vi "stationary_v5_parallel_dragonfly.vi"() -> ()   [LabVIEW 2020]
uses:
  CUSTOM_CONTROLS/Liquid_Handler_Enum_NSE.ctl
  CUSTOM_CONTROLS/Transport_to_Reactor_Enum_NSE.ctl
  CUSTOM_CONTROLS/Transport_to_Analysis_Enum_NSE.ctl
  CUSTOM_CONTROLS/Rinse_Vent_Reactor_Enum_NSE.ctl
  CUSTOM_CONTROLS/Rinse_Vent_Transfer_Lines_Enum_NSE - Copy.ctl
  CUSTOM_CONTROLS/Hardware_Initiation_Enum.ctl
  CUSTOM_CONTROLS/Reactor_Outer_Loop_Enum_NSE.ctl
  CUSTOM_CONTROLS/Reactors_Enum_NSE.ctl
  <vilib>/DAQmx/read.llb/DAQmx Read (Analog 1D Wfm NChan 1Samp).vi
  <vilib>/DAQmx/miscellaneous.llb/DAQmx Fill In Error Info.vi
  HARVARD/LIBRARY_CC/Harvard Apparatus PHD Ultra Series.lvlib
panel:
  out "Schedule - Reactor to Analysis":dbl[](array[numeric])=[2556.0, 3156.0]
  out "Schedule - Liquid Handler":dbl[](array[numeric])=[1.0, 601.0]
  out "IndexTemp":dbl
  out "InitializationExp":bool
  out "IndexAct":dbl
  out "NextAnaTimeTrigger":dbl
  out "Index_Ana_Rxn":dbl
  out "Converged?":bool
  in  "Array 3":dbl[](array[numeric])
  in  "Convergence criterion (area counts)":dbl=-10.0
  out "Full Results":dbl[](array[numeric])
  out "Optimum":dbl[](array[numeric])=[50.17167959931792, 8.535205424923882, 2.0, 1.0, 39.0]
  in  "Array 2":dbl[](array[numeric])
  in  "Array":dbl[][](array[numeric])
  out "Next batch":dbl[][](array[numeric])=[[75.0, 32.5, 2.0, 2.0], [75.0, 32.5, 2.0, 2.0]]
  out "Batch Results":dbl[](array[numeric])
  in  "Batch size":i32=4
  in  "Number of initial experiments":i32=5
  out "Product area":dbl
  out "schedule_reset":bool
  out "product_area":dbl=1000000000000000.0
  out "analysis_finished":bool
  out "Next analysis time":dbl=1000000000000000.0
  out "reactor_to_analysis_finished":bool
  out "loop_to_reactor_finished":bool
  out "rinse_reactor_finished":bool
  out "rinse_transfer_lines_finished":bool
  out "liquid_handler_finished":bool
  out "Temperature - Reactor 10":dbl format="%#_3g"
  out "Temperature - Reactor 9":dbl format="%#_3g"
  out "Temperature - Reactor 8":dbl format="%#_3g"
  out "Temperature - Reactor 7":dbl format="%#_3g"
  out "Temperature - Reactor 6":dbl format="%#_3g"
  out "Temperature - Reactor 5":dbl format="%#_3g"
  out "Temperature - Reactor 4":dbl format="%#_3g"
  out "Temperature - Reactor 3":dbl format="%#_3g"
  out "Temperature - Reactor 2":dbl format="%#_3g"
  out "Temperature - Reactor 1":dbl
  out "Relay output DAQ error":bool
  out "Slug preparation error":bool
  out "Reaction scheduling error":bool
  out "Slug composition error":bool
  out "Analog input DAQ error":bool
  out "Reagent table parsing error":bool
  out "Data processing output":string
  out "Analysis Error":errorcluster
  out "Performing Optimization?":bool
  out "Shutdown complete":bool
  out "reaction scheduling error":errorcluster
  out "Analog input 3":waveform(dbl)[](graph)=[{"t0"=timestamp(3735667643.042628 s since 1904-01-01), "dt"=1.0, "Y"=[1.5884301073614158], "attributes"=variant("NI_ChannelName"=variant(string "NI9205"), "NI_UnitDescription"=variant(string "Volts"))}, {"t0"=timestamp(3735667643.0426416 s since 1904-01-01), "dt"=1.0, "Y"=[2.7564288374126047], "attributes"=variant("NI_ChannelName"=variant(string "NI9206"), "NI_UnitDescription"=variant(string "Volts"))}, {"t0"=timestamp(3735667643.042656 s since 1904-01-01), "dt"=1.0, "Y"=[0.0967580440506516], "attributes"=variant("NI_ChannelName"=variant(string "NI9207"), "NI_UnitDescription"=variant(string "Volts"))}, {"t0"=timestamp(3735667643.04267 s since 1904-01-01), "dt"=1.0, "Y"=[2.2988144683350704], "attributes"=variant("NI_ChannelName"=variant(string "NI9208"), "NI_UnitDescription"=variant(string "Volts"))}, {"t0"=timestamp(3735667643.042684 s since 1904-01-01), "dt"=1.0, "Y"=[0.5635616561855846], "attributes"=variant("NI_ChannelName"=variant(string "NI9209"), "NI_UnitDescription"=variant(string "Volts"))}, {"t0"=timestamp(3735667643.042698 s since 1904-01-01), "dt"=1.0, "Y"=[2.4613101697855475], "attributes"=variant("NI_ChannelName"=variant(string "NI9210"), "NI_UnitDescription"=variant(string "Volts"))}, {"t0"=timestamp(3735667643.0427117 s since 1904-01-01), "dt"=1.0, "Y"=[0.03569936837913687], "attributes"=variant("NI_ChannelName"=variant(string "NI9211"), "NI_UnitDescription"=variant(string "Volts"))}, {"t0"=timestamp(3735667643.042726 s since 1904-01-01), "dt"=1.0, "Y"=[2.0184685330254633], "attributes"=variant("NI_ChannelName"=variant(string "NI9212"), "NI_UnitDescription"=variant(string "Volts"))}, {"t0"=timestamp(3735667643.04274 s since 1904-01-01), "dt"=1.0, "Y"=[-8.232623427411115e-05], "attributes"=variant("NI_ChannelName"=variant(string "NI9213"), "NI_UnitDescription"=variant(string "Volts"))}, {"t0"=timestamp(3735667643.0427537 s since 1904-01-01), "dt"=1.0, "Y"=[0.0002459461853764819], "attributes"=variant("NI_ChannelName"=variant(string "NI9214"), "NI_UnitDescription"=variant(string "Volts"))}, {"t0"=timestamp(3735667643.042768 s since 1904-01-01), "dt"=1.0, "Y"=[-8.232623427411115e-05], "attributes"=variant("NI_ChannelName"=variant(string "NI9215"), "NI_UnitDescription"=variant(string "Volts"))}, {"t0"=timestamp(3735667643.042782 s since 1904-01-01), "dt"=1.0, "Y"=[-0.00041059865377756494], "attributes"=variant("NI_ChannelName"=variant(string "NI9216"), "NI_UnitDescription"=variant(string "Volts"))}, {"t0"=timestamp(3735667643.0427957 s since 1904-01-01), "dt"=1.0, "Y"=[-8.232623427411115e-05], "attributes"=variant("NI_ChannelName"=variant(string "NI9217"), "NI_UnitDescription"=variant(string "Volts"))}, {"t0"=timestamp(3735667643.04281 s since 1904-01-01), "dt"=1.0, "Y"=[-0.02634411933170616], "attributes"=variant("NI_ChannelName"=variant(string "NI9218"), "NI_UnitDescription"=variant(string "Volts"))}, {"t0"=timestamp(3735667643.042824 s since 1904-01-01), "dt"=1.0, "Y"=[0.0074679394549679486], "attributes"=variant("NI_ChannelName"=variant(string "NI9219"), "NI_UnitDescription"=variant(string "Volts"))}, {"t0"=timestamp(3735667643.0428376 s since 1904-01-01), "dt"=1.0, "Y"=[-0.007960864261802411], "attributes"=variant("NI_ChannelName"=variant(string "NI9220"), "NI_UnitDescription"=variant(string "Volts"))}, {"t0"=timestamp(3735667643.042852 s since 1904-01-01), "dt"=1.0, "Y"=[4.807167858513361], "attributes"=variant("NI_ChannelName"=variant(string "NI9221"), "NI_UnitDescription"=variant(string "Volts"))}, {"t0"=timestamp(3735667643.0428658 s since 1904-01-01), "dt"=1.0, "Y"=[0.6298727473376983], "attributes"=variant("NI_ChannelName"=variant(string "NI9222"), "NI_UnitDescription"=variant(string "Volts"))}, {"t0"=timestamp(3735667643.04288 s since 1904-01-01), "dt"=1.0, "Y"=[2.1277837243918682], "attributes"=variant("NI_ChannelName"=variant(string "NI9223"), "NI_UnitDescription"=variant(string "Volts"))}, {"t0"=timestamp(3735667643.042894 s since 1904-01-01), "dt"=1.0, "Y"=[2.690773937081018], "attributes"=variant("NI_ChannelName"=variant(string "NI9224"), "NI_UnitDescription"=variant(string "Volts"))}, {"t0"=timestamp(3735667643.0429077 s since 1904-01-01), "dt"=1.0, "Y"=[2.492496222785915], "attributes"=variant("NI_ChannelName"=variant(string "NI9225"), "NI_UnitDescription"=variant(string "Volts"))}, {"t0"=timestamp(3735667643.042922 s since 1904-01-01), "dt"=1.0, "Y"=[2.2528561025872307], "attributes"=variant("NI_ChannelName"=variant(string "NI9226"), "NI_UnitDescription"=variant(string "Volts"))}]
  out "r10_start_time":dbl
  out "r10_temp_F":string
  out "r10_res_time":dbl
  out "r9_start_time":dbl
  out "r9_temp_F":string
  out "r9_res_time":dbl
  out "r8_start_time":dbl=4416.0
  out "r8_temp_F":string="32"
  out "r8_res_time":dbl=300.0
  out "r7_start_time":dbl
  out "r7_temp_F":string
  out "r7_res_time":dbl
  out "r6_start_time":dbl=3651.0
  out "r6_temp_F":string="32"
  out "r6_res_time":dbl=300.0
  out "r5_start_time":dbl=596.0
  out "r5_temp_F":string="95"
  out "r5_res_time":dbl=240.0
  out "r4_start_time":dbl=591.0
  out "r4_temp_F":string="95"
  out "r4_res_time":dbl=240.0
  out "r3_start_time":dbl=1356.0
  out "r3_temp_F":string="32"
  out "r3_res_time":dbl=300.0
  out "r2_start_time":dbl=591.0
  out "r2_temp_F":string="32"
  out "r2_res_time":dbl=300.0
  out "r1_res_time":dbl
  out "r1_temp_F":string
  out "r1_start_time":dbl
  out "Next start time - rinse reactor":dbl=986.0
  out "Relay Output DAQ Error":errorcluster
  out "Next start time - transport from reactor to analysis":dbl=836.0
  out "Next start time - rinse transfer lines":dbl=596.0
  out "Analog Input DAQ Error":errorcluster
  out "Next start time - transport from loop to reactor":dbl=481.0
  out "Master time [s]":dbl
  out "Next start time - liquid handler":dbl=1.0
  out "Slug preparation status":string="Preparing slug 1"
  out "Ready to start schedule timer":bool
  in  "Stop everything":bool
  in  "Pressurization confirmed":bool
  out "Hardware communication established":bool
  in  "Initiate hardware communication":bool=TRUE
  in  "Tab Control":T1(tab)=enum."Reactor Valves & Enablement"
  in  "LH Valve Position - Needle":string="4"
  in  "LH Valve Position - Reservoir":string="1"
  in  "LH Valve ID":i32
  in  "LH Valve COM":refnum<visa-resource-name>="COM27"
  in  "Carrier Pump COM":refnum<visa-resource-name>="COM12"
  in  "LH Pump COM":refnum<visa-resource-name>="COM58"
  in  "Carrier Pump ID":i32
  in  "LH Pump ID":i32
  in  "Rinse Well Number":i16=68
  in  "Rinse Rack Placement":i16=1
  in  "Rinse Rack Number":i16=209
  in  "Gilson Valve ID":i32=3 caption="Rinse Pump ID"
  in  "Gilson LH ID":i32=27 caption="Rinse Pump ID"
  in  "LH Injection Flow Rate (uL/min)":dbl=100.0 format="%.1f"
  in  "Gas Buffer Well Number":i16=69
  in  "Gas Buffer Rack Placement":i16=1
  in  "Gas Buffer Rack Number":i16=209
  in  "LH Withdraw\nFlow Rate (uL/min)":dbl=75.0 format="%.1f"
  in  "Gilson COM":refnum<visa-resource-name>="COM4"
  in  "Carrier Syringe Infuse\nRate (Rinse) (uL/min)":dbl=600.0 format="%.1f"
  in  "LH Syringe Diameter (mm)":dbl=4.75 format="%.3f"
  in  "Carrier Syringe Diameter (mm)":dbl=9.525 format="%.3f"
  in  "LH Syringe Max Vol (mL)":dbl=2.5 format="%.1f"
  in  "Carrier Syringe Max Vol (mL)":dbl=8.0 format="%.1f"
  in  "Carrier Valve COM":refnum<visa-resource-name>="COM50"
  in  "Carrier Valve ID":i32
  in  "Carrier Valve Position - System":string="A"
  in  "Carrier Valve Position - Refill":string="B"
  in  "Waste Valve COM":refnum<visa-resource-name>="COM5"
  in  "Waste Valve ID":i32=8
  in  "Waste Valve Position - System":string="B"
  in  "Waste Valve Position - Sample":string="A"
  in  "Online Pump COM":refnum<visa-resource-name>="COM36"
  in  "Online Pump ID":i32
  in  "Online Syringe Diameter (mm)":dbl=9.525
  in  "Online Syringe Max Vol (mL)":dbl=8.0
  in  "Reactor Selector Valve\n - Upstream - COM":refnum<visa-resource-name>="COM10"
  in  "Reactor Number":string="2"
  in  "Rinse Pump COM":refnum<visa-resource-name>="COM9"
  in  "Rinse Pump ID":i32
  in  "Rinse Syringe Diameter [mm]":dbl=9.525
  in  "Rinse Syringe Max Vol [mL]":dbl=8.0
  in  "Rinse Syringe Infuse Rate [uL/min]":dbl=500.0
  in  "Online Syringe Infuse Rate [uL/min]":dbl
  in  "Injection Valve COM":refnum<visa-resource-name>="COM18"
  in  "Injection Valve ID":i32
  in  "Injection Valve Position - System":string="A"
  in  "Injection Valve Position - LH Needle":string="B"
  in  "Analytical Valve COM":refnum<visa-resource-name>="COM33"
  in  "Analytical Valve ID":i32
  in  "Analytical Valve Position - System":string="A"
  in  "Analytical Valve Position - HPLC":string="B"
  in  "Reactor Selector Valve Downstream COM":refnum<visa-resource-name>="COM54"
  in  "Reactor Selector Valve Upstream ID":i32
  in  "Reactor Selector Valve Downstream ID":i32
  in  "Vent Valve COM":refnum<visa-resource-name>="COM31"
  in  "Vent Valve ID":i32
  in  "Vent Valve Position - System":string="A"
  in  "Vent Valve Position - Vent":string="B"
  in  "Carrier Syringe Infuse Rate\n(Droplet Transport) [uL/min]":dbl=450.0
  in  "Perfluorinated Oil Well Number":dbl=64.0
  in  "Analog Input (NI 9205) task out":refnum<k21>
  in  "Relay Output (NI 9482) task out":refnum<k21>
  in  "Agilent channel (relay output)":i32
  in  "Entrance Volume (sample loop to reactor phase sensor) [uL]":dbl=390.0 format="%.1f"
  in  "Exit Volume (reactor to sampling valve) [uL]":dbl=480.0 format="%.1f"
  in  "Number of Post-Slug Purges of LH Needle":dbl=2.0 format="%#_13g"
  in  "Number of Post-Slug Purges of LH Needle (Hovering)":dbl=2.0 format="%#_13g"
  in  "Number of Rinse Vial Dips of the LH Needle, Post-Slug":i32=2
  in  "Number of Rinse Vial Dips of the LH Needle, Between Stock Solutions":i32=1
  in  "Dip Time of LH Needle in Rinse Vial [s]":dbl=1.0 format="%#_13g"
  in  "Reaction Time Target [s]":dbl=300.0 format="%.1f"
  in  "Entrance Volume (reactor phase sensor to reactor center) [uL]":dbl=52.0
  in  "LH Buffer (upstream) [uL]":dbl=10.0 format="%.1f"
  in  "Number of Droplet Stirs":i32=10
  in  "LH Transfer Fluid Density (g/L)":dbl=889.0 format="%.1f"
  in  "LH Sample Loop Volume (uL)":dbl=40.0 format="%.1f"
  in  "Number of LH Needle Purges Prior to Droplet Prep":dbl=1.0 format="%#_13g"
  in  "LH Gas Buffer (downstream) [uL]":dbl=10.0
  in  "Transfer Volume from Needle to Sample Loop [uL]":dbl=310.0
  in  "Reactor Valve 10 Position - Reaction":string="B"
  in  "Reactor Valve 9 Position - Reaction":string="B"
  in  "Reactor Valve 8 Position - Reaction":string="B"
  in  "Reactor Valve 7 Position - Reaction":string="B"
  in  "Reactor Valve 6 Position - Reaction":string="B"
  in  "Reactor Valve 5 Position - Reaction":string="B"
  in  "Reactor Valve 4 Position - Reaction":string="B"
  in  "Reactor Valve 3 Position - Reaction":string="B"
  in  "Reactor Valve 2 Position - Reaction":string="B"
  in  "Reactor Valve 10 Position - System":string="A"
  in  "Reactor Valve 9 Position - System":string="A"
  in  "Reactor Valve 8 Position - System":string="A"
  in  "Reactor Valve 7 Position - System":string="A"
  in  "Reactor Valve 6 Position - System":string="A"
  in  "Reactor Valve 5 Position - System":string="A"
  in  "Reactor Valve 4 Position - System":string="A"
  in  "Reactor Valve 3 Position - System":string="A"
  in  "Reactor Valve 2 Position - System":string="A"
  in  "Reactor Valve 10 ID":dbl
  in  "Reactor Valve 9 ID":dbl
  in  "Reactor Valve 8 ID":dbl
  in  "Reactor Valve 7 ID":dbl
  in  "Reactor Valve 6 ID":dbl
  in  "Reactor Valve 5 ID":dbl
  in  "Reactor Valve 4 ID":dbl
  in  "Reactor Valve 3 ID":dbl
  in  "Reactor Valve 2 ID":i32
  in  "Reactor Valve 10 COM":refnum<visa-resource-name>="COM51"
  in  "Reactor Valve 9 COM":refnum<visa-resource-name>="COM30"
  in  "Reactor Valve 8 COM":refnum<visa-resource-name>="COM56"
  in  "Reactor Valve 7 COM":refnum<visa-resource-name>="COM48"
  in  "Reactor Valve 6 COM":refnum<visa-resource-name>="COM53"
  in  "Reactor Valve 5 COM":refnum<visa-resource-name>="COM37"
  in  "Reactor Valve 4 COM":refnum<visa-resource-name>="COM49"
  in  "Reactor Valve 3 COM":refnum<visa-resource-name>="COM24"
  in  "Reactor Valve 2 COM":refnum<visa-resource-name>="COM5"
  in  "Reactor Valve 1 ID":i32
  in  "Reactor Valve 1 Position - System":string="A"
  in  "Reactor Valve 1 Position - Reaction":string="B"
  in  "Reactor Valve 1 COM":refnum<visa-resource-name>="COM26"
  in  "Reactor 1 enabled?":bool
  in  "Reactor 2 enabled?":bool
  in  "Reactor 3 enabled?":bool
  in  "Reactor 4 enabled?":bool=TRUE
  in  "Reactor 5 enabled?":bool=TRUE
  in  "Reactor 6 enabled?":bool=TRUE
  in  "Reactor 7 enabled?":bool
  in  "Reactor 8 enabled?":bool=TRUE
  in  "Reactor 9 enabled?":bool
  in  "Reactor 10 enabled?":bool
  out "Temperature Control Error - Reactor 10":errorcluster
  out "Temperature Control Error - Reactor 9":errorcluster
  out "Temperature Control Error - Reactor 8":errorcluster
  out "Temperature Control Error - Reactor 7":errorcluster
  out "Temperature Control Error - Reactor 6":errorcluster
  out "Temperature Control Error - Reactor 5":errorcluster
  out "Temperature Control Error - Reactor 4":errorcluster
  out "Temperature Control Error - Reactor 3":errorcluster
  out "Temperature Control Error - Reactor 2":errorcluster
  out "Temperature Control Error - Reactor 1":errorcluster
  in  "Watlow Instance - Reactor 10":dbl=1.0
  in  "Watlow Zone - Reactor 10":dbl=1.0
  in  "Watlow Instance - Reactor 9":dbl=9.0
  in  "Watlow Zone - Reactor 9":dbl=1.0
  in  "Watlow Instance - Reactor 8":dbl=8.0
  in  "Watlow Zone - Reactor 8":dbl=1.0
  in  "Watlow Instance - Reactor 7":dbl=12.0
  in  "Watlow Zone - Reactor 7":dbl=1.0
  in  "Watlow Instance - Reactor 6":dbl=11.0
  in  "Watlow Zone - Reactor 6":dbl=1.0
  in  "Watlow Instance - Reactor 5":dbl=10.0
  in  "Watlow Zone - Reactor 5":dbl=1.0
  in  "Watlow Instance - Reactor 4":dbl=4.0
  in  "Watlow Zone - Reactor 4":dbl=1.0
  in  "Watlow Instance - Reactor 3":dbl=7.0
  in  "Watlow Zone - Reactor 3":dbl=1.0
  in  "Watlow Instance - Reactor 2":dbl=2.0
  in  "Watlow Zone - Reactor 2":dbl=1.0
  in  "Watlow Instance - Reactor 1":dbl=5.0
  in  "Watlow Zone - Reactor 1":dbl=1.0
  out "r1_done":bool
  out "r2_done":bool
  out "r3_done":bool
  out "r4_done":bool
  out "r5_done":bool
  out "r6_done":bool
  out "r7_done":bool
  out "r8_done":bool
  out "r9_done":bool
  out "r10_done":bool
  in  "Watlow COM":refnum<visa-resource-name>="COM13"
  in  "Vent time [s]":dbl=40.0
  in  "Analytical method length [s]":dbl=820.0
  in  "Transport time - reactor to analysis [s]":dbl=150.0
  in  "Rinse and vent time - transfer lines plus one reactor [s]":dbl=230.0
  in  "Rinse and vent time - transfer lines only [s]":dbl=175.0
  in  "Transport time - droplet to reactor [s]":dbl=145.0
  in  "Liquid handler preparation time [s]":dbl=740.0
  out "Schedule - Liquid Handler to Reactor":dbl[](array[numeric])=[481.0, 1081.0]
  out "Schedule - Rinse Transfer Lines":dbl[](array[numeric])=[606.0, 1206.0]
  out "Schedule - Rinse Reactor":dbl[](array[numeric])=[2696.0, 3296.0]
  out "Schedule - Analysis":dbl[](array[numeric])=[2696.0, 3296.0]
  out "Schedule - Reactors":dbl[][](array[numeric])=[[0.0, 0.0], [606.0, 0.0], [0.0, 1206.0], [0.0, 0.0], [0.0, 0.0], [0.0, 0.0], [0.0, 0.0], [0.0, 0.0], [0.0, 0.0], [0.0, 0.0]]
  out "Reaction number - transport to reactor":dbl
  out "Reaction number - rinse transfer lines":dbl
  out "Reaction number - transport from reactor to analysis":dbl
  out "Reactor assignment - transport from loop to reactor":string
  out "Reactor assignment - transport from reactor to analysis":string="5"
  out "Reaction number - rinse reactor":dbl
  in  "Transfer lines plus reactor volume - for rinse/vent operation":dbl=1300.0
  in  "Transfer lines volume - for rinse/vent operation [uL]":dbl=1100.0
  in  "Volume between rinse droplets [uL]":dbl=15.0
  in  "Number of rinse droplets":i32=3
  in  "Rinse droplet volume [uL]":dbl=20.0
  out "Phase Sensor Reading - Injection Valve [V]":dbl=2.690773937081018
  out "Phase Sensor Reading - Reactor 1":dbl=1.5884301073614158
  out "Phase Sensor Reading - Reactor 2":dbl=2.7564288374126047
  out "Phase Sensor Reading - Reactor 3":dbl=0.0967580440506516
  out "Phase Sensor Reading - Reactor 4":dbl=2.2988144683350704
  out "Phase Sensor Reading - Reactor 5":dbl=0.5635616561855846
  out "Phase Sensor Reading - Reactor 6":dbl=2.4613101697855475
  out "Phase Sensor Reading - Reactor 7":dbl=0.03569936837913687
  out "Phase Sensor Reading - Reactor 8":dbl=2.0184685330254633
  out "Phase Sensor Reading - Reactor 9":dbl=4.807167858513361
  out "Phase Sensor Reading - Reactor 10":dbl=0.6298727473376983
  in  "Phase Sensor Liquid Threshold - Reactor 1":dbl=3.5
  in  "Phase Sensor Liquid Threshold - Reactor 2":dbl=3.5
  in  "Phase Sensor Liquid Threshold - Reactor 3":dbl=3.5
  in  "Phase Sensor Liquid Threshold - Reactor 4":dbl=1.0
  in  "Phase Sensor Liquid Threshold - Reactor 5":dbl=3.5
  in  "Phase Sensor Liquid Threshold - Reactor 6":dbl=3.5
  in  "Phase Sensor Liquid Threshold - Reactor 7":dbl=1.0
  in  "Phase Sensor Liquid Threshold - Reactor 8":dbl=3.5
  in  "Phase Sensor Liquid Threshold - Reactor 9":dbl=3.5
  in  "Phase Sensor Liquid Threshold - Reactor 10":dbl=3.5
  in  "Phase Sensor Liquid Threshold - Injection Valve":dbl=1.0
  out "Phase Sensor Detection - Injection Valve":bool
  out "Phase Sensor Reading Start - Injection Valve [s]":dbl=1000000000000000.0
  in  "Phase Sensor - Injection Valve - Minimum Gas Length [s]":dbl=3.0
  out "Phase Sensor Reading - Analytical Valve":dbl=0.6298727473376983
  in  "Phase Sensor Liquid Threshold - Analytical Valve":dbl=3.5
  out "Phase Sensor Reading Start - Reactor [s]":dbl=1000000000000000.0
  in  "Phase Sensor - Reactor - Minimum Liquid Length [s]":dbl=3.0
  out "Phase Sensor Detection - Reactor":bool
  out "Phase Sensor Detection - Analytical Valve":bool
  out "Phase Sensor Reading Start - Analytical Valve [s]":dbl=1000000000000000.0
  in  "Phase Sensor - Analytical Valve - Minimum Liquid Length [s]":dbl=3.0
  in  "python path":path=path "C:/Users/Parallel Oscillator/PycharmProjects/oscillatorArduino/interface_3.py"
  in  "python Peltier fn name":string="RunPeltier1"
  in  "Peltier value":dbl=255.0
  in  "LED value":dbl=128.0
  in  "Data Analysis File (root)":string="C:\\Users\\Admin\\Desktop\\log\\ana_path"
  in  "Path for HPLC Chromatograms":string="C:\\Chem32\\1\\Data\\"
  in  "ChemStation Name":string="hpcore1716"
  in  "Name of HPLC processing function":string="TS_process_coupling_product_area"
  in  "Data pattern":string="Test_Blank_FullReportF*"
  in  "Template reagent file path":path=path "C:/Users/Parallel Oscillator/Documents/Parallel LabVIEW/Input/TS_Reagent_Table_Dragonfly_2.xlsx"
  out "error out":errorcluster
  in  "Dragonfly python path":path=path "C:/Users/Parallel Oscillator/PycharmProjects/dragonfly_V1/dragonfly_V5.py"
  in  "Initialization function":string="define_initial_experiments"
  in  "Refinement function":string="refine"
  in  "Summary report function":string="report"
  out "Slug Composition Error":errorcluster
  out "Reagent Table Parsing Error":errorcluster
  out "Slug Preparation Error":errorcluster
  # "Error Tracking"
  # "Main Updates"
  # "Temperature Tracking"
  # "Dragonfly Optimization"
  # "Parameters & Control"
  # "Algorithm Output"
  # "Results"
  # "Schedule"
  # "Pumps and Valves (excluding reactor valves - see next tab)"
  # "Liquid Handler & Vial Placement"
  # "cDAQ"
  # "I/O --> DAQmx Name Controls --> DAQmx Task Name"
  # "Droplet Preparation"
  # "Transport Volumes"
  # "Carryover Minimization"
  # "Buttons for manually enabling/\ndisabling each reactor"
  # "The values in this tab define the lengths of operations, in seconds, that the scheduler uses to define the schedule for the\nreaction sequence"
  # "Same signal temporarily wired\nto R10 and analytical valve readings\ndue to hardware problem on MIT side"
  # "TODO: control board software not integrated with this VI yet"
  # "Type \"print _DDENAME$\" in OpenLab to obtain the Application Name"
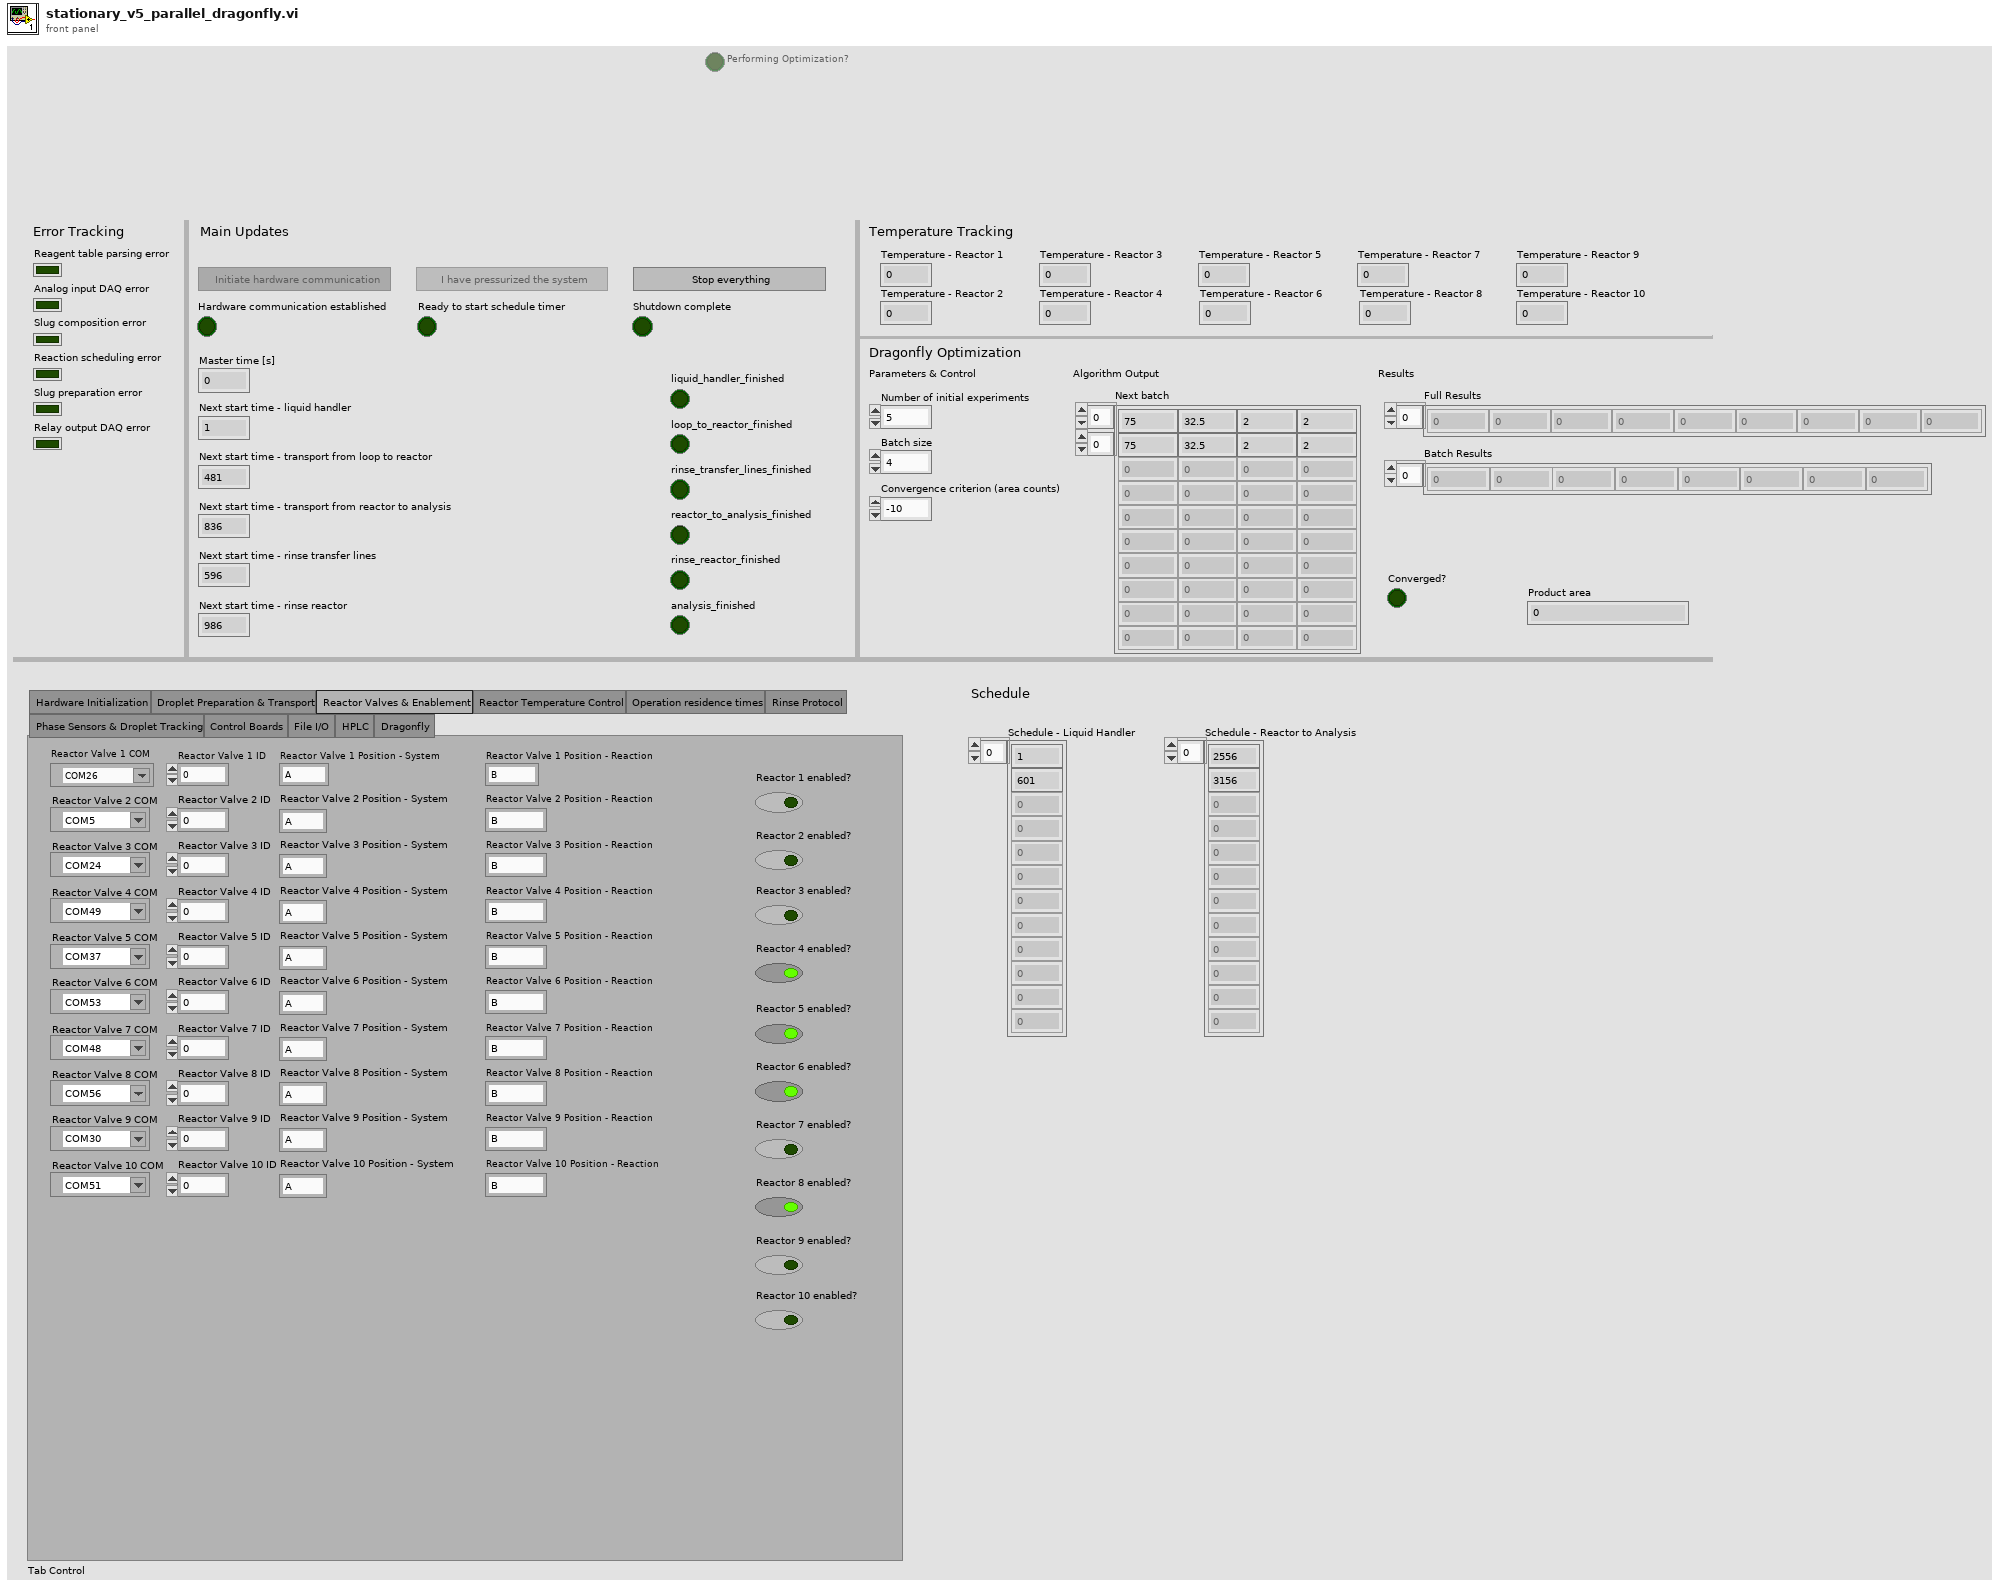
[diagram p1: front panel]
types:
  T1 = enum32{"Hardware Initialization", "Droplet Preparation & Transport", "Reactor Valves & Enablement", "Reactor Temperature Control", "Operation residence times", "Rinse Protocol", "Phase Sensors & Droplet Tracking", "Control Boards", "File I/O", "HPLC", "Dragonfly"}
  T2 = typedef "Hardware_Initiation_Enum.ctl" = enum16{"Initialize parameters", "Wait to begin hardware initialization", "Initialize hardware", "Wait for user to confirm pressurization", "Pressurize everything", "Running"}
  T3 = typedef "Rinse_Vent_Transfer_Lines_Enum_NSE - Copy.ctl" = enum16{"Waiting for hardware initialization", "Rinse and vent transfer lines sequence is idle", "Rinse and vent transfer lines in progress"}
  T4 = typedef "Rinse_Vent_Reactor_Enum_NSE.ctl" = enum16{"Waiting for hardware initialization", "Rinse and vent reactor sequence is idle", "Rinse and vent reactor in progress"}
  T5 = typedef "Transport_to_Analysis_Enum_NSE.ctl" = enum16{"Waiting for hardware initialization", "Transport sequence is idle", "Transport in progress"}
  T6 = typedef "Transport_to_Reactor_Enum_NSE.ctl" = enum16{"Waiting for hardware initialization", "Transport sequence is idle", "Transport in progress"}
  T7 = typedef "Liquid_Handler_Enum_NSE.ctl" = enum16{"Waiting for hardware initialization", "Liquid handler is idle", "Liquid handler is preparing a droplet"}
  T8 = enum16{"Enabled", "Disabled", "Disabled and Grayed Out"}
  T9 = typedef "Reactor_Outer_Loop_Enum_NSE.ctl" = enum16{"Waiting for hardware initialization", "Running"}
  T10 = typedef "Reactors_Enum_NSE.ctl" = enum16{"Getting next assignment", "Running", "Done"}
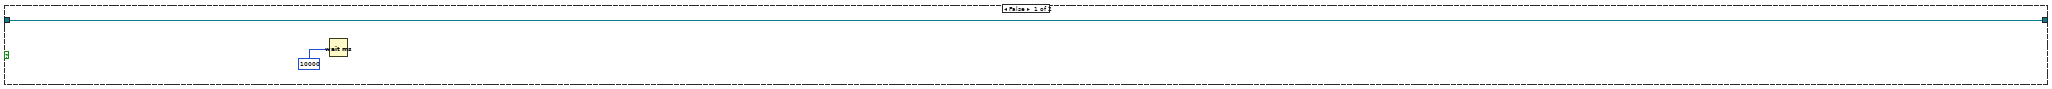
[diagram p2: hidden frame]
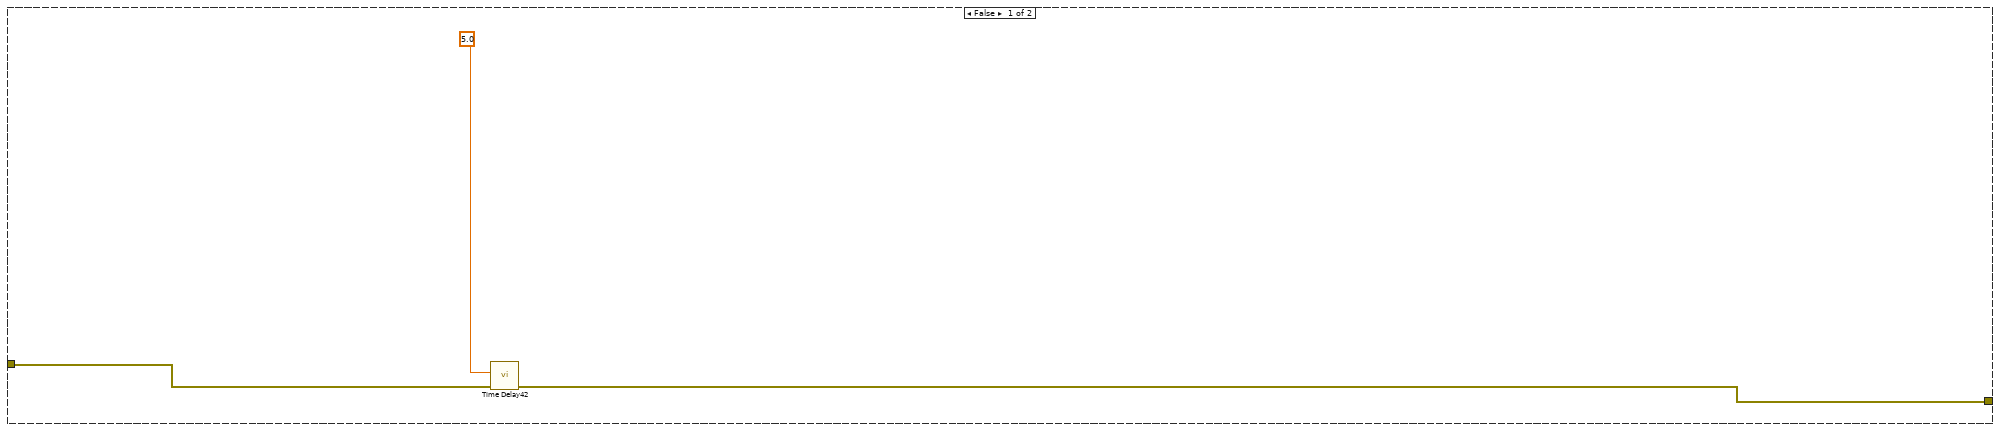
[diagram p4: hidden frame]
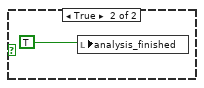
[diagram p5: hidden frame]
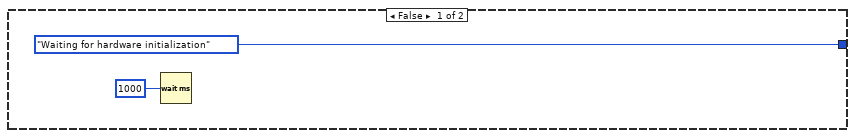
[diagram p7: hidden frame]
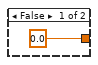
[diagram p8: hidden frame]
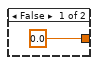
[diagram p9: hidden frame]
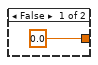
[diagram p10: hidden frame]
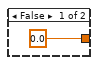
[diagram p11: hidden frame]
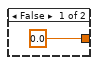
[diagram p12: hidden frame]
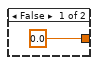
[diagram p13: hidden frame]
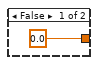
[diagram p14: hidden frame]
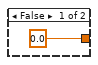
[diagram p15: hidden frame]
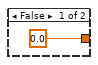
[diagram p16: hidden frame]
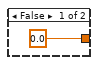
[diagram p17: hidden frame]
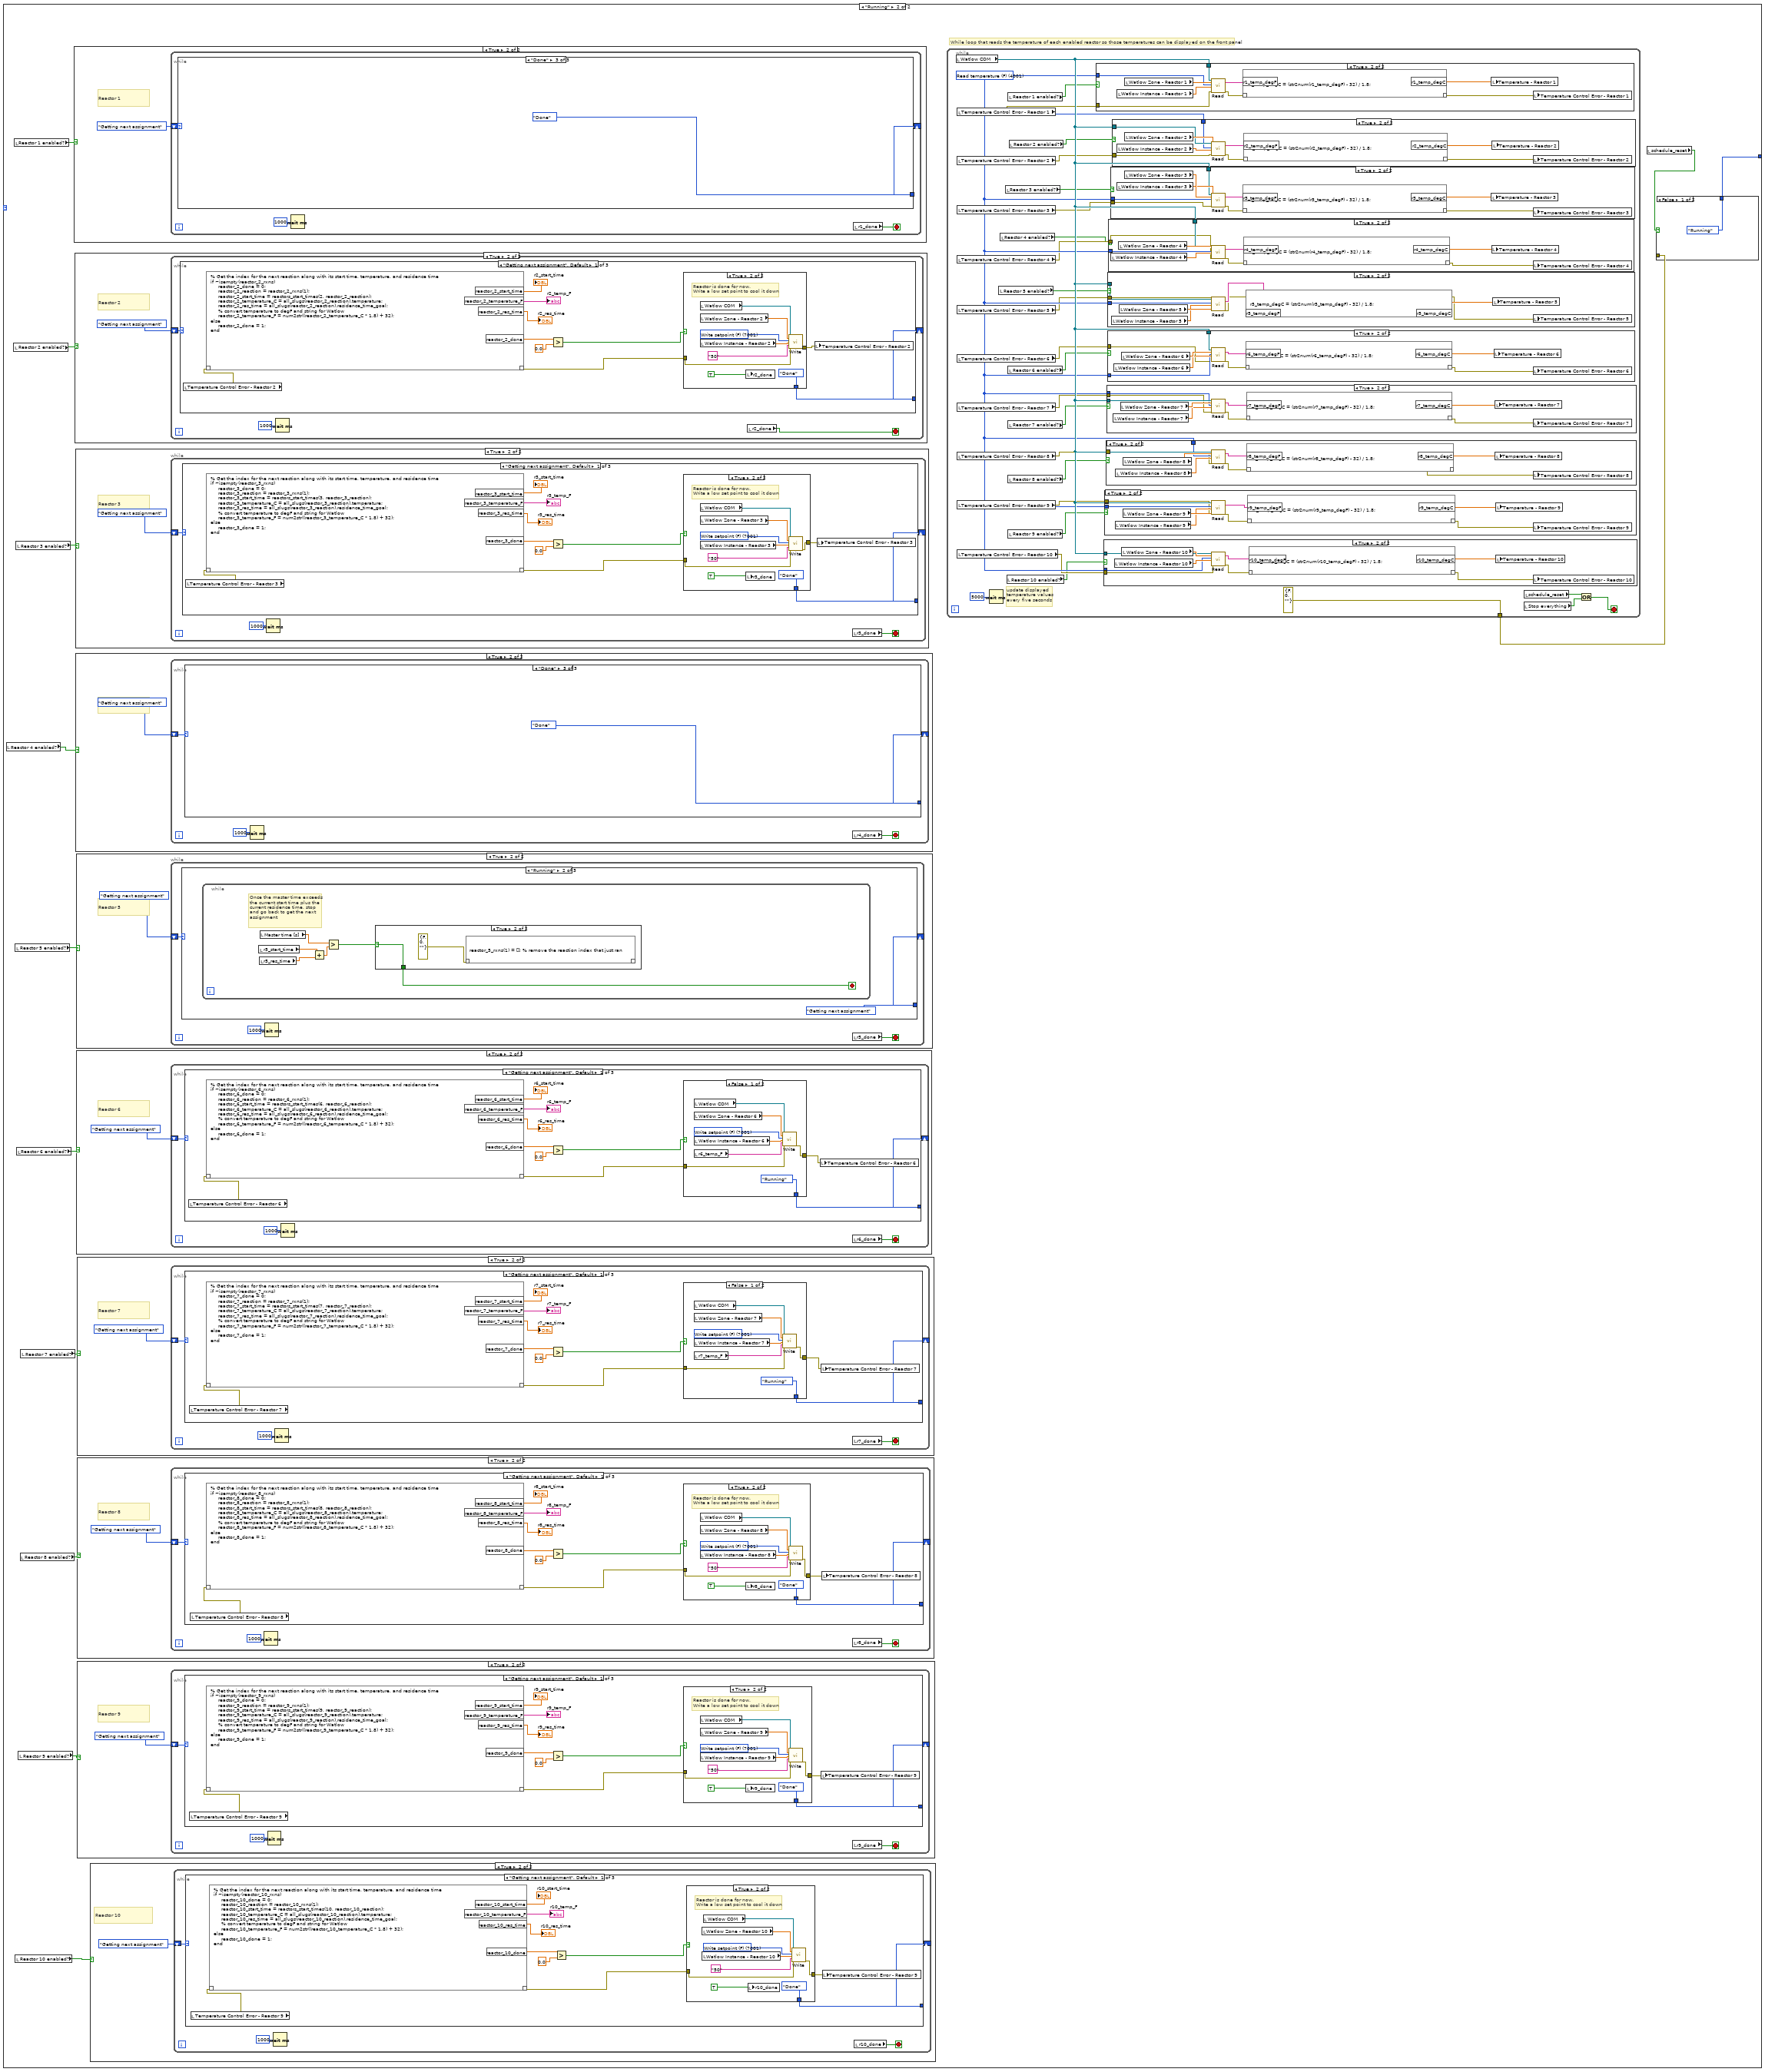
[diagram p18: hidden frame]
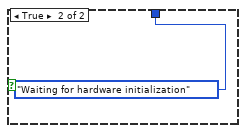
[diagram p19: hidden frame]
diagram:
  # "LIQUID HANDLER LOOP"
  # "Shutdown sequence"
  # "TODO: ADD CODE HERE TO DEAL WITH CASES WHERE THE\nPREP STEP FAILS AND THE SCHEDULE HAS TO BE RESET. IF\nTHE SCHEDULE GETS RESET, PRUDENT TO UPDATE THE \"NEXT\nSTART TIME\" VALUE. BUT DON'T NEED TO, BECAUSE THE\nCODE WON'T TRIGGER THE TRANSPORT UNTIL IT SEES THE\nDROPLET AT THE INJECTION VALVE ANYWAY"
  # "TODO: Calculate expected transport time\nto identify failure / lost droplet - use \ncalculated time in the while loop to the right ... to stop it EITHER when the PS detects the droplet OR when the droplet is suspected to be lost"
  # "Updating the master time and sensors"
  # "Rinse and vent sequences"
  # "Transport Sequence - Reactor to Analysis"
  # "Transport Sequence - Injection Valve Sample Loop to Reactor"
  # "Liquid Handler Loop"
  n1 = Open Python Session(python version="3.9", 3:errorcluster {"status"=FALSE, "code"=0, "source"=""} ("error constant")) -> (session out=w3:refnum<k35>, error out=w6:errorcluster)  [unwired: 1 in]
  n2 = while {
    shift-right: [w22] -> _
    shift-left: Hardware_Initiation_Enum."Initialize parameters" ("Enum") -> [w23]
    tunnel: errorcluster {"status"=FALSE, "code"=0, "source"=""} ("error constant") -> [w20]
    tunnel: w6 -> [w18]
    shift-right: [w19] -> _
    shift-left: w3 -> [w17]
    stop <- w21 stop-if-true
    n3 = case shown="\"Initialize parameters\"" w23 {
      tunnel: [Hardware_Initiation_Enum."Wait to begin hardware initialization" ("Enum") w118 Hardware_Initiation_Enum."Wait for user to confirm pressurization" ("Enum") w329 Hardware_Initiation_Enum."Running" ("Enum") w640] -> w22
      tunnel: w20 -> [_ _ _ _ _ _]
      tunnel: [w32 w115 w133 w327 w334 w638] -> w19
      tunnel: w17 -> [w31 w115 w133 w327 w334 w638]
      tunnel: w18 -> [w30 _ _ _ _ _]
      frame "Initialize parameters" {
        w24 = 1000.0
        w41 = 0.0
        w44 = 1000000000000000.0
        w48 = errorcluster {"status"=FALSE, "code"=0, "source"=""} ("error constant")
        w27 = errorcluster {"status"=FALSE, "code"=0, "source"=""} ("error constant")
        w42 = 0.0
        w45 = FALSE
        # "Reset error values"
        # "Perform initial scheduling operation"
        # "Load reagent table and parse initial slugs"
        n4 = local read "Liquid handler preparation time [s]"() -> (w90:dbl)
        n5 = local read "Transport time - droplet to reactor [s]"() -> (w89:dbl)
        n6 = local read "Rinse and vent time - transfer lines only [s]"() -> (w88:dbl)
        n7 = local read "Rinse and vent time - transfer lines plus one reactor [s]"() -> (w87:dbl)
        n8 = local read "Transport time - reactor to analysis [s]"() -> (w86:dbl)
        n9 = local read "Analytical method length [s]"() -> (w85:dbl)
        n10 = local read "Reactor 1 enabled?"() -> (w67:bool)
        n11 = local read "Reactor 2 enabled?"() -> (w66:bool)
        n12 = local read "Reactor 3 enabled?"() -> (w65:bool)
        n13 = local read "Reactor 4 enabled?"() -> (w64:bool)
        n14 = local read "Reactor 5 enabled?"() -> (w63:bool)
        n15 = local read "Reactor 6 enabled?"() -> (w62:bool)
        n16 = local read "Reactor 7 enabled?"() -> (w61:bool)
        n17 = local read "Reactor 8 enabled?"() -> (w60:bool)
        n18 = local read "Reactor 9 enabled?"() -> (w59:bool)
        n19 = local read "Reactor 10 enabled?"() -> (w58:bool)
        n20 = local write "Master time [s]"(w42) -> ()
        n21 = local write "Reaction number - rinse reactor"(w42) -> ()
        n22 = local write "Reaction number - rinse transfer lines"(w42) -> ()
        n23 = local write "Reaction number - transport from reactor to analysis"(w42) -> ()
        n24 = local write "Reaction number - transport to reactor"(w42) -> ()
        n25 = property on="Initiate hardware communication" class="Bool (strict)"(error in=w48, "DisabledEnum"=T8."Disabled and Grayed Out") -> ()  [unwired: 1 in, 2 out]
        n26 = local write "Initiate hardware communication"(w45) -> ()
        n27 = local write "Pressurization confirmed"(w45) -> ()
        n28 = local write "Hardware communication established"(w45) -> ()
        n29 = local write "Ready to start schedule timer"(w45) -> ()
        n30 = local write "Phase Sensor Detection - Injection Valve"(w45) -> ()
        n31 = local write "Stop everything"(w45) -> ()
        n32 = local write "Phase Sensor Detection - Reactor"(w45) -> ()
        n33 = local write "Phase Sensor Detection - Analytical Valve"(w45) -> ()
        n34 = local write "Shutdown complete"(w45) -> ()
        n35 = property on="Pressurization confirmed" class="Bool (strict)"(error in=w48, "DisabledEnum"=T8."Disabled and Grayed Out") -> ()  [unwired: 1 in, 2 out]
        n36 = local read "Rinse and vent time - transfer lines plus one reactor [s]"() -> (w75:dbl)
        n37 = local read "Rinse and vent time - transfer lines only [s]"() -> (w76:dbl)
        n38 = local write "Analysis Error"(w27) -> ()
        n39 = case shown="True" w67 {
          tunnel: [0.0 1.0] -> w68
          frame False {
          }
          frame True {
          }
        }
        n40 = case shown="True" w66 {
          tunnel: [0.0 1.0] -> w57
          frame False {
          }
          frame True {
          }
        }
        n41 = case shown="True" w65 {
          tunnel: [0.0 1.0] -> w56
          frame False {
          }
          frame True {
          }
        }
        n42 = case shown="True" w64 {
          tunnel: [0.0 1.0] -> w55
          frame False {
          }
          frame True {
          }
        }
        n43 = case shown="True" w63 {
          tunnel: [0.0 1.0] -> w54
          frame False {
          }
          frame True {
          }
        }
        n44 = case shown="True" w62 {
          tunnel: [0.0 1.0] -> w53
          frame False {
          }
          frame True {
          }
        }
        n45 = case shown="True" w61 {
          tunnel: [0.0 1.0] -> w52
          frame False {
          }
          frame True {
          }
        }
        n46 = case shown="True" w60 {
          tunnel: [0.0 1.0] -> w51
          frame False {
          }
          frame True {
          }
        }
        n47 = case shown="True" w59 {
          tunnel: [0.0 1.0] -> w50
          frame False {
          }
          frame True {
          }
        }
        n48 = case shown="True" w58 {
          tunnel: [0.0 1.0] -> w49
          frame False {
          }
          frame True {
          }
        }
        n49 = local write "Reagent Table Parsing Error"(w27) -> ()
        n50 = call "Time Delay79"("error in (no error)"=w27, "Delay Time (s)"=3.0) -> ("error out"=w26:errorcluster)  [unwired: 9 in]
        n51 = local write "Product area"(w42) -> ()
        n52 = local write "liquid_handler_finished"(w45) -> ()
        n53 = local write "reactor_to_analysis_finished"(w45) -> ()
        n54 = local write "loop_to_reactor_finished"(w45) -> ()
        n55 = local write "rinse_reactor_finished"(w45) -> ()
        n56 = local write "rinse_transfer_lines_finished"(w45) -> ()
        n57 = local write "analysis_finished"(w45) -> ()
        n58 = local read "Vent time [s]"() -> (w77:dbl)
        n59 = local read "Vent time [s]"() -> (w74:dbl)
        n60 = local write "Converged?"(w45) -> ()
        n61 = local write "Data processing output"("") -> ()
        n62 = local write "Next analysis time"(w44) -> ()
        n63 = Greater?(x=w77, y=w76) -> (0:w73:bool)
        n64 = Greater?(x=w74, y=w75) -> (0:w72:bool)
        n65 = Or(x=w73, y=w72) -> (x .or. y?=w71:bool)
        n66 = local read "Array 3"() -> (w29:dbl[])
        n67 = local read "Number of initial experiments"() -> (w39:i32)
        n68 = local write "Temperature - Reactor 1"(w41) -> ()
        n69 = local write "Temperature - Reactor 10"(w41) -> ()
        n70 = local write "Temperature - Reactor 2"(w41) -> ()
        n71 = local write "Temperature - Reactor 9"(w41) -> ()
        n72 = local write "Temperature - Reactor 8"(w41) -> ()
        n73 = local write "Temperature - Reactor 7"(w41) -> ()
        n74 = local write "Temperature - Reactor 6"(w41) -> ()
        n75 = local write "Temperature - Reactor 5"(w41) -> ()
        n76 = local write "Temperature - Reactor 4"(w41) -> ()
        n77 = case shown="True" w71 {
          tunnel: w26 -> [_ w114]
          frame False {
          }
          frame True {
            n78 = call "Display Message to User2"("error in (no error)"=w114) -> ()  [unwired: 9 in, 2 out]
            n79 = local write "Stop everything"(TRUE) -> ()
          }
        }
        n80 = local write "Temperature - Reactor 3"(w41) -> ()
        n81 = local read "Dragonfly python path"() -> (w36:path)
        n82 = local write "Batch Results"(w29) -> ()
        n83 = local write "Full Results"(w29) -> ()
        n84 = local read "Batch size"() -> (w38:i32)
        n85 = local read "Initialization function"() -> (w40:string)
        n86 = node(w31, w36, w40, w30, "Array", w39, w38) -> (w32:refnum<k35>, w35:dbl[][])  [unwired: 2 in, 3 out]
        n87 = local write "InitializationExp"(TRUE) -> ()
        n88 = local write "Next batch"(w35) -> ()
        n89 = local write "NextAnaTimeTrigger"(w24) -> ()
        n90 = local write "IndexAct"(w24) -> ()
        n91 = Path To String(path="Template reagent file path") -> (string=w33:string)
        n92 = script code="%clear all\n%fclose('all');\n\n% Define reagent table based on initialization experiments from Dragonfly\niteration = 0;\nreagent_table_path = nse_dragonfly_to_reagent_table(template_file_path, iteration, next_batch);\n\n\n% reagent_table lists all reagents in the system\nreagent_table = ReagentTable();\nreagent_table.load_from_file(reagent_table_path);\n\nanalyte_table = AnalyteTable();\nanalyte_table.load_from_file(reagent_table_path);\n\n% slug_tracker is the matrix of slug information\n% index identifies the information contained in each column of slug_tracker \n\nN_reactors = 0;\nenabled_reactors_list = [];\nif r1_enabled\n    enabled_reactors_list = [enabled_reactors_list 1];\n    N_reactors = N_reactors + 1;\nend\nif r2_enabled\n    enabled_reactors_list = [enabled_reactors_list 2];\n    N_reactors = N_reactors + 1;\nend\nif r3_enabled\n    enabled_reactors_list = [enabled_reactors_list 3];\n    N_reactors = N_reactors + 1;\nend\nif r4_enabled\n    enabled_reactors_list = [enabled_reactors_list 4];\n    N_reactors = N_reactors + 1;\nend\nif r5_enabled\n    enabled_reactors_list = [enabled_reactors_list 5];\n    N_reactors = N_reactors + 1;\nend\nif r6_enabled\n    enabled_reactors_list = [enabled_reactors_list 6];\n    N_reactors = N_reactors + 1;\nend\nif r7_enabled\n    enabled_reactors_list = [enabled_reactors_list 7];\n    N_reactors = N_reactors + 1;\nend\nif r8_enabled\n    enabled_reactors_list = [enabled_reactors_list 8];\n    N_reactors = N_reactors + 1;\nend\nif r9_enabled\n    enabled_reactors_list = [enabled_reactors_list 9];\n    N_reactors = N_reactors + 1;\nend\nif r10_enabled\n    enabled_reactors_list = [enabled_reactors_list 10];\n    N_reactors = N_reactors + 1;\nend\n[all_slugs] = nse_parse_initial_slugs_parallel_v7(reagent_table_path, N_reactors, enabled_reactors_list); %for Dragonfly: unsorted version!!!!\n[liquid_handler_start_times, loop_to_reactor_start_times, rinse_transfer_lines_start_times, reactor_to_analysis_start_times, rinse_reactor_start_times, analysis_start_times, reactors_start_times] = nse_scheduler_v3(all_slugs, 10, tau_prep, tau_loop_to_reactor, tau_rinse_vent_transfer_lines, tau_rinse_vent_reactor, tau_reactor_to_analysis, tau_analysis)\nrinse_transfer_lines_last_rxn = 0;\nrinse_reactor_last_rxn = 0;\n% wait until everything is initialized and pressurized before starting the clock\n\n% Define initial start time for liquid handler\nliquid_handler_next_start_time = liquid_handler_start_times(1);\n\nrinse_slugs = [];"("??"=w26, "tau_prep"=w90, "tau_loop_to_reactor"=w89, "tau_rinse_vent_transfer_lines"=w88, "tau_rinse_vent_reactor"=w87, "tau_reactor_to_analysis"=w86, "tau_analysis"=w85, "r1_enabled"=w68, "r2_enabled"=w57, "r3_enabled"=w56, "r4_enabled"=w55, "r5_enabled"=w54, "r6_enabled"=w53, "r7_enabled"=w52, "r8_enabled"=w51, "r9_enabled"=w50, "r10_enabled"=w49, "next_batch"=w35, "template_file_path"=w33) -> ("??"=w47:errorcluster, "liquid_handler_start_times"=→"Schedule - Liquid Handler":dbl[], "loop_to_reactor_start_times"=→"Schedule - Liquid Handler to Reactor":dbl[], "rinse_transfer_lines_start_times"=→"Schedule - Rinse Transfer Lines":dbl[], "reactor_to_analysis_start_times"=→"Schedule - Reactor to Analysis":dbl[], "rinse_reactor_start_times"=→"Schedule - Rinse Reactor":dbl[], "analysis_start_times"=→"Schedule - Analysis":dbl[], "reactors_start_times"=→"Schedule - Reactors":dbl[][], "liquid_handler_next_start_time"=w78:dbl)
        "Reagent Table Parsing Error" <- w47
        n93 = local write "Next start time - liquid handler"(w78) -> ()
        n94 = Unbundle By Name(w47) -> ("status"=→"Reagent table parsing error":bool)
        "Analog Input DAQ Error" <- w27
        "product_area" <- w44
        "schedule_reset" <- w45
      }
      frame "Wait to begin hardware initialization" {
        n95 = property on="Initiate hardware communication" class="Bool (strict)"(error in=errorcluster {"status"=FALSE, "code"=0, "source"=""} ("error constant"), "DisabledEnum"=T8."Enabled") -> ()  [unwired: 1 in, 2 out]
        n96 = local read "Initiate hardware communication"() -> (w119:bool)
        n97 = case shown="True" w119 {
          tunnel: [Hardware_Initiation_Enum."Wait to begin hardware initialization" ("Enum") Hardware_Initiation_Enum."Initialize hardware" ("Enum")] -> w118
          frame False {
            n98 = Wait (ms)(milliseconds to wait=100) -> ()  [unwired: 1 out]
          }
          frame True {
            # "The user has confirmed that we are ready to proceed with\nhardware initialization. Disable the \"initiate hardware\ncommunication\" button and proceed to the next case in\nthe sequence: the hardware initialization step."
            n99 = property on="Initiate hardware communication" class="Bool (strict)"("DisabledEnum"=T8."Disabled and Grayed Out") -> ()  [unwired: 2 in, 2 out]
          }
        }
      }
      frame "Initialize hardware" {
        w167 = "2"
        w196 = "0"
        w195 = u16 7001 items=["Read temperature (F)"=4001, "Read setpoint (F)"=8029, "Write setpoint (F)"=7001, "Read autotune status"=8027, "Write start autotune"=8026]
        # "TODO:\nEdit the cDAQ start VI\nto accommodate\nadditional relay modules,\nthe digital output module, etc."
        # "TODO:\nUse the \"reactor enabled\"\nbooleans to enable or\ndisable these temperature\nchannel initializations"
        # "TODO:\nUse the \"reactor enabled\"\nbooleans to enable or\ndisable these valve\ninitializations"
        # "Initialize the Watlow and write low setpoints"
        # "Initialize the Sensors"
        # "Initialize the Pumps and Valves"
        # "Home the Liquid Handler"
        n100 = local read "Gilson COM"() -> (w279:refnum<visa-resource-name>)
        n101 = local read "Gilson LH ID"() -> (w278:i32)
        n102 = call "Gilson Home Device.vi"("error in"=errorcluster {"status"=FALSE, "code"=0, "source"=""} ("error constant"), "ID (30 for GX-241)"=w278, "VISA resource name"=w279) -> ("error out"=w303:errorcluster)  [unwired: 6 in, 2 out]
        n103 = local read "Reactor Valve 2 COM"() -> (w257:refnum<visa-resource-name>)
        n104 = local read "Reactor Valve 3 COM"() -> (w255:refnum<visa-resource-name>)
        n105 = local read "Reactor Valve 4 COM"() -> (w253:refnum<visa-resource-name>)
        n106 = local read "Reactor Valve 5 COM"() -> (w251:refnum<visa-resource-name>)
        n107 = local read "Reactor Valve 6 COM"() -> (w249:refnum<visa-resource-name>)
        n108 = local read "Reactor Valve 7 COM"() -> (w247:refnum<visa-resource-name>)
        n109 = local read "Reactor Valve 8 COM"() -> (w245:refnum<visa-resource-name>)
        n110 = local read "Reactor Valve 9 COM"() -> (w243:refnum<visa-resource-name>)
        n111 = local read "Reactor Valve 10 COM"() -> (w241:refnum<visa-resource-name>)
        n112 = local read "Injection Valve COM"() -> (w275:refnum<visa-resource-name>)
        n113 = call <vilib>:"Simple Error Handler.vi"("error in (no error)"=w303) -> ("error out"=w150:errorcluster)  [unwired: 4 in, 4 out]
        n114 = case shown="True" FALSE {
          tunnel: [w304 w306] -> w182
          tunnel: w150 -> [w304 w305]
          frame False {
            # "COMMENTING OUT REACTOR VALVE 1"
          }
          frame True {
            n115 = local read "Reactor Valve 1 COM"() -> (w310:refnum<visa-resource-name>)
            n116 = call "VALCO_OPEN.vi"("Error In (No Error)"=w305, "COM Port"=w310) -> ("Error Out"=w311:errorcluster, "COM Port (Out)"=w309:refnum<visa-resource-name>)  [unwired: 8 in]
            n117 = local read "Reactor Valve 1 ID"() -> (w307:i32)
            n118 = local read "Reactor Valve 1 Position - System"() -> (w308:string)
            n119 = call "VALCO_SET_POS_232.vi"("Error In"=w311, "New Position (as string)"=w308, "Valve ID"=w307, "COM Port In"=w309) -> ("Error Out"=w306:errorcluster)  [unwired: 5 in, 2 out]
          }
        }
        n120 = local read "Carrier Valve COM"() -> (w142:refnum<visa-resource-name>)
        n121 = local read "Injection Valve Position - LH Needle"() -> (w272:string)
        n122 = local read "Reactor Selector Valve\n - Upstream - COM"() -> (w287:refnum<visa-resource-name>)
        n123 = local read "Reactor Selector Valve Downstream COM"() -> (w169:refnum<visa-resource-name>)
        n124 = local read "LH Valve COM"() -> (w302:refnum<visa-resource-name>)
        n125 = local read "LH Valve Position - Needle"() -> (w290:string)
        n126 = local read "Analytical Valve COM"() -> (w271:refnum<visa-resource-name>)
        n127 = call "VALCO_OPEN.vi"("Error In (No Error)"=w150, "COM Port"=w257) -> ("Error Out"=w266:errorcluster, "COM Port (Out)"=w256:refnum<visa-resource-name>)  [unwired: 8 in]
        n128 = call "VALCO_OPEN.vi"("Error In (No Error)"=w150, "COM Port"=w255) -> ("Error Out"=w265:errorcluster, "COM Port (Out)"=w254:refnum<visa-resource-name>)  [unwired: 8 in]
        n129 = call "VALCO_OPEN.vi"("Error In (No Error)"=w150, "COM Port"=w253) -> ("Error Out"=w264:errorcluster, "COM Port (Out)"=w252:refnum<visa-resource-name>)  [unwired: 8 in]
        n130 = call "VALCO_OPEN.vi"("Error In (No Error)"=w150, "COM Port"=w251) -> ("Error Out"=w263:errorcluster, "COM Port (Out)"=w250:refnum<visa-resource-name>)  [unwired: 8 in]
        n131 = call "VALCO_OPEN.vi"("Error In (No Error)"=w150, "COM Port"=w249) -> ("Error Out"=w262:errorcluster, "COM Port (Out)"=w248:refnum<visa-resource-name>)  [unwired: 8 in]
        n132 = call "VALCO_OPEN.vi"("Error In (No Error)"=w150, "COM Port"=w247) -> ("Error Out"=w261:errorcluster, "COM Port (Out)"=w246:refnum<visa-resource-name>)  [unwired: 8 in]
        n133 = call "VALCO_OPEN.vi"("Error In (No Error)"=w150, "COM Port"=w245) -> ("Error Out"=w260:errorcluster, "COM Port (Out)"=w244:refnum<visa-resource-name>)  [unwired: 8 in]
        n134 = call "VALCO_OPEN.vi"("Error In (No Error)"=w150, "COM Port"=w243) -> ("Error Out"=w259:errorcluster, "COM Port (Out)"=w242:refnum<visa-resource-name>)  [unwired: 8 in]
        n135 = call "VALCO_OPEN.vi"("Error In (No Error)"=w150, "COM Port"=w241) -> ("Error Out"=w258:errorcluster, "COM Port (Out)"=w240:refnum<visa-resource-name>)  [unwired: 8 in]
        n136 = local read "Injection Valve ID"() -> (w273:i32)
        n137 = local read "LH Valve ID"() -> (w289:i32)
        n138 = local read "Reactor Valve 10 Position - System"() -> (w230:string)
        n139 = call "START_CDAQ_NIMAX_NSE_Parallel.vi"("error in (no error)"=errorcluster {"status"=FALSE, "code"=0, "source"=""} ("error constant")) -> ("analog input (NI 9205) task out"=w149:refnum<k21>, "analog input (NI 9205) error out"=w138:errorcluster, "relay output (NI 9482) task out"=w148:refnum<k21>, "relay output (NI 9482) error out"=w136:errorcluster)  [unwired: 21 in, 2 out]
        n140 = call "VALCO_OPEN.vi"("Error In (No Error)"=w150, "COM Port"=w275) -> ("Error Out"=w276:errorcluster, "COM Port (Out)"=w274:refnum<visa-resource-name>)  [unwired: 8 in]
        n141 = local read "Analytical Valve Position - System"() -> (w268:string)
        n142 = local read "Reactor Valve 2 Position - System"() -> (w238:string)
        n143 = local read "Reactor Valve 3 Position - System"() -> (w237:string)
        n144 = local read "Reactor Valve 4 Position - System"() -> (w236:string)
        n145 = local read "Reactor Valve 5 Position - System"() -> (w235:string)
        n146 = local read "Reactor Valve 6 Position - System"() -> (w234:string)
        n147 = local read "Reactor Valve 7 Position - System"() -> (w233:string)
        n148 = local read "Reactor Valve 8 Position - System"() -> (w232:string)
        n149 = local read "Reactor Valve 9 Position - System"() -> (w231:string)
        n150 = local read "Carrier Valve Position - System"() -> (w143:string)
        n151 = call "VALCO_OPEN.vi"("Error In (No Error)"=w150, "COM Port"=w142) -> ("Error Out"=w140:errorcluster, "COM Port (Out)"=w141:refnum<visa-resource-name>)  [unwired: 8 in]
        n152 = call "VALCO_OPEN.vi"("Error In (No Error)"=w150, "COM Port"=w271) -> ("Error Out"=w267:errorcluster, "COM Port (Out)"=w270:refnum<visa-resource-name>)  [unwired: 8 in]
        n153 = Unbundle By Name(w136) -> ("status"=→"Relay output DAQ error":bool)
        n154 = call "VALCO_OPEN.vi"("Error In (No Error)"=w150, "COM Port"=w302) -> ("Error Out"=w291:errorcluster, "COM Port (Out)"=w292:refnum<visa-resource-name>)  [unwired: 8 in]
        n155 = call "VALCO_OPEN.vi"("Error In (No Error)"=w150, "COM Port"=w169) -> ("Error Out"=w168:errorcluster, "COM Port (Out)"=w170:refnum<visa-resource-name>)  [unwired: 8 in]
        n156 = call "VALCO_OPEN.vi"("Error In (No Error)"=w150, "COM Port"=w287) -> ("Error Out"=w288:errorcluster, "COM Port (Out)"=w286:refnum<visa-resource-name>)  [unwired: 8 in]
        n157 = call "VALCO_SET_POS_232.vi"("Error In"=w276, "New Position (as string)"=w272, "Valve ID"=w273, "COM Port In"=w274) -> ()  [unwired: 5 in, 3 out]
        n158 = local read "Carrier Valve ID"() -> (w144:i32)
        n159 = local write "Analog Input (NI 9205) task out"(w149) -> ()
        n160 = local write "Analog Input DAQ Error"(w138) -> ()
        n161 = local write "Relay Output (NI 9482) task out"(w148) -> ()
        n162 = local write "Relay Output DAQ Error"(w136) -> ()
        n163 = local read "Watlow COM"() -> (w217:refnum<visa-resource-name>)
        n164 = local read "Vent Valve COM"() -> (w156:refnum<visa-resource-name>)
        n165 = local read "Analytical Valve ID"() -> (w269:i32)
        n166 = call "VALCO_SET_POS_232.vi"("Error In"=w267, "New Position (as string)"=w268, "Valve ID"=w269, "COM Port In"=w270) -> ("Error Out"=w166:errorcluster)  [unwired: 5 in, 2 out]
        n167 = call "VALCO_SET_POS_232.vi"("Error In"=w291, "New Position (as string)"=w290, "Valve ID"=w289, "COM Port In"=w292) -> ("Error Out"=w165:errorcluster)  [unwired: 5 in, 2 out]
        n168 = call "VALCO_SET_POS_232.vi"("Error In"=w140, "New Position (as string)"=w143, "Valve ID"=w144, "COM Port In"=w141) -> ("Error Out"=w139:errorcluster)  [unwired: 5 in, 2 out]
        n169 = call "VALCO_SET_POS_232.vi"("Error In"=w266, "New Position (as string)"=w238, "Valve ID"=0, "COM Port In"=w256) -> ("Error Out"=w181:errorcluster)  [unwired: 5 in, 2 out]
        n170 = call "VALCO_SET_POS_232.vi"("Error In"=w265, "New Position (as string)"=w237, "Valve ID"=0, "COM Port In"=w254) -> ("Error Out"=w180:errorcluster)  [unwired: 5 in, 2 out]
        n171 = call "VALCO_SET_POS_232.vi"("Error In"=w264, "New Position (as string)"=w236, "Valve ID"=0, "COM Port In"=w252) -> ("Error Out"=w179:errorcluster)  [unwired: 5 in, 2 out]
        n172 = call "VALCO_SET_POS_232.vi"("Error In"=w263, "New Position (as string)"=w235, "Valve ID"=0, "COM Port In"=w250) -> ("Error Out"=w178:errorcluster)  [unwired: 5 in, 2 out]
        n173 = call "VALCO_SET_POS_232.vi"("Error In"=w262, "New Position (as string)"=w234, "Valve ID"=0, "COM Port In"=w248) -> ("Error Out"=w177:errorcluster)  [unwired: 5 in, 2 out]
        n174 = call "VALCO_SET_POS_232.vi"("Error In"=w261, "New Position (as string)"=w233, "Valve ID"=0, "COM Port In"=w246) -> ("Error Out"=w176:errorcluster)  [unwired: 5 in, 2 out]
        n175 = call "VALCO_SET_POS_232.vi"("Error In"=w260, "New Position (as string)"=w232, "Valve ID"=0, "COM Port In"=w244) -> ("Error Out"=w175:errorcluster)  [unwired: 5 in, 2 out]
        n176 = call "VALCO_SET_POS_232.vi"("Error In"=w259, "New Position (as string)"=w231, "Valve ID"=0, "COM Port In"=w242) -> ("Error Out"=w174:errorcluster)  [unwired: 5 in, 2 out]
        n177 = call "VALCO_SET_POS_232.vi"("Error In"=w258, "New Position (as string)"=w230, "Valve ID"=0, "COM Port In"=w240) -> ("Error Out"=w173:errorcluster)  [unwired: 5 in, 2 out]
        n178 = call "Initialize.vi"("Comms Port"=w217, "Error In"=errorcluster {"status"=FALSE, "code"=0, "source"=""} ("error constant")) -> ("UUT Port 2"=w194:refnum<visa-resource-name>, "Error Out"=w193:errorcluster)  [unwired: 15 in, 1 out]
        n179 = local read "Vent Valve Position - System"() -> (w154:string)
        n180 = call "VALCO_SET_POS_232.vi"("Error In"=w168, "New Position (as string)"=w167, "Valve ID"=0, "COM Port In"=w170) -> ("Error Out"=w163:errorcluster)  [unwired: 5 in, 2 out]
        n181 = local read "Watlow Zone - Reactor 2"() -> (w214:dbl)
        n182 = local read "Watlow Instance - Reactor 2"() -> (w213:dbl)
        n183 = local read "Watlow Zone - Reactor 3"() -> (w212:dbl)
        n184 = local read "Watlow Instance - Reactor 3"() -> (w211:dbl)
        n185 = local read "Watlow Zone - Reactor 4"() -> (w210:dbl)
        n186 = local read "Watlow Instance - Reactor 4"() -> (w209:dbl)
        n187 = local read "Watlow Zone - Reactor 5"() -> (w208:dbl)
        n188 = local read "Watlow Instance - Reactor 5"() -> (w207:dbl)
        n189 = local read "Watlow Zone - Reactor 6"() -> (w206:dbl)
        n190 = local read "Watlow Instance - Reactor 6"() -> (w205:dbl)
        n191 = local read "Watlow Zone - Reactor 7"() -> (w204:dbl)
        n192 = local read "Watlow Instance - Reactor 7"() -> (w203:dbl)
        n193 = local read "Watlow Zone - Reactor 8"() -> (w202:dbl)
        n194 = local read "Watlow Instance - Reactor 8"() -> (w201:dbl)
        n195 = local read "Watlow Zone - Reactor 9"() -> (w199:dbl)
        n196 = local read "Watlow Instance - Reactor 9"() -> (w200:dbl)
        n197 = local read "Watlow Zone - Reactor 10"() -> (w198:dbl)
        n198 = local read "Watlow Instance - Reactor 10"() -> (w197:dbl)
        n199 = call "VALCO_SET_POS_232.vi"("Error In"=w288, "New Position (as string)"=w167, "Valve ID"=0, "COM Port In"=w286) -> ("Error Out"=w164:errorcluster)  [unwired: 5 in, 2 out]
        n200 = call "VALCO_OPEN.vi"("Error In (No Error)"=w150, "COM Port"=w156) -> ("Error Out"=w158:errorcluster, "COM Port (Out)"=w157:refnum<visa-resource-name>)  [unwired: 8 in]
        n201 = local read "Vent Valve ID"() -> (w155:i32)
        n202 = local read "Watlow Instance - Reactor 1"() -> (w215:dbl)
        n203 = local read "Watlow Zone - Reactor 1"() -> (w216:dbl)
        n204 = Unbundle By Name(w138) -> ("status"=w137:bool)
        n205 = call "VALCO_SET_POS_232.vi"("Error In"=w158, "New Position (as string)"=w154, "Valve ID"=w155, "COM Port In"=w157) -> ("Error Out"=w153:errorcluster)  [unwired: 5 in, 2 out]
        n206 = local read "Rinse Syringe Infuse Rate [uL/min]"() -> (w280:dbl)
        n207 = Merge Errors(w153, w166, w165, w139, w164, w163) -> (w151:errorcluster)
        n208 = local read "Carrier Syringe Infuse\nRate (Rinse) (uL/min)"() -> (w294:dbl)
        n209 = Merge Errors(w182, w181, w180, w179, w178, w177, w176, w175, w174, w173) -> (w172:errorcluster)
        n210 = local read "LH Withdraw\nFlow Rate (uL/min)"() -> (w293:dbl)
        n211 = local read "Carrier Pump COM"() -> (w300:refnum<visa-resource-name>)
        n212 = local write "Analog input DAQ error"(w137) -> ()
        n213 = local read "LH Pump COM"() -> (w301:refnum<visa-resource-name>)
        n214 = local read "Rinse Pump COM"() -> (w284:refnum<visa-resource-name>)
        n215 = call "Write.vi"("PC Comms Port"=w194, "Zone"=w216, "Parameter"=w195, "Instance"=w215, "Write Value"=w196, "Error In"=w193) -> ("Error Out"=w192:errorcluster)  [unwired: 13 in]
        n216 = call "Write.vi"("PC Comms Port"=w194, "Zone"=w214, "Parameter"=w195, "Instance"=w213, "Write Value"=w196, "Error In"=w193) -> ("Error Out"=w191:errorcluster)  [unwired: 13 in]
        n217 = call "Write.vi"("PC Comms Port"=w194, "Zone"=w212, "Parameter"=w195, "Instance"=w211, "Write Value"=w196, "Error In"=w193) -> ("Error Out"=w190:errorcluster)  [unwired: 13 in]
        n218 = call "Write.vi"("PC Comms Port"=w194, "Zone"=w210, "Parameter"=w195, "Instance"=w209, "Write Value"=w196, "Error In"=w193) -> ("Error Out"=w189:errorcluster)  [unwired: 13 in]
        n219 = call "Write.vi"("PC Comms Port"=w194, "Zone"=w208, "Parameter"=w195, "Instance"=w207, "Write Value"=w196, "Error In"=w193) -> ("Error Out"=w188:errorcluster)  [unwired: 13 in]
        n220 = call "Write.vi"("PC Comms Port"=w194, "Zone"=w206, "Parameter"=w195, "Instance"=w205, "Write Value"=w196, "Error In"=w193) -> ("Error Out"=w187:errorcluster)  [unwired: 13 in]
        n221 = call "Write.vi"("PC Comms Port"=w194, "Zone"=w204, "Parameter"=w195, "Instance"=w203, "Write Value"=w196, "Error In"=w193) -> ("Error Out"=w186:errorcluster)  [unwired: 13 in]
        n222 = call "Write.vi"("PC Comms Port"=w194, "Zone"=w202, "Parameter"=w195, "Instance"=w201, "Write Value"=w196, "Error In"=w193) -> ("Error Out"=w185:errorcluster)  [unwired: 13 in]
        n223 = call "Write.vi"("PC Comms Port"=w194, "Zone"=w199, "Parameter"=w195, "Instance"=w200, "Write Value"=w196, "Error In"=w193) -> ("Error Out"=w184:errorcluster)  [unwired: 13 in]
        n224 = call "Write.vi"("PC Comms Port"=w194, "Zone"=w198, "Parameter"=w195, "Instance"=w197, "Write Value"=w196, "Error In"=w193) -> ("Error Out"=w183:errorcluster)  [unwired: 13 in]
        n225 = case shown="False" FALSE {
          tunnel: [w312 w314] -> w160
          tunnel: w150 -> [w312 w313]
          frame False {
            # "commenting out the online pump"
          }
          frame True {
            n226 = local read "Online Pump COM"() -> (w320:refnum<visa-resource-name>)
            n227 = call "Initialize.vi"("error in (no error)"=w313, "VISA resource name"=w320) -> ("error out"=w315:errorcluster, "VISA resource name out"=w319:refnum<visa-resource-name>)  [unwired: 8 in]
            n228 = local read "Online Syringe Infuse Rate [uL/min]"() -> (w316:dbl)
            n229 = local read "Online Pump ID"() -> (w318:i32)
            n230 = local read "Online Syringe Diameter (mm)"() -> (w317:dbl)
            n231 = call "HARVARD_INITIALIZE_PUMP.vi"("VISA resource name"=w319, "Pump address (0)"=w318, "Syringe Diameter (9.525 mm)"=w317, "Infuse Flow Rate (80)"=w316, "error in (no error)"=w315) -> ("error out"=w314:errorcluster)  [unwired: 21 in, 1 out]
          }
        }
        n232 = call "Initialize.vi"("error in (no error)"=w150, "VISA resource name"=w300) -> ("error out"=w128:errorcluster, "VISA resource name out"=w298:refnum<visa-resource-name>)  [unwired: 8 in]
        n233 = local read "Carrier Pump ID"() -> (w296:i32)
        n234 = call "Initialize.vi"("error in (no error)"=w150, "VISA resource name"=w301) -> ("error out"=w130:errorcluster, "VISA resource name out"=w299:refnum<visa-resource-name>)  [unwired: 8 in]
        n235 = call "Time Delay78"("error in (no error)"=w128, "Delay Time (s)"=0.5) -> ("error out"=w127:errorcluster)  [unwired: 9 in]
        n236 = call "Time Delay77"("error in (no error)"=w130, "Delay Time (s)"=0.5) -> ("error out"=w129:errorcluster)  [unwired: 9 in]
        n237 = call "Initialize.vi"("error in (no error)"=w150, "VISA resource name"=w284) -> ("error out"=w132:errorcluster, "VISA resource name out"=w283:refnum<visa-resource-name>)  [unwired: 8 in]
        n238 = call "Time Delay76"() -> ()  [unwired: 11 in, 1 out]
        n239 = local write "Temperature Control Error - Reactor 10"(w183) -> ()
        n240 = local write "Temperature Control Error - Reactor 2"(w191) -> ()
        n241 = local write "Temperature Control Error - Reactor 3"(w190) -> ()
        n242 = local write "Temperature Control Error - Reactor 4"(w189) -> ()
        n243 = local write "Temperature Control Error - Reactor 5"(w188) -> ()
        n244 = local write "Temperature Control Error - Reactor 6"(w187) -> ()
        n245 = local write "Temperature Control Error - Reactor 7"(w186) -> ()
        n246 = local write "Temperature Control Error - Reactor 8"(w185) -> ()
        n247 = local write "Temperature Control Error - Reactor 9"(w184) -> ()
        n248 = local read "Rinse Syringe Diameter [mm]"() -> (w282:dbl)
        n249 = call "Time Delay75"("error in (no error)"=w132, "Delay Time (s)"=0.5) -> ("error out"=w131:errorcluster)  [unwired: 9 in]
        n250 = local read "LH Pump ID"() -> (w297:i32)
        n251 = call "HARVARD_INITIALIZE_PUMP.vi"("VISA resource name"=w299, "Pump address (0)"=w297, "Syringe Diameter (9.525 mm)"=4.75, "Infuse Flow Rate (80)"=w293, "error in (no error)"=w129) -> ("error out"=w162:errorcluster)  [unwired: 21 in, 1 out]
        n252 = local read "Carrier Syringe Diameter (mm)"() -> (w295:dbl)
        n253 = call "HARVARD_INITIALIZE_PUMP.vi"("VISA resource name"=w298, "Pump address (0)"=w296, "Syringe Diameter (9.525 mm)"=w295, "Infuse Flow Rate (80)"=w294, "error in (no error)"=w127) -> ("error out"=w161:errorcluster)  [unwired: 21 in, 1 out]
        n254 = call "HARVARD_INITIALIZE_PUMP.vi"("VISA resource name"=w283, "Pump address (0)"=0, "Syringe Diameter (9.525 mm)"=w282, "Infuse Flow Rate (80)"=w280, "error in (no error)"=w131) -> ("error out"=w159:errorcluster)  [unwired: 21 in, 1 out]
        n255 = local write "Temperature Control Error - Reactor 1"(w192) -> ()
        n256 = Merge Errors(w162, w161, w160, w159) -> (w152:errorcluster)
        n257 = Merge Errors(w150, w151, w152, w172, w192, w191, w190, w189, w188, w187, w186, w185, w184, w183, w138, w136) -> (w220:errorcluster)
        n258 = Unbundle By Name(w220) -> ("status"=w219:bool)
        n259 = case shown="True" w219 {
          frame False {
            n260 = local write "Hardware communication established"(TRUE) -> ()
            n261 = property on="Pressurization confirmed" class="Bool (strict)"("DisabledEnum"=T8."Enabled") -> ()  [unwired: 2 in, 2 out]
          }
          frame True {
            n262 = call "Time Delay"("Delay Time (s)"=5.0) -> ("error out"=w324:errorcluster)  [unwired: 10 in]
            n263 = call "Display Message to User"("error in (no error)"=w324, "Message"="Not all hardware could be initialized; the VI will now quit. Please check all hardware connections. It may be necessary to cycle all power off and back on. Allow the control box up to 30 seconds to boot up after turning it on.") -> ("OK"=w325:bool)  [unwired: 8 in, 1 out]
            n264 = Stop(stop? (T)=w325) -> ()
          }
        }
      }
      frame "Wait for user to confirm pressurization" {
        n265 = local read "Pressurization confirmed"() -> (w328:bool)
        n266 = case shown="False" w328 {
          tunnel: [Hardware_Initiation_Enum."Wait for user to confirm pressurization" ("Enum") Hardware_Initiation_Enum."Pressurize everything" ("Enum")] -> w329
          frame False {
            n267 = Wait (ms)(milliseconds to wait=100) -> ()  [unwired: 1 out]
          }
          frame True {
            n268 = property on="Pressurization confirmed" class="Bool (strict)"("DisabledEnum"=T8."Disabled and Grayed Out") -> ()  [unwired: 2 in, 2 out]
          }
        }
      }
      frame "Pressurize everything" {
        w345 = "10"
        w362 = "9"
        w375 = "8"
        w392 = "7"
        w399 = "6"
        w416 = "5"
        w423 = "4"
        w440 = "3"
        w448 = "2"
        w460 = "2"
        w457 = errorcluster {"status"=FALSE, "code"=0, "source"=""} ("error constant")
        w473 = 5
        # "Pressurize the reactor loops"
        n269 = case shown="False" FALSE {
          tunnel: w457 -> [w492 w496]
          tunnel: [w492 w494] -> w444
          tunnel: [0 w493] -> w338
          frame False {
            # "JUST COMMENTING OUT REACTOR VALVE 1"
          }
          frame True {
            w505 = "1"
            w493 = 3
            n270 = local read "Reactor Valve 1 COM"() -> (w498:refnum<visa-resource-name>)
            n271 = local read "Reactor Valve 1 ID"() -> (w497:i32)
            n272 = local read "Reactor Selector Valve\n - Upstream - COM"() -> (w503:refnum<visa-resource-name>)
            n273 = local read "Reactor Selector Valve Downstream COM"() -> (w500:refnum<visa-resource-name>)
            n274 = call "VALCO_OPEN.vi"("Error In (No Error)"=w496, "COM Port"=w503) -> ("Error Out"=w504:errorcluster, "COM Port (Out)"=w502:refnum<visa-resource-name>)  [unwired: 8 in]
            n275 = call "VALCO_OPEN.vi"("Error In (No Error)"=w496, "COM Port"=w500) -> ("Error Out"=w499:errorcluster, "COM Port (Out)"=w501:refnum<visa-resource-name>)  [unwired: 8 in]
            n276 = call "VALCO_SET_POS_232.vi"("Error In"=w504, "New Position (as string)"=w505, "Valve ID"=0, "COM Port In"=w502) -> ("Error Out"=w495:errorcluster)  [unwired: 5 in, 2 out]
            n277 = call "VALCO_SET_POS_232.vi"("Error In"=w499, "New Position (as string)"=w505, "Valve ID"=0, "COM Port In"=w501) -> ()  [unwired: 5 in, 3 out]
            n278 = for {
              N: w493 -> [_]
              tunnel: w498 -> [w511]
              tunnel: w497 -> [w510]
              shift-right: [w509] -> w494
              shift-left: w495 -> [w508]
              n279 = local read "Reactor Valve 1 Position - Reaction"() -> (w517:string)
              n280 = call "Time Delay5"("error in (no error)"=w508, "Delay Time (s)"=1) -> ("error out"=w514:errorcluster)  [unwired: 9 in]
              n281 = call "VALCO_SET_POS_232.vi"("Error In"=w514, "New Position (as string)"=w517, "Valve ID"=w510, "COM Port In"=w511) -> ("Error Out"=w515:errorcluster, "Valve ID out"=w519:u8, "COM Port Out"=w520:refnum<visa-resource-name>)  [unwired: 5 in]
              n282 = local read "Reactor Valve 1 Position - System"() -> (w518:string)
              n283 = call "Time Delay6"("error in (no error)"=w515, "Delay Time (s)"=1) -> ("error out"=w516:errorcluster)  [unwired: 9 in]
              n284 = call "VALCO_SET_POS_232.vi"("Error In"=w516, "New Position (as string)"=w518, "Valve ID"=w519, "COM Port In"=w520) -> ("Error Out"=w509:errorcluster)  [unwired: 5 in, 2 out]
            }
          }
        }
        n285 = local read "Reactor Valve 6 COM"() -> (w406:refnum<visa-resource-name>)
        n286 = local read "Reactor Valve 6 ID"() -> (w407:dbl)
        n287 = local read "Reactor Selector Valve\n - Upstream - COM"() -> (w401:refnum<visa-resource-name>)
        n288 = local read "Reactor Selector Valve Downstream COM"() -> (w404:refnum<visa-resource-name>)
        n289 = local read "Reactor Valve 2 COM"() -> (w455:refnum<visa-resource-name>)
        n290 = local read "Reactor Valve 2 ID"() -> (w456:i32)
        n291 = local read "Reactor Selector Valve\n - Upstream - COM"() -> (w450:refnum<visa-resource-name>)
        n292 = local read "Reactor Selector Valve Downstream COM"() -> (w453:refnum<visa-resource-name>)
        n293 = local read "Reactor Valve 10 COM"() -> (w352:refnum<visa-resource-name>)
        n294 = local read "Reactor Valve 10 ID"() -> (w353:dbl)
        n295 = local read "Reactor Valve 5 COM"() -> (w409:refnum<visa-resource-name>)
        n296 = local read "Reactor Valve 5 ID"() -> (w408:dbl)
        n297 = local read "Reactor Selector Valve\n - Upstream - COM"() -> (w414:refnum<visa-resource-name>)
        n298 = local read "Reactor Selector Valve Downstream COM"() -> (w411:refnum<visa-resource-name>)
        n299 = local read "Reactor Valve 3 COM"() -> (w433:refnum<visa-resource-name>)
        n300 = local read "Reactor Valve 3 ID"() -> (w432:dbl)
        n301 = local read "Reactor Selector Valve\n - Upstream - COM"() -> (w438:refnum<visa-resource-name>)
        n302 = local read "Reactor Selector Valve Downstream COM"() -> (w435:refnum<visa-resource-name>)
        n303 = local read "Reactor Valve 4 COM"() -> (w430:refnum<visa-resource-name>)
        n304 = local read "Reactor Valve 4 ID"() -> (w431:dbl)
        n305 = local read "Reactor Selector Valve\n - Upstream - COM"() -> (w425:refnum<visa-resource-name>)
        n306 = local read "Reactor Selector Valve Downstream COM"() -> (w428:refnum<visa-resource-name>)
        n307 = local read "Reactor Valve 7 COM"() -> (w385:refnum<visa-resource-name>)
        n308 = local read "Reactor Valve 7 ID"() -> (w384:dbl)
        n309 = local read "Reactor Selector Valve\n - Upstream - COM"() -> (w390:refnum<visa-resource-name>)
        n310 = local read "Reactor Selector Valve Downstream COM"() -> (w387:refnum<visa-resource-name>)
        n311 = local read "Reactor Selector Valve\n - Upstream - COM"() -> (w347:refnum<visa-resource-name>)
        n312 = local read "Reactor Selector Valve Downstream COM"() -> (w350:refnum<visa-resource-name>)
        n313 = local read "Reactor Valve 8 COM"() -> (w382:refnum<visa-resource-name>)
        n314 = local read "Reactor Valve 8 ID"() -> (w383:dbl)
        n315 = local read "Reactor Selector Valve\n - Upstream - COM"() -> (w377:refnum<visa-resource-name>)
        n316 = local read "Reactor Selector Valve Downstream COM"() -> (w380:refnum<visa-resource-name>)
        n317 = local read "Reactor Valve 9 COM"() -> (w355:refnum<visa-resource-name>)
        n318 = local read "Reactor Valve 9 ID"() -> (w354:dbl)
        n319 = local read "Reactor Selector Valve\n - Upstream - COM"() -> (w360:refnum<visa-resource-name>)
        n320 = local read "Reactor Selector Valve Downstream COM"() -> (w357:refnum<visa-resource-name>)
        n321 = call "VALCO_OPEN.vi"("Error In (No Error)"=w444, "COM Port"=w450) -> ("Error Out"=w449:errorcluster, "COM Port (Out)"=w451:refnum<visa-resource-name>)  [unwired: 8 in]
        n322 = call "VALCO_OPEN.vi"("Error In (No Error)"=w444, "COM Port"=w453) -> ("Error Out"=w454:errorcluster, "COM Port (Out)"=w452:refnum<visa-resource-name>)  [unwired: 8 in]
        n323 = call "VALCO_SET_POS_232.vi"("Error In"=w449, "New Position (as string)"=w448, "Valve ID"=0, "COM Port In"=w451) -> ("Error Out"=w445:errorcluster)  [unwired: 5 in, 2 out]
        n324 = call "VALCO_SET_POS_232.vi"("Error In"=w454, "New Position (as string)"=w448, "Valve ID"=0, "COM Port In"=w452) -> ()  [unwired: 5 in, 3 out]
        n325 = for {
          N: w338 -> [_]
          tunnel: w455 -> [w627]
          tunnel: w456 -> [w626]
          shift-right: [w625] -> w371
          shift-left: w445 -> [w637]
          n326 = local read "Reactor Valve 2 Position - Reaction"() -> (w633:string)
          n327 = call "Time Delay47"("error in (no error)"=w637, "Delay Time (s)"=1) -> ("error out"=w630:errorcluster)  [unwired: 9 in]
          n328 = call "VALCO_SET_POS_232.vi"("Error In"=w630, "New Position (as string)"=w633, "Valve ID"=w626, "COM Port In"=w627) -> ("Error Out"=w631:errorcluster, "Valve ID out"=w635:u8, "COM Port Out"=w636:refnum<visa-resource-name>)  [unwired: 5 in]
          n329 = local read "Reactor Valve 2 Position - System"() -> (w634:string)
          n330 = call "Time Delay48"("error in (no error)"=w631, "Delay Time (s)"=1) -> ("error out"=w632:errorcluster)  [unwired: 9 in]
          n331 = call "VALCO_SET_POS_232.vi"("Error In"=w632, "New Position (as string)"=w634, "Valve ID"=w635, "COM Port In"=w636) -> ("Error Out"=w625:errorcluster)  [unwired: 5 in, 2 out]
        }
        n332 = call "VALCO_OPEN.vi"("Error In (No Error)"=w371, "COM Port"=w438) -> ("Error Out"=w439:errorcluster, "COM Port (Out)"=w437:refnum<visa-resource-name>)  [unwired: 8 in]
        n333 = call "VALCO_OPEN.vi"("Error In (No Error)"=w371, "COM Port"=w435) -> ("Error Out"=w434:errorcluster, "COM Port (Out)"=w436:refnum<visa-resource-name>)  [unwired: 8 in]
        n334 = call "VALCO_SET_POS_232.vi"("Error In"=w439, "New Position (as string)"=w440, "Valve ID"=0, "COM Port In"=w437) -> ("Error Out"=w443:errorcluster)  [unwired: 5 in, 2 out]
        n335 = call "VALCO_SET_POS_232.vi"("Error In"=w434, "New Position (as string)"=w440, "Valve ID"=0, "COM Port In"=w436) -> ()  [unwired: 5 in, 3 out]
        n336 = for {
          N: w338 -> [_]
          tunnel: w433 -> [w614]
          tunnel: w432 -> [w613]
          shift-right: [w612] -> w370
          shift-left: w443 -> [w624]
          n337 = local read "Reactor Valve 3 Position - Reaction"() -> (w620:string)
          n338 = call "Time Delay49"("error in (no error)"=w624, "Delay Time (s)"=1) -> ("error out"=w617:errorcluster)  [unwired: 9 in]
          n339 = call "VALCO_SET_POS_232.vi"("Error In"=w617, "New Position (as string)"=w620, "Valve ID"=w613, "COM Port In"=w614) -> ("Error Out"=w618:errorcluster, "Valve ID out"=w622:u8, "COM Port Out"=w623:refnum<visa-resource-name>)  [unwired: 5 in]
          n340 = local read "Reactor Valve 3 Position - System"() -> (w621:string)
          n341 = call "Time Delay50"("error in (no error)"=w618, "Delay Time (s)"=1) -> ("error out"=w619:errorcluster)  [unwired: 9 in]
          n342 = call "VALCO_SET_POS_232.vi"("Error In"=w619, "New Position (as string)"=w621, "Valve ID"=w622, "COM Port In"=w623) -> ("Error Out"=w612:errorcluster)  [unwired: 5 in, 2 out]
        }
        n343 = call "VALCO_OPEN.vi"("Error In (No Error)"=w370, "COM Port"=w425) -> ("Error Out"=w424:errorcluster, "COM Port (Out)"=w426:refnum<visa-resource-name>)  [unwired: 8 in]
        n344 = call "VALCO_OPEN.vi"("Error In (No Error)"=w370, "COM Port"=w428) -> ("Error Out"=w429:errorcluster, "COM Port (Out)"=w427:refnum<visa-resource-name>)  [unwired: 8 in]
        n345 = call "VALCO_SET_POS_232.vi"("Error In"=w424, "New Position (as string)"=w423, "Valve ID"=0, "COM Port In"=w426) -> ("Error Out"=w420:errorcluster)  [unwired: 5 in, 2 out]
        n346 = call "VALCO_SET_POS_232.vi"("Error In"=w429, "New Position (as string)"=w423, "Valve ID"=0, "COM Port In"=w427) -> ()  [unwired: 5 in, 3 out]
        n347 = for {
          N: w338 -> [_]
          tunnel: w430 -> [w601]
          tunnel: w431 -> [w600]
          shift-right: [w599] -> w369
          shift-left: w420 -> [w611]
          n348 = local read "Reactor Valve 4 Position - Reaction"() -> (w607:string)
          n349 = call "Time Delay51"("error in (no error)"=w611, "Delay Time (s)"=1) -> ("error out"=w604:errorcluster)  [unwired: 9 in]
          n350 = call "VALCO_SET_POS_232.vi"("Error In"=w604, "New Position (as string)"=w607, "Valve ID"=w600, "COM Port In"=w601) -> ("Error Out"=w605:errorcluster, "Valve ID out"=w609:u8, "COM Port Out"=w610:refnum<visa-resource-name>)  [unwired: 5 in]
          n351 = local read "Reactor Valve 4 Position - System"() -> (w608:string)
          n352 = call "Time Delay52"("error in (no error)"=w605, "Delay Time (s)"=1) -> ("error out"=w606:errorcluster)  [unwired: 9 in]
          n353 = call "VALCO_SET_POS_232.vi"("Error In"=w606, "New Position (as string)"=w608, "Valve ID"=w609, "COM Port In"=w610) -> ("Error Out"=w599:errorcluster)  [unwired: 5 in, 2 out]
        }
        n354 = call "VALCO_OPEN.vi"("Error In (No Error)"=w369, "COM Port"=w414) -> ("Error Out"=w415:errorcluster, "COM Port (Out)"=w413:refnum<visa-resource-name>)  [unwired: 8 in]
        n355 = call "VALCO_OPEN.vi"("Error In (No Error)"=w369, "COM Port"=w411) -> ("Error Out"=w410:errorcluster, "COM Port (Out)"=w412:refnum<visa-resource-name>)  [unwired: 8 in]
        n356 = call "VALCO_SET_POS_232.vi"("Error In"=w415, "New Position (as string)"=w416, "Valve ID"=0, "COM Port In"=w413) -> ("Error Out"=w419:errorcluster)  [unwired: 5 in, 2 out]
        n357 = call "VALCO_SET_POS_232.vi"("Error In"=w410, "New Position (as string)"=w416, "Valve ID"=0, "COM Port In"=w412) -> ()  [unwired: 5 in, 3 out]
        n358 = for {
          N: w338 -> [_]
          tunnel: w409 -> [w588]
          tunnel: w408 -> [w587]
          shift-right: [w586] -> w368
          shift-left: w419 -> [w598]
          n359 = local read "Reactor Valve 5 Position - Reaction"() -> (w594:string)
          n360 = call "Time Delay53"("error in (no error)"=w598, "Delay Time (s)"=1) -> ("error out"=w591:errorcluster)  [unwired: 9 in]
          n361 = call "VALCO_SET_POS_232.vi"("Error In"=w591, "New Position (as string)"=w594, "Valve ID"=w587, "COM Port In"=w588) -> ("Error Out"=w592:errorcluster, "Valve ID out"=w596:u8, "COM Port Out"=w597:refnum<visa-resource-name>)  [unwired: 5 in]
          n362 = local read "Reactor Valve 5 Position - System"() -> (w595:string)
          n363 = call "Time Delay54"("error in (no error)"=w592, "Delay Time (s)"=1) -> ("error out"=w593:errorcluster)  [unwired: 9 in]
          n364 = call "VALCO_SET_POS_232.vi"("Error In"=w593, "New Position (as string)"=w595, "Valve ID"=w596, "COM Port In"=w597) -> ("Error Out"=w586:errorcluster)  [unwired: 5 in, 2 out]
        }
        n365 = call "VALCO_OPEN.vi"("Error In (No Error)"=w368, "COM Port"=w401) -> ("Error Out"=w400:errorcluster, "COM Port (Out)"=w402:refnum<visa-resource-name>)  [unwired: 8 in]
        n366 = call "VALCO_OPEN.vi"("Error In (No Error)"=w368, "COM Port"=w404) -> ("Error Out"=w405:errorcluster, "COM Port (Out)"=w403:refnum<visa-resource-name>)  [unwired: 8 in]
        n367 = call "VALCO_SET_POS_232.vi"("Error In"=w400, "New Position (as string)"=w399, "Valve ID"=0, "COM Port In"=w402) -> ("Error Out"=w396:errorcluster)  [unwired: 5 in, 2 out]
        n368 = call "VALCO_SET_POS_232.vi"("Error In"=w405, "New Position (as string)"=w399, "Valve ID"=0, "COM Port In"=w403) -> ()  [unwired: 5 in, 3 out]
        n369 = for {
          N: w338 -> [_]
          tunnel: w406 -> [w575]
          tunnel: w407 -> [w574]
          shift-right: [w573] -> w367
          shift-left: w396 -> [w585]
          n370 = local read "Reactor Valve 6 Position - Reaction"() -> (w581:string)
          n371 = call "Time Delay55"("error in (no error)"=w585, "Delay Time (s)"=1) -> ("error out"=w578:errorcluster)  [unwired: 9 in]
          n372 = call "VALCO_SET_POS_232.vi"("Error In"=w578, "New Position (as string)"=w581, "Valve ID"=w574, "COM Port In"=w575) -> ("Error Out"=w579:errorcluster, "Valve ID out"=w583:u8, "COM Port Out"=w584:refnum<visa-resource-name>)  [unwired: 5 in]
          n373 = local read "Reactor Valve 6 Position - System"() -> (w582:string)
          n374 = call "Time Delay56"("error in (no error)"=w579, "Delay Time (s)"=1) -> ("error out"=w580:errorcluster)  [unwired: 9 in]
          n375 = call "VALCO_SET_POS_232.vi"("Error In"=w580, "New Position (as string)"=w582, "Valve ID"=w583, "COM Port In"=w584) -> ("Error Out"=w573:errorcluster)  [unwired: 5 in, 2 out]
        }
        n376 = call "VALCO_OPEN.vi"("Error In (No Error)"=w367, "COM Port"=w390) -> ("Error Out"=w391:errorcluster, "COM Port (Out)"=w389:refnum<visa-resource-name>)  [unwired: 8 in]
        n377 = call "VALCO_OPEN.vi"("Error In (No Error)"=w367, "COM Port"=w387) -> ("Error Out"=w386:errorcluster, "COM Port (Out)"=w388:refnum<visa-resource-name>)  [unwired: 8 in]
        n378 = call "VALCO_SET_POS_232.vi"("Error In"=w391, "New Position (as string)"=w392, "Valve ID"=0, "COM Port In"=w389) -> ("Error Out"=w395:errorcluster)  [unwired: 5 in, 2 out]
        n379 = call "VALCO_SET_POS_232.vi"("Error In"=w386, "New Position (as string)"=w392, "Valve ID"=0, "COM Port In"=w388) -> ()  [unwired: 5 in, 3 out]
        n380 = for {
          N: w338 -> [_]
          tunnel: w385 -> [w562]
          tunnel: w384 -> [w561]
          shift-right: [w560] -> w366
          shift-left: w395 -> [w572]
          n381 = local read "Reactor Valve 7 Position - Reaction"() -> (w568:string)
          n382 = call "Time Delay57"("error in (no error)"=w572, "Delay Time (s)"=1) -> ("error out"=w565:errorcluster)  [unwired: 9 in]
          n383 = call "VALCO_SET_POS_232.vi"("Error In"=w565, "New Position (as string)"=w568, "Valve ID"=w561, "COM Port In"=w562) -> ("Error Out"=w566:errorcluster, "Valve ID out"=w570:u8, "COM Port Out"=w571:refnum<visa-resource-name>)  [unwired: 5 in]
          n384 = local read "Reactor Valve 7 Position - System"() -> (w569:string)
          n385 = call "Time Delay58"("error in (no error)"=w566, "Delay Time (s)"=1) -> ("error out"=w567:errorcluster)  [unwired: 9 in]
          n386 = call "VALCO_SET_POS_232.vi"("Error In"=w567, "New Position (as string)"=w569, "Valve ID"=w570, "COM Port In"=w571) -> ("Error Out"=w560:errorcluster)  [unwired: 5 in, 2 out]
        }
        n387 = call "VALCO_OPEN.vi"("Error In (No Error)"=w366, "COM Port"=w377) -> ("Error Out"=w376:errorcluster, "COM Port (Out)"=w378:refnum<visa-resource-name>)  [unwired: 8 in]
        n388 = call "VALCO_OPEN.vi"("Error In (No Error)"=w366, "COM Port"=w380) -> ("Error Out"=w381:errorcluster, "COM Port (Out)"=w379:refnum<visa-resource-name>)  [unwired: 8 in]
        n389 = call "VALCO_SET_POS_232.vi"("Error In"=w376, "New Position (as string)"=w375, "Valve ID"=0, "COM Port In"=w378) -> ("Error Out"=w372:errorcluster)  [unwired: 5 in, 2 out]
        n390 = call "VALCO_SET_POS_232.vi"("Error In"=w381, "New Position (as string)"=w375, "Valve ID"=0, "COM Port In"=w379) -> ()  [unwired: 5 in, 3 out]
        n391 = for {
          N: w338 -> [_]
          tunnel: w382 -> [w549]
          tunnel: w383 -> [w548]
          shift-right: [w547] -> w341
          shift-left: w372 -> [w559]
          n392 = local read "Reactor Valve 8 Position - Reaction"() -> (w555:string)
          n393 = call "Time Delay59"("error in (no error)"=w559, "Delay Time (s)"=1) -> ("error out"=w552:errorcluster)  [unwired: 9 in]
          n394 = call "VALCO_SET_POS_232.vi"("Error In"=w552, "New Position (as string)"=w555, "Valve ID"=w548, "COM Port In"=w549) -> ("Error Out"=w553:errorcluster, "Valve ID out"=w557:u8, "COM Port Out"=w558:refnum<visa-resource-name>)  [unwired: 5 in]
          n395 = local read "Reactor Valve 8 Position - System"() -> (w556:string)
          n396 = call "Time Delay60"("error in (no error)"=w553, "Delay Time (s)"=1) -> ("error out"=w554:errorcluster)  [unwired: 9 in]
          n397 = call "VALCO_SET_POS_232.vi"("Error In"=w554, "New Position (as string)"=w556, "Valve ID"=w557, "COM Port In"=w558) -> ("Error Out"=w547:errorcluster)  [unwired: 5 in, 2 out]
        }
        n398 = call "VALCO_OPEN.vi"("Error In (No Error)"=w341, "COM Port"=w360) -> ("Error Out"=w361:errorcluster, "COM Port (Out)"=w359:refnum<visa-resource-name>)  [unwired: 8 in]
        n399 = call "VALCO_OPEN.vi"("Error In (No Error)"=w341, "COM Port"=w357) -> ("Error Out"=w356:errorcluster, "COM Port (Out)"=w358:refnum<visa-resource-name>)  [unwired: 8 in]
        n400 = call "VALCO_SET_POS_232.vi"("Error In"=w361, "New Position (as string)"=w362, "Valve ID"=0, "COM Port In"=w359) -> ("Error Out"=w365:errorcluster)  [unwired: 5 in, 2 out]
        n401 = call "VALCO_SET_POS_232.vi"("Error In"=w356, "New Position (as string)"=w362, "Valve ID"=0, "COM Port In"=w358) -> ()  [unwired: 5 in, 3 out]
        n402 = for {
          N: w338 -> [_]
          tunnel: w355 -> [w536]
          tunnel: w354 -> [w535]
          shift-right: [w534] -> w340
          shift-left: w365 -> [w546]
          n403 = local read "Reactor Valve 9 Position - Reaction"() -> (w542:string)
          n404 = call "Time Delay61"("error in (no error)"=w546, "Delay Time (s)"=1) -> ("error out"=w539:errorcluster)  [unwired: 9 in]
          n405 = call "VALCO_SET_POS_232.vi"("Error In"=w539, "New Position (as string)"=w542, "Valve ID"=w535, "COM Port In"=w536) -> ("Error Out"=w540:errorcluster, "Valve ID out"=w544:u8, "COM Port Out"=w545:refnum<visa-resource-name>)  [unwired: 5 in]
          n406 = local read "Reactor Valve 9 Position - System"() -> (w543:string)
          n407 = call "Time Delay62"("error in (no error)"=w540, "Delay Time (s)"=1) -> ("error out"=w541:errorcluster)  [unwired: 9 in]
          n408 = call "VALCO_SET_POS_232.vi"("Error In"=w541, "New Position (as string)"=w543, "Valve ID"=w544, "COM Port In"=w545) -> ("Error Out"=w534:errorcluster)  [unwired: 5 in, 2 out]
        }
        n409 = call "VALCO_OPEN.vi"("Error In (No Error)"=w340, "COM Port"=w347) -> ("Error Out"=w346:errorcluster, "COM Port (Out)"=w348:refnum<visa-resource-name>)  [unwired: 8 in]
        n410 = call "VALCO_OPEN.vi"("Error In (No Error)"=w340, "COM Port"=w350) -> ("Error Out"=w351:errorcluster, "COM Port (Out)"=w349:refnum<visa-resource-name>)  [unwired: 8 in]
        n411 = call "VALCO_SET_POS_232.vi"("Error In"=w346, "New Position (as string)"=w345, "Valve ID"=0, "COM Port In"=w348) -> ("Error Out"=w342:errorcluster)  [unwired: 5 in, 2 out]
        n412 = call "VALCO_SET_POS_232.vi"("Error In"=w351, "New Position (as string)"=w345, "Valve ID"=0, "COM Port In"=w349) -> ()  [unwired: 5 in, 3 out]
        n413 = for {
          N: w338 -> [_]
          tunnel: w352 -> [w523]
          tunnel: w353 -> [w522]
          shift-right: [w521] -> w339
          shift-left: w342 -> [w533]
          n414 = local read "Reactor Valve 10 Position - Reaction"() -> (w529:string)
          n415 = call "Time Delay63"("error in (no error)"=w533, "Delay Time (s)"=1) -> ("error out"=w526:errorcluster)  [unwired: 9 in]
          n416 = call "VALCO_SET_POS_232.vi"("Error In"=w526, "New Position (as string)"=w529, "Valve ID"=w522, "COM Port In"=w523) -> ("Error Out"=w527:errorcluster, "Valve ID out"=w531:u8, "COM Port Out"=w532:refnum<visa-resource-name>)  [unwired: 5 in]
          n417 = local read "Reactor Valve 10 Position - System"() -> (w530:string)
          n418 = call "Time Delay64"("error in (no error)"=w527, "Delay Time (s)"=1) -> ("error out"=w528:errorcluster)  [unwired: 9 in]
          n419 = call "VALCO_SET_POS_232.vi"("Error In"=w528, "New Position (as string)"=w530, "Valve ID"=w531, "COM Port In"=w532) -> ("Error Out"=w521:errorcluster)  [unwired: 5 in, 2 out]
        }
        n420 = local read "Carrier Valve ID"() -> (w475:i32)
        n421 = local read "Carrier Valve Position - System"() -> (w476:string)
        n422 = local read "Carrier Valve COM"() -> (w474:refnum<visa-resource-name>)
        n423 = call "VALCO_SET_POS_232.vi"("Error In"=w457, "New Position (as string)"=w476, "Valve ID"=w475, "COM Port In"=w474) -> ("Error Out"=w477:errorcluster, "Valve ID out"=w479:u8, "COM Port Out"=w478:refnum<visa-resource-name>)  [unwired: 5 in]
        n424 = local read "Carrier Valve Position - Refill"() -> (w480:string)
        n425 = call "Time Delay11"("error in (no error)"=w477, "Delay Time (s)"=w473) -> ("error out"=w481:errorcluster)  [unwired: 9 in]
        n426 = local read "Carrier Valve Position - System"() -> (w486:string)
        n427 = call "VALCO_SET_POS_232.vi"("Error In"=w481, "New Position (as string)"=w480, "Valve ID"=w479, "COM Port In"=w478) -> ("Error Out"=w482:errorcluster, "Valve ID out"=w485:u8, "COM Port Out"=w484:refnum<visa-resource-name>)  [unwired: 5 in]
        n428 = call "Time Delay12"("error in (no error)"=w482, "Delay Time (s)"=w473) -> ("error out"=w483:errorcluster)  [unwired: 9 in]
        n429 = call "VALCO_SET_POS_232.vi"("Error In"=w483, "New Position (as string)"=w486, "Valve ID"=w485, "COM Port In"=w484) -> ()  [unwired: 5 in, 3 out]
        n430 = local read "Reactor Selector Valve\n - Upstream - COM"() -> (w462:refnum<visa-resource-name>)
        n431 = local read "Reactor Selector Valve Downstream COM"() -> (w465:refnum<visa-resource-name>)
        n432 = local read "Injection Valve COM"() -> (w471:refnum<visa-resource-name>)
        n433 = call "VALCO_OPEN.vi"("Error In (No Error)"=w339, "COM Port"=w465) -> ("Error Out"=w466:errorcluster, "COM Port (Out)"=w464:refnum<visa-resource-name>)  [unwired: 8 in]
        n434 = call "VALCO_OPEN.vi"("Error In (No Error)"=w339, "COM Port"=w462) -> ("Error Out"=w461:errorcluster, "COM Port (Out)"=w463:refnum<visa-resource-name>)  [unwired: 8 in]
        n435 = local read "Injection Valve Position - LH Needle"() -> (w468:string)
        n436 = local read "Injection Valve ID"() -> (w469:i32)
        n437 = call "VALCO_OPEN.vi"("Error In (No Error)"=w339, "COM Port"=w471) -> ("Error Out"=w467:errorcluster, "COM Port (Out)"=w470:refnum<visa-resource-name>)  [unwired: 8 in]
        n438 = call "VALCO_SET_POS_232.vi"("Error In"=w466, "New Position (as string)"=w460, "Valve ID"=0, "COM Port In"=w464) -> ("Error Out"=w337:errorcluster)  [unwired: 5 in, 2 out]
        n439 = case shown="False" FALSE {
          tunnel: w337 -> [_ w487]
          frame False {
            # "COMMENTING OUT RINSE SYRINGE PRIMING"
          }
          frame True {
            n440 = in-place {
              in-place-border: w487 -> [w488]
              in-place-border: [w488] -> _
              n441 = local read "Rinse Pump COM"() -> (w489:refnum<visa-resource-name>)
              n442 = local read "Rinse Pump ID"() -> (w490:i32)
              n443 = call "POPUP_PRIMING_NSE.vi"("Rinse Pump ID"=w490, "Rinse Pump COM"=w489) -> ()  [unwired: 2 in]
            }
          }
        }
        n444 = call "VALCO_SET_POS_232.vi"("Error In"=w461, "New Position (as string)"=w460, "Valve ID"=0, "COM Port In"=w463) -> ()  [unwired: 5 in, 3 out]
        n445 = call "VALCO_SET_POS_232.vi"("Error In"=w467, "New Position (as string)"=w468, "Valve ID"=w469, "COM Port In"=w470) -> ()  [unwired: 5 in, 3 out]
      }
      frame "Running" {
        # "Just an infinite loop while the rest of the system is running"
        n446 = while {
          tunnel: [Hardware_Initiation_Enum."Running" ("Enum")] -> w640
          stop <- w641 stop-if-true
          n447 = call "Elapsed Time"("Time Target (s)"=5.0) -> ("Time has Elapsed"=w641:bool)  [unwired: 11 in, 7 out]
        }
        n448 = local write "Ready to start schedule timer"(TRUE) -> ()
      }
    }
    n449 = local read "Stop everything"() -> (w21:bool)
  }
  n450 = case shown="True" TRUE {
    frame False {
    }
    frame True {
      # "Reactor Sequence\nThe loops below exclusively manage the temperatures of the reactors"
      n451 = while {
        shift-right: [w648] -> _
        shift-left: Reactor_Outer_Loop_Enum_NSE."Waiting for hardware initialization" ("Enum") -> [w647]
        stop <- w646 stop-if-true
        n452 = Wait (ms)(milliseconds to wait=1000) -> ()  [unwired: 1 out]
        n453 = case shown="\"Waiting for hardware initialization\", Default" w647 {
          tunnel: [w650 w699] -> w648
          frame "Waiting for hardware initialization", Default {
            w649 = FALSE
            n454 = local write "r1_done"(w649) -> ()
            n455 = local write "r2_done"(w649) -> ()
            n456 = local write "r3_done"(w649) -> ()
            n457 = local write "r4_done"(w649) -> ()
            n458 = local write "r5_done"(w649) -> ()
            n459 = local write "r6_done"(w649) -> ()
            n460 = local write "r7_done"(w649) -> ()
            n461 = local write "r8_done"(w649) -> ()
            n462 = local write "r9_done"(w649) -> ()
            n463 = local write "r10_done"(w649) -> ()
            n464 = local read "Ready to start schedule timer"() -> (w651:bool)
            n465 = case shown="True" w651 {
              tunnel: [Reactor_Outer_Loop_Enum_NSE."Waiting for hardware initialization" ("Enum") Reactor_Outer_Loop_Enum_NSE."Running" ("Enum")] -> w650
              frame False {
                n466 = Wait (ms)(milliseconds to wait=1000) -> ()  [unwired: 1 out]
              }
              frame True {
                n467 = local read "Reactor 1 enabled?"() -> (w675:bool)
                n468 = local read "Reactor 2 enabled?"() -> (w674:bool)
                n469 = local read "Reactor 3 enabled?"() -> (w673:bool)
                n470 = local read "Reactor 4 enabled?"() -> (w672:bool)
                n471 = local read "Reactor 5 enabled?"() -> (w671:bool)
                n472 = local read "Reactor 6 enabled?"() -> (w670:bool)
                n473 = local read "Reactor 7 enabled?"() -> (w669:bool)
                n474 = local read "Reactor 8 enabled?"() -> (w668:bool)
                n475 = local read "Reactor 9 enabled?"() -> (w667:bool)
                n476 = local read "Reactor 10 enabled?"() -> (w666:bool)
                n477 = case shown="True" w675 {
                  tunnel: [0.0 1.0] -> w665
                  frame False {
                  }
                  frame True {
                  }
                }
                n478 = case shown="True" w674 {
                  tunnel: [0.0 1.0] -> w664
                  frame False {
                  }
                  frame True {
                  }
                }
                n479 = case shown="True" w673 {
                  tunnel: [0.0 1.0] -> w663
                  frame False {
                  }
                  frame True {
                  }
                }
                n480 = case shown="True" w672 {
                  tunnel: [0.0 1.0] -> w662
                  frame False {
                  }
                  frame True {
                  }
                }
                n481 = case shown="True" w671 {
                  tunnel: [0.0 1.0] -> w661
                  frame False {
                  }
                  frame True {
                  }
                }
                n482 = case shown="True" w670 {
                  tunnel: [0.0 1.0] -> w660
                  frame False {
                  }
                  frame True {
                  }
                }
                n483 = case shown="True" w669 {
                  tunnel: [0.0 1.0] -> w659
                  frame False {
                  }
                  frame True {
                  }
                }
                n484 = case shown="True" w668 {
                  tunnel: [0.0 1.0] -> w658
                  frame False {
                  }
                  frame True {
                  }
                }
                n485 = case shown="True" w667 {
                  tunnel: [0.0 1.0] -> w657
                  frame False {
                  }
                  frame True {
                  }
                }
                n486 = case shown="True" w666 {
                  tunnel: [0.0 1.0] -> w656
                  frame False {
                  }
                  frame True {
                  }
                }
                n487 = local read "Schedule - Reactors"() -> (w677:dbl[][])
                n488 = script code="% reactors_start_times: N_reactors x N_rxns -- the row denotes the reactor number, the column denotes the reaction number\n% a row for a given reactor looks like: 0 0 0 17 0 0 0 0 0 0 0 0 0 0 74 0 0 0 0 0 0 0 0 0 0 0 139 0 0 0 0 0\n% this means that at t=17, \"given reactor\" needs to already be at the temperature for reaction 4. Starting at t=17, \"given reactor\" needs to remain at\n% that temperature until t=17+tau_res_time_4, then \"given reactor\" needs to start moving to the  temperature for reaction 15; starting at t=74,\n% \"given reactor\" needs to remain at that temperature until t=74+tau_res_time_15\nif r1_enabled\n    reactor_1_rxns = find(reactors_start_times(1,:)); % returns the indices corresponding to the nonzero elements in reactors_start_times(1,:); the indices are equal to the assigned reaction numbers\n    reactor_1_reaction = reactor_1_rxns(1);\nend\nif r2_enabled\n    reactor_2_rxns = find(reactors_start_times(2,:));\n    reactor_2_reaction = reactor_2_rxns(1);\nend\nif r3_enabled\n    reactor_3_rxns = find(reactors_start_times(3,:));\n    reactor_3_reaction = reactor_3_rxns(1);\nend\nif r4_enabled\n    reactor_4_rxns = find(reactors_start_times(4,:));\n    reactor_4_reaction = reactor_4_rxns(1);\nend\nif r5_enabled\n    reactor_5_rxns = find(reactors_start_times(5,:));\n    reactor_5_reaction = reactor_5_rxns(1);\nend\nif r6_enabled\n    reactor_6_rxns = find(reactors_start_times(6,:));\n    reactor_6_reaction = reactor_6_rxns(1);\nend\nif r7_enabled\n    reactor_7_rxns = find(reactors_start_times(7,:));\n   reactor_7_reaction = reactor_7_rxns(1);\nend\nif r8_enabled\n    reactor_8_rxns = find(reactors_start_times(8,:));\n    reactor_8_reaction = reactor_8_rxns(1);\nend\nif r9_enabled\n    reactor_9_rxns = find(reactors_start_times(9,:));\n    reactor_9_reaction = reactor_9_rxns(1);\nend\nif r10_enabled\n    reactor_10_rxns = find(reactors_start_times(10,:));\n    reactor_10_reaction = reactor_10_rxns(1);\nend"("??"=errorcluster {"status"=FALSE, "code"=0, "source"=""} ("error constant"), "reactors_start_times"=w677, "r1_enabled"=w665, "r2_enabled"=w664, "r3_enabled"=w663, "r4_enabled"=w662, "r5_enabled"=w661, "r6_enabled"=w660, "r7_enabled"=w659, "r8_enabled"=w658, "r9_enabled"=w657, "r10_enabled"=w656) -> ("??"=w655:errorcluster)
                "reaction scheduling error" <- w655
                n489 = Unbundle By Name(w655) -> ("status"=w654:bool)
                n490 = local write "Reaction scheduling error"(w654) -> ()
              }
            }
          }
          frame "Running" {
            # "While loop that reads the temperature of each enabled reactor so those temperatures can be displayed on the front panel"
            n491 = local read "Reactor 4 enabled?"() -> (w705:bool)
            n492 = local read "Reactor 2 enabled?"() -> (w703:bool)
            n493 = local read "Reactor 1 enabled?"() -> (w702:bool)
            n494 = local read "Reactor 5 enabled?"() -> (w706:bool)
            n495 = local read "Reactor 10 enabled?"() -> (w711:bool)
            n496 = local read "Reactor 3 enabled?"() -> (w704:bool)
            n497 = local read "Reactor 6 enabled?"() -> (w707:bool)
            n498 = local read "Reactor 9 enabled?"() -> (w710:bool)
            n499 = local read "Reactor 8 enabled?"() -> (w709:bool)
            n500 = local read "Reactor 7 enabled?"() -> (w708:bool)
            n501 = case shown="True" w702 {
              frame False {
              }
              frame True {
                # "Reactor 1"
                n502 = while {
                  shift-right: [w1070] -> _
                  shift-left: Reactors_Enum_NSE."Getting next assignment" ("Enum") -> [w1069]
                  stop <- w1068 stop-if-true
                  n503 = case shown="\"Done\"" w1069 {
                    tunnel: [w1077 Reactors_Enum_NSE."Getting next assignment" ("Enum") Reactors_Enum_NSE."Done" ("Enum")] -> w1070
                    frame "Getting next assignment", Default {
                      n504 = local read "Temperature Control Error - Reactor 1"() -> (w1072:errorcluster)
                      n505 = script code="% Get the index for the next reaction along with its start time, temperature, and residence time\nif ~isempty(reactor_1_rxns)\n     reactor_1_done = 0;\n     reactor_1_reaction = reactor_1_rxns(1);\n     reactor_1_start_time = reactors_start_times(1, reactor_1_reaction);\n     reactor_1_temperature_C = all_slugs(reactor_1_reaction).temperature;\n     reactor_1_res_time = all_slugs(reactor_1_reaction).residence_time_goal;\n     % convert temperature to degF and string for Watlow\n     reactor_1_temperature_F = num2str((reactor_1_temperature_C * 1.8) + 32);\nelse\n     reactor_1_done = 1;\nend"("??"=w1072) -> ("??"=w1076:errorcluster, "reactor_1_start_time"=→"r1_start_time":dbl, "reactor_1_temperature_F"=→"r1_temp_F":string, "reactor_1_res_time"=→"r1_res_time":dbl, "reactor_1_done"=w1075:dbl)
                      n506 = Greater?(x=w1075, y=0.0) -> (0:w1073:bool)
                      n507 = case shown="True" w1073 {
                        tunnel: [Reactors_Enum_NSE."Running" ("Enum") Reactors_Enum_NSE."Done" ("Enum")] -> w1077
                        tunnel: w1076 -> [w1082 w1092]
                        tunnel: [w1081 w1089] -> w1071
                        frame False {
                          w1084 = u16 7001 items=["Read temperature (F)"=4001, "Read setpoint (F)"=8029, "Write setpoint (F)"=7001, "Read autotune status"=8027, "Write start autotune"=8026]
                          n508 = local read "Watlow COM"() -> (w1085:refnum<visa-resource-name>)
                          n509 = local read "Watlow Zone - Reactor 1"() -> (w1086:dbl)
                          n510 = local read "Watlow Instance - Reactor 1"() -> (w1087:dbl)
                          n511 = local read "r1_temp_F"() -> (w1083:string)
                          n512 = call "Write.vi"("PC Comms Port"=w1085, "Zone"=w1086, "Parameter"=w1084, "Instance"=w1087, "Write Value"=w1083, "Error In"=w1082) -> ("Error Out"=w1081:errorcluster)  [unwired: 13 in]
                        }
                        frame True {
                          w1093 = u16 7001 items=["Read temperature (F)"=4001, "Read setpoint (F)"=8029, "Write setpoint (F)"=7001, "Read autotune status"=8027, "Write start autotune"=8026]
                          # "Reactor is done for now.\nWrite a low set point to cool it down"
                          n513 = local read "Watlow COM"() -> (w1094:refnum<visa-resource-name>)
                          n514 = local read "Watlow Zone - Reactor 1"() -> (w1095:dbl)
                          n515 = local read "Watlow Instance - Reactor 1"() -> (w1096:dbl)
                          n516 = local write "r1_done"(TRUE) -> ()
                          n517 = call "Write.vi"("PC Comms Port"=w1094, "Zone"=w1095, "Parameter"=w1093, "Instance"=w1096, "Write Value"="50", "Error In"=w1092) -> ("Error Out"=w1089:errorcluster)  [unwired: 13 in]
                        }
                      }
                      n518 = local write "Temperature Control Error - Reactor 1"(w1071) -> ()
                    }
                    frame "Running" {
                      n519 = while {
                        stop <- w1099 stop-if-true
                        # "Once the master time exceeds\nthe current start time plus the\ncurrent residence time, stop\nand go back to get the next\nassignment"
                        n520 = local read "r1_start_time"() -> (w1104:dbl)
                        n521 = local read "r1_res_time"() -> (w1103:dbl)
                        n522 = local read "Master time [s]"() -> (w1101:dbl)
                        n523 = Add(x=w1104, y=w1103) -> (x+y=w1102:dbl)
                        n524 = Greater?(x=w1101, y=w1102) -> (0:w1100:bool)
                        n525 = case shown="True" w1100 {
                          selector: w1100 -> [w1105 w1108]
                          tunnel: [w1105 w1108] -> w1099
                          frame False {
                            n526 = Wait (ms)(milliseconds to wait=500) -> ()  [unwired: 1 out]
                          }
                          frame True {
                            n527 = script code="reactor_1_rxns(1) = []; % remove the reaction index that just ran"("??"=errorcluster {"status"=FALSE, "code"=0, "source"=""} ("error constant")) -> ()  [unwired: 1 out]
                          }
                        }
                      }
                    }
                    frame "Done" {
                    }
                  }
                  n528 = Wait (ms)(milliseconds to wait=1000) -> ()  [unwired: 1 out]
                  n529 = local read "r1_done"() -> (w1068:bool)
                }
              }
            }
            n530 = case shown="True" w703 {
              frame False {
              }
              frame True {
                # "Reactor 2"
                n531 = while {
                  shift-right: [w1026] -> _
                  shift-left: Reactors_Enum_NSE."Getting next assignment" ("Enum") -> [w1025]
                  stop <- w1023 stop-if-true
                  n532 = case shown="\"Getting next assignment\", Default" w1025 {
                    tunnel: [w1033 Reactors_Enum_NSE."Getting next assignment" ("Enum") Reactors_Enum_NSE."Done" ("Enum")] -> w1026
                    frame "Getting next assignment", Default {
                      n533 = local read "Temperature Control Error - Reactor 2"() -> (w1028:errorcluster)
                      n534 = script code="% Get the index for the next reaction along with its start time, temperature, and residence time\nif ~isempty(reactor_2_rxns)\n     reactor_2_done = 0;\n     reactor_2_reaction = reactor_2_rxns(1);\n     reactor_2_start_time = reactors_start_times(2, reactor_2_reaction);\n     reactor_2_temperature_C = all_slugs(reactor_2_reaction).temperature;\n     reactor_2_res_time = all_slugs(reactor_2_reaction).residence_time_goal;\n     % convert temperature to degF and string for Watlow\n     reactor_2_temperature_F = num2str((reactor_2_temperature_C * 1.8) + 32);\nelse\n     reactor_2_done = 1;\nend"("??"=w1028) -> ("??"=w1032:errorcluster, "reactor_2_start_time"=→"r2_start_time":dbl, "reactor_2_temperature_F"=→"r2_temp_F":string, "reactor_2_res_time"=→"r2_res_time":dbl, "reactor_2_done"=w1031:dbl)
                      n535 = Greater?(x=w1031, y=0.0) -> (0:w1029:bool)
                      n536 = case shown="True" w1029 {
                        tunnel: [Reactors_Enum_NSE."Running" ("Enum") Reactors_Enum_NSE."Done" ("Enum")] -> w1033
                        tunnel: w1032 -> [w1038 w1048]
                        tunnel: [w1037 w1045] -> w1027
                        frame False {
                          w1040 = u16 7001 items=["Read temperature (F)"=4001, "Read setpoint (F)"=8029, "Write setpoint (F)"=7001, "Read autotune status"=8027, "Write start autotune"=8026]
                          n537 = local read "Watlow COM"() -> (w1041:refnum<visa-resource-name>)
                          n538 = local read "Watlow Zone - Reactor 2"() -> (w1042:dbl)
                          n539 = local read "Watlow Instance - Reactor 2"() -> (w1043:dbl)
                          n540 = local read "r2_temp_F"() -> (w1039:string)
                          n541 = call "Write.vi"("PC Comms Port"=w1041, "Zone"=w1042, "Parameter"=w1040, "Instance"=w1043, "Write Value"=w1039, "Error In"=w1038) -> ("Error Out"=w1037:errorcluster)  [unwired: 13 in]
                        }
                        frame True {
                          w1049 = u16 7001 items=["Read temperature (F)"=4001, "Read setpoint (F)"=8029, "Write setpoint (F)"=7001, "Read autotune status"=8027, "Write start autotune"=8026]
                          # "Reactor is done for now.\nWrite a low set point to cool it down"
                          n542 = local read "Watlow COM"() -> (w1050:refnum<visa-resource-name>)
                          n543 = local read "Watlow Zone - Reactor 2"() -> (w1051:dbl)
                          n544 = local read "Watlow Instance - Reactor 2"() -> (w1052:dbl)
                          n545 = local write "r2_done"(TRUE) -> ()
                          n546 = call "Write.vi"("PC Comms Port"=w1050, "Zone"=w1051, "Parameter"=w1049, "Instance"=w1052, "Write Value"="50", "Error In"=w1048) -> ("Error Out"=w1045:errorcluster)  [unwired: 13 in]
                        }
                      }
                      n547 = local write "Temperature Control Error - Reactor 2"(w1027) -> ()
                    }
                    frame "Running" {
                      n548 = while {
                        stop <- w1055 stop-if-true
                        # "Once the master time exceeds\nthe current start time plus the\ncurrent residence time, stop\nand go back to get the next\nassignment"
                        n549 = local read "r2_start_time"() -> (w1060:dbl)
                        n550 = local read "r2_res_time"() -> (w1059:dbl)
                        n551 = local read "Master time [s]"() -> (w1057:dbl)
                        n552 = Add(x=w1060, y=w1059) -> (x+y=w1058:dbl)
                        n553 = Greater?(x=w1057, y=w1058) -> (0:w1056:bool)
                        n554 = case shown="True" w1056 {
                          selector: w1056 -> [w1061 w1064]
                          tunnel: [w1061 w1064] -> w1055
                          frame False {
                            n555 = Wait (ms)(milliseconds to wait=500) -> ()  [unwired: 1 out]
                          }
                          frame True {
                            n556 = script code="reactor_2_rxns(1) = []; % remove the reaction index that just ran"("??"=errorcluster {"status"=FALSE, "code"=0, "source"=""} ("error constant")) -> ()  [unwired: 1 out]
                          }
                        }
                      }
                    }
                    frame "Done" {
                    }
                  }
                  n557 = Wait (ms)(milliseconds to wait=1000) -> ()  [unwired: 1 out]
                  n558 = local read "r2_done"() -> (w1023:bool)
                }
              }
            }
            n559 = case shown="True" w704 {
              frame False {
              }
              frame True {
                # "Reactor 3"
                n560 = while {
                  shift-right: [w982] -> _
                  shift-left: Reactors_Enum_NSE."Getting next assignment" ("Enum") -> [w981]
                  stop <- w980 stop-if-true
                  n561 = case shown="\"Getting next assignment\", Default" w981 {
                    tunnel: [w989 Reactors_Enum_NSE."Getting next assignment" ("Enum") Reactors_Enum_NSE."Done" ("Enum")] -> w982
                    frame "Getting next assignment", Default {
                      n562 = local read "Temperature Control Error - Reactor 3"() -> (w984:errorcluster)
                      n563 = script code="% Get the index for the next reaction along with its start time, temperature, and residence time\nif ~isempty(reactor_3_rxns)\n     reactor_3_done = 0;\n     reactor_3_reaction = reactor_3_rxns(1);\n     reactor_3_start_time = reactors_start_times(3, reactor_3_reaction);\n     reactor_3_temperature_C = all_slugs(reactor_3_reaction).temperature;\n     reactor_3_res_time = all_slugs(reactor_3_reaction).residence_time_goal;\n     % convert temperature to degF and string for Watlow\n     reactor_3_temperature_F = num2str((reactor_3_temperature_C * 1.8) + 32);\nelse\n     reactor_3_done = 1;\nend"("??"=w984) -> ("??"=w988:errorcluster, "reactor_3_start_time"=→"r3_start_time":dbl, "reactor_3_temperature_F"=→"r3_temp_F":string, "reactor_3_res_time"=→"r3_res_time":dbl, "reactor_3_done"=w987:dbl)
                      n564 = Greater?(x=w987, y=0.0) -> (0:w985:bool)
                      n565 = case shown="True" w985 {
                        tunnel: [Reactors_Enum_NSE."Running" ("Enum") Reactors_Enum_NSE."Done" ("Enum")] -> w989
                        tunnel: w988 -> [w994 w1004]
                        tunnel: [w993 w1001] -> w983
                        frame False {
                          w996 = u16 7001 items=["Read temperature (F)"=4001, "Read setpoint (F)"=8029, "Write setpoint (F)"=7001, "Read autotune status"=8027, "Write start autotune"=8026]
                          n566 = local read "Watlow COM"() -> (w997:refnum<visa-resource-name>)
                          n567 = local read "Watlow Zone - Reactor 3"() -> (w998:dbl)
                          n568 = local read "Watlow Instance - Reactor 3"() -> (w999:dbl)
                          n569 = local read "r3_temp_F"() -> (w995:string)
                          n570 = call "Write.vi"("PC Comms Port"=w997, "Zone"=w998, "Parameter"=w996, "Instance"=w999, "Write Value"=w995, "Error In"=w994) -> ("Error Out"=w993:errorcluster)  [unwired: 13 in]
                        }
                        frame True {
                          w1005 = u16 7001 items=["Read temperature (F)"=4001, "Read setpoint (F)"=8029, "Write setpoint (F)"=7001, "Read autotune status"=8027, "Write start autotune"=8026]
                          # "Reactor is done for now.\nWrite a low set point to cool it down"
                          n571 = local read "Watlow COM"() -> (w1006:refnum<visa-resource-name>)
                          n572 = local read "Watlow Zone - Reactor 3"() -> (w1007:dbl)
                          n573 = local read "Watlow Instance - Reactor 3"() -> (w1008:dbl)
                          n574 = local write "r3_done"(TRUE) -> ()
                          n575 = call "Write.vi"("PC Comms Port"=w1006, "Zone"=w1007, "Parameter"=w1005, "Instance"=w1008, "Write Value"="50", "Error In"=w1004) -> ("Error Out"=w1001:errorcluster)  [unwired: 13 in]
                        }
                      }
                      n576 = local write "Temperature Control Error - Reactor 3"(w983) -> ()
                    }
                    frame "Running" {
                      n577 = while {
                        stop <- w1011 stop-if-true
                        # "Once the master time exceeds\nthe current start time plus the\ncurrent residence time, stop\nand go back to get the next\nassignment"
                        n578 = local read "r3_start_time"() -> (w1016:dbl)
                        n579 = local read "r3_res_time"() -> (w1015:dbl)
                        n580 = local read "Master time [s]"() -> (w1013:dbl)
                        n581 = Add(x=w1016, y=w1015) -> (x+y=w1014:dbl)
                        n582 = Greater?(x=w1013, y=w1014) -> (0:w1012:bool)
                        n583 = case shown="True" w1012 {
                          selector: w1012 -> [w1017 w1020]
                          tunnel: [w1017 w1020] -> w1011
                          frame False {
                            n584 = Wait (ms)(milliseconds to wait=500) -> ()  [unwired: 1 out]
                          }
                          frame True {
                            n585 = script code="reactor_3_rxns(1) = []; % remove the reaction index that just ran"("??"=errorcluster {"status"=FALSE, "code"=0, "source"=""} ("error constant")) -> ()  [unwired: 1 out]
                          }
                        }
                      }
                    }
                    frame "Done" {
                    }
                  }
                  n586 = Wait (ms)(milliseconds to wait=1000) -> ()  [unwired: 1 out]
                  n587 = local read "r3_done"() -> (w980:bool)
                }
              }
            }
            n588 = case shown="True" w705 {
              frame False {
              }
              frame True {
                # "Reactor 4"
                n589 = while {
                  shift-right: [w938] -> _
                  shift-left: Reactors_Enum_NSE."Getting next assignment" ("Enum") -> [w937]
                  stop <- w936 stop-if-true
                  n590 = case shown="\"Done\"" w937 {
                    tunnel: [w945 Reactors_Enum_NSE."Getting next assignment" ("Enum") Reactors_Enum_NSE."Done" ("Enum")] -> w938
                    frame "Getting next assignment", Default {
                      n591 = local read "Temperature Control Error - Reactor 4"() -> (w940:errorcluster)
                      n592 = script code="% Get the index for the next reaction along with its start time, temperature, and residence time\nif ~isempty(reactor_4_rxns)\n     reactor_4_done = 0;\n     reactor_4_reaction = reactor_4_rxns(1);\n     reactor_4_start_time = reactors_start_times(4, reactor_4_reaction);\n     reactor_4_temperature_C = all_slugs(reactor_4_reaction).temperature;\n     reactor_4_res_time = all_slugs(reactor_4_reaction).residence_time_goal;\n     % convert temperature to degF and string for Watlow\n     reactor_4_temperature_F = num2str((reactor_4_temperature_C * 1.8) + 32);\nelse\n     reactor_4_done = 1;\nend"("??"=w940) -> ("??"=w944:errorcluster, "reactor_4_start_time"=→"r4_start_time":dbl, "reactor_4_temperature_F"=→"r4_temp_F":string, "reactor_4_res_time"=→"r4_res_time":dbl, "reactor_4_done"=w943:dbl)
                      n593 = Greater?(x=w943, y=0.0) -> (0:w941:bool)
                      n594 = case shown="False" w941 {
                        tunnel: [Reactors_Enum_NSE."Running" ("Enum") Reactors_Enum_NSE."Done" ("Enum")] -> w945
                        tunnel: w944 -> [w950 w960]
                        tunnel: [w949 w957] -> w939
                        frame False {
                          w952 = u16 7001 items=["Read temperature (F)"=4001, "Read setpoint (F)"=8029, "Write setpoint (F)"=7001, "Read autotune status"=8027, "Write start autotune"=8026]
                          n595 = local read "Watlow COM"() -> (w953:refnum<visa-resource-name>)
                          n596 = local read "Watlow Zone - Reactor 4"() -> (w954:dbl)
                          n597 = local read "Watlow Instance - Reactor 4"() -> (w955:dbl)
                          n598 = local read "r4_temp_F"() -> (w951:string)
                          n599 = call "Write.vi"("PC Comms Port"=w953, "Zone"=w954, "Parameter"=w952, "Instance"=w955, "Write Value"=w951, "Error In"=w950) -> ("Error Out"=w949:errorcluster)  [unwired: 13 in]
                        }
                        frame True {
                          w961 = u16 7001 items=["Read temperature (F)"=4001, "Read setpoint (F)"=8029, "Write setpoint (F)"=7001, "Read autotune status"=8027, "Write start autotune"=8026]
                          # "Reactor is done for now.\nWrite a low set point to cool it down"
                          n600 = local read "Watlow COM"() -> (w962:refnum<visa-resource-name>)
                          n601 = local read "Watlow Zone - Reactor 4"() -> (w963:dbl)
                          n602 = local read "Watlow Instance - Reactor 4"() -> (w964:dbl)
                          n603 = local write "r4_done"(TRUE) -> ()
                          n604 = call "Write.vi"("PC Comms Port"=w962, "Zone"=w963, "Parameter"=w961, "Instance"=w964, "Write Value"="50", "Error In"=w960) -> ("Error Out"=w957:errorcluster)  [unwired: 13 in]
                        }
                      }
                      n605 = local write "Temperature Control Error - Reactor 4"(w939) -> ()
                    }
                    frame "Running" {
                      n606 = while {
                        stop <- w967 stop-if-true
                        # "Once the master time exceeds\nthe current start time plus the\ncurrent residence time, stop\nand go back to get the next\nassignment"
                        n607 = local read "r4_start_time"() -> (w972:dbl)
                        n608 = local read "r4_res_time"() -> (w971:dbl)
                        n609 = local read "Master time [s]"() -> (w969:dbl)
                        n610 = Add(x=w972, y=w971) -> (x+y=w970:dbl)
                        n611 = Greater?(x=w969, y=w970) -> (0:w968:bool)
                        n612 = case shown="False" w968 {
                          selector: w968 -> [w973 w976]
                          tunnel: [w973 w976] -> w967
                          frame False {
                            n613 = Wait (ms)(milliseconds to wait=500) -> ()  [unwired: 1 out]
                          }
                          frame True {
                            n614 = script code="reactor_4_rxns(1) = []; % remove the reaction index that just ran"("??"=errorcluster {"status"=FALSE, "code"=0, "source"=""} ("error constant")) -> ()  [unwired: 1 out]
                          }
                        }
                      }
                    }
                    frame "Done" {
                    }
                  }
                  n615 = Wait (ms)(milliseconds to wait=1000) -> ()  [unwired: 1 out]
                  n616 = local read "r4_done"() -> (w936:bool)
                }
              }
            }
            n617 = case shown="True" w706 {
              frame False {
              }
              frame True {
                # "Reactor 5"
                n618 = while {
                  shift-right: [w894] -> _
                  shift-left: Reactors_Enum_NSE."Getting next assignment" ("Enum") -> [w893]
                  stop <- w892 stop-if-true
                  n619 = case shown="\"Running\"" w893 {
                    tunnel: [w901 Reactors_Enum_NSE."Getting next assignment" ("Enum") Reactors_Enum_NSE."Done" ("Enum")] -> w894
                    frame "Getting next assignment", Default {
                      n620 = local read "Temperature Control Error - Reactor 5"() -> (w896:errorcluster)
                      n621 = script code="% Get the index for the next reaction along with its start time, temperature, and residence time\nif ~isempty(reactor_5_rxns)\n     reactor_5_done = 0;\n     reactor_5_reaction = reactor_5_rxns(1);\n     reactor_5_start_time = reactors_start_times(5, reactor_5_reaction);\n     reactor_5_temperature_C = all_slugs(reactor_5_reaction).temperature;\n     reactor_5_res_time = all_slugs(reactor_5_reaction).residence_time_goal;\n     % convert temperature to degF and string for Watlow\n     reactor_5_temperature_F = num2str((reactor_5_temperature_C * 1.8) + 32);\nelse\n     reactor_5_done = 1;\nend"("??"=w896) -> ("??"=w900:errorcluster, "reactor_5_start_time"=→"r5_start_time":dbl, "reactor_5_temperature_F"=→"r5_temp_F":string, "reactor_5_res_time"=→"r5_res_time":dbl, "reactor_5_done"=w899:dbl)
                      n622 = Greater?(x=w899, y=0.0) -> (0:w897:bool)
                      n623 = case shown="True" w897 {
                        tunnel: [Reactors_Enum_NSE."Running" ("Enum") Reactors_Enum_NSE."Done" ("Enum")] -> w901
                        tunnel: w900 -> [w906 w916]
                        tunnel: [w905 w913] -> w895
                        frame False {
                          w908 = u16 7001 items=["Read temperature (F)"=4001, "Read setpoint (F)"=8029, "Write setpoint (F)"=7001, "Read autotune status"=8027, "Write start autotune"=8026]
                          n624 = local read "Watlow COM"() -> (w909:refnum<visa-resource-name>)
                          n625 = local read "Watlow Zone - Reactor 5"() -> (w910:dbl)
                          n626 = local read "Watlow Instance - Reactor 5"() -> (w911:dbl)
                          n627 = local read "r5_temp_F"() -> (w907:string)
                          n628 = call "Write.vi"("PC Comms Port"=w909, "Zone"=w910, "Parameter"=w908, "Instance"=w911, "Write Value"=w907, "Error In"=w906) -> ("Error Out"=w905:errorcluster)  [unwired: 13 in]
                        }
                        frame True {
                          w917 = u16 7001 items=["Read temperature (F)"=4001, "Read setpoint (F)"=8029, "Write setpoint (F)"=7001, "Read autotune status"=8027, "Write start autotune"=8026]
                          # "Reactor is done for now.\nWrite a low set point to cool it down"
                          n629 = local read "Watlow COM"() -> (w918:refnum<visa-resource-name>)
                          n630 = local read "Watlow Zone - Reactor 5"() -> (w919:dbl)
                          n631 = local read "Watlow Instance - Reactor 5"() -> (w920:dbl)
                          n632 = local write "r5_done"(TRUE) -> ()
                          n633 = call "Write.vi"("PC Comms Port"=w918, "Zone"=w919, "Parameter"=w917, "Instance"=w920, "Write Value"="50", "Error In"=w916) -> ("Error Out"=w913:errorcluster)  [unwired: 13 in]
                        }
                      }
                      n634 = local write "Temperature Control Error - Reactor 5"(w895) -> ()
                    }
                    frame "Running" {
                      n635 = while {
                        stop <- w923 stop-if-true
                        # "Once the master time exceeds\nthe current start time plus the\ncurrent residence time, stop\nand go back to get the next\nassignment"
                        n636 = local read "r5_start_time"() -> (w928:dbl)
                        n637 = local read "r5_res_time"() -> (w927:dbl)
                        n638 = local read "Master time [s]"() -> (w925:dbl)
                        n639 = Add(x=w928, y=w927) -> (x+y=w926:dbl)
                        n640 = Greater?(x=w925, y=w926) -> (0:w924:bool)
                        n641 = case shown="True" w924 {
                          selector: w924 -> [w929 w932]
                          tunnel: [w929 w932] -> w923
                          frame False {
                            n642 = Wait (ms)(milliseconds to wait=500) -> ()  [unwired: 1 out]
                          }
                          frame True {
                            n643 = script code="reactor_5_rxns(1) = []; % remove the reaction index that just ran"("??"=errorcluster {"status"=FALSE, "code"=0, "source"=""} ("error constant")) -> ()  [unwired: 1 out]
                          }
                        }
                      }
                    }
                    frame "Done" {
                    }
                  }
                  n644 = Wait (ms)(milliseconds to wait=1000) -> ()  [unwired: 1 out]
                  n645 = local read "r5_done"() -> (w892:bool)
                }
              }
            }
            n646 = case shown="True" w707 {
              frame False {
              }
              frame True {
                # "Reactor 6"
                n647 = while {
                  shift-right: [w850] -> _
                  shift-left: Reactors_Enum_NSE."Getting next assignment" ("Enum") -> [w849]
                  stop <- w848 stop-if-true
                  n648 = case shown="\"Getting next assignment\", Default" w849 {
                    tunnel: [w857 Reactors_Enum_NSE."Getting next assignment" ("Enum") Reactors_Enum_NSE."Done" ("Enum")] -> w850
                    frame "Getting next assignment", Default {
                      n649 = local read "Temperature Control Error - Reactor 6"() -> (w852:errorcluster)
                      n650 = script code="% Get the index for the next reaction along with its start time, temperature, and residence time\nif ~isempty(reactor_6_rxns)\n     reactor_6_done = 0;\n     reactor_6_reaction = reactor_6_rxns(1);\n     reactor_6_start_time = reactors_start_times(6, reactor_6_reaction);\n     reactor_6_temperature_C = all_slugs(reactor_6_reaction).temperature;\n     reactor_6_res_time = all_slugs(reactor_6_reaction).residence_time_goal;\n     % convert temperature to degF and string for Watlow\n     reactor_6_temperature_F = num2str((reactor_6_temperature_C * 1.8) + 32);\nelse\n     reactor_6_done = 1;\nend"("??"=w852) -> ("??"=w856:errorcluster, "reactor_6_start_time"=→"r6_start_time":dbl, "reactor_6_temperature_F"=→"r6_temp_F":string, "reactor_6_res_time"=→"r6_res_time":dbl, "reactor_6_done"=w855:dbl)
                      n651 = Greater?(x=w855, y=0.0) -> (0:w853:bool)
                      n652 = case shown="False" w853 {
                        tunnel: [Reactors_Enum_NSE."Running" ("Enum") Reactors_Enum_NSE."Done" ("Enum")] -> w857
                        tunnel: w856 -> [w862 w872]
                        tunnel: [w861 w869] -> w851
                        frame False {
                          w864 = u16 7001 items=["Read temperature (F)"=4001, "Read setpoint (F)"=8029, "Write setpoint (F)"=7001, "Read autotune status"=8027, "Write start autotune"=8026]
                          n653 = local read "Watlow COM"() -> (w865:refnum<visa-resource-name>)
                          n654 = local read "Watlow Zone - Reactor 6"() -> (w866:dbl)
                          n655 = local read "Watlow Instance - Reactor 6"() -> (w867:dbl)
                          n656 = local read "r6_temp_F"() -> (w863:string)
                          n657 = call "Write.vi"("PC Comms Port"=w865, "Zone"=w866, "Parameter"=w864, "Instance"=w867, "Write Value"=w863, "Error In"=w862) -> ("Error Out"=w861:errorcluster)  [unwired: 13 in]
                        }
                        frame True {
                          w873 = u16 7001 items=["Read temperature (F)"=4001, "Read setpoint (F)"=8029, "Write setpoint (F)"=7001, "Read autotune status"=8027, "Write start autotune"=8026]
                          # "Reactor is done for now.\nWrite a low set point to cool it down"
                          n658 = local read "Watlow COM"() -> (w874:refnum<visa-resource-name>)
                          n659 = local read "Watlow Zone - Reactor 6"() -> (w875:dbl)
                          n660 = local read "Watlow Instance - Reactor 6"() -> (w876:dbl)
                          n661 = local write "r6_done"(TRUE) -> ()
                          n662 = call "Write.vi"("PC Comms Port"=w874, "Zone"=w875, "Parameter"=w873, "Instance"=w876, "Write Value"="50", "Error In"=w872) -> ("Error Out"=w869:errorcluster)  [unwired: 13 in]
                        }
                      }
                      n663 = local write "Temperature Control Error - Reactor 6"(w851) -> ()
                    }
                    frame "Running" {
                      n664 = while {
                        stop <- w879 stop-if-true
                        # "Once the master time exceeds\nthe current start time plus the\ncurrent residence time, stop\nand go back to get the next\nassignment"
                        n665 = local read "r6_start_time"() -> (w884:dbl)
                        n666 = local read "r6_res_time"() -> (w883:dbl)
                        n667 = local read "Master time [s]"() -> (w881:dbl)
                        n668 = Add(x=w884, y=w883) -> (x+y=w882:dbl)
                        n669 = Greater?(x=w881, y=w882) -> (0:w880:bool)
                        n670 = case shown="False" w880 {
                          selector: w880 -> [w885 w888]
                          tunnel: [w885 w888] -> w879
                          frame False {
                            n671 = Wait (ms)(milliseconds to wait=500) -> ()  [unwired: 1 out]
                          }
                          frame True {
                            n672 = script code="reactor_6_rxns(1) = []; % remove the reaction index that just ran"("??"=errorcluster {"status"=FALSE, "code"=0, "source"=""} ("error constant")) -> ()  [unwired: 1 out]
                          }
                        }
                      }
                    }
                    frame "Done" {
                    }
                  }
                  n673 = Wait (ms)(milliseconds to wait=1000) -> ()  [unwired: 1 out]
                  n674 = local read "r6_done"() -> (w848:bool)
                }
              }
            }
            n675 = case shown="True" w708 {
              frame False {
              }
              frame True {
                # "Reactor 7"
                n676 = while {
                  shift-right: [w806] -> _
                  shift-left: Reactors_Enum_NSE."Getting next assignment" ("Enum") -> [w805]
                  stop <- w804 stop-if-true
                  n677 = case shown="\"Getting next assignment\", Default" w805 {
                    tunnel: [w813 Reactors_Enum_NSE."Getting next assignment" ("Enum") Reactors_Enum_NSE."Done" ("Enum")] -> w806
                    frame "Getting next assignment", Default {
                      n678 = local read "Temperature Control Error - Reactor 7"() -> (w808:errorcluster)
                      n679 = script code="% Get the index for the next reaction along with its start time, temperature, and residence time\nif ~isempty(reactor_7_rxns)\n     reactor_7_done = 0;\n     reactor_7_reaction = reactor_7_rxns(1);\n     reactor_7_start_time = reactors_start_times(7, reactor_7_reaction);\n     reactor_7_temperature_C = all_slugs(reactor_7_reaction).temperature;\n     reactor_7_res_time = all_slugs(reactor_7_reaction).residence_time_goal;\n     % convert temperature to degF and string for Watlow\n     reactor_7_temperature_F = num2str((reactor_7_temperature_C * 1.8) + 32);\nelse\n     reactor_7_done = 1;\nend"("??"=w808) -> ("??"=w812:errorcluster, "reactor_7_start_time"=→"r7_start_time":dbl, "reactor_7_temperature_F"=→"r7_temp_F":string, "reactor_7_res_time"=→"r7_res_time":dbl, "reactor_7_done"=w811:dbl)
                      n680 = Greater?(x=w811, y=0.0) -> (0:w809:bool)
                      n681 = case shown="False" w809 {
                        tunnel: [Reactors_Enum_NSE."Running" ("Enum") Reactors_Enum_NSE."Done" ("Enum")] -> w813
                        tunnel: w812 -> [w818 w828]
                        tunnel: [w817 w825] -> w807
                        frame False {
                          w820 = u16 7001 items=["Read temperature (F)"=4001, "Read setpoint (F)"=8029, "Write setpoint (F)"=7001, "Read autotune status"=8027, "Write start autotune"=8026]
                          n682 = local read "Watlow COM"() -> (w821:refnum<visa-resource-name>)
                          n683 = local read "Watlow Zone - Reactor 7"() -> (w822:dbl)
                          n684 = local read "Watlow Instance - Reactor 7"() -> (w823:dbl)
                          n685 = local read "r7_temp_F"() -> (w819:string)
                          n686 = call "Write.vi"("PC Comms Port"=w821, "Zone"=w822, "Parameter"=w820, "Instance"=w823, "Write Value"=w819, "Error In"=w818) -> ("Error Out"=w817:errorcluster)  [unwired: 13 in]
                        }
                        frame True {
                          w829 = u16 7001 items=["Read temperature (F)"=4001, "Read setpoint (F)"=8029, "Write setpoint (F)"=7001, "Read autotune status"=8027, "Write start autotune"=8026]
                          # "Reactor is done for now.\nWrite a low set point to cool it down"
                          n687 = local read "Watlow COM"() -> (w830:refnum<visa-resource-name>)
                          n688 = local read "Watlow Zone - Reactor 7"() -> (w831:dbl)
                          n689 = local read "Watlow Instance - Reactor 7"() -> (w832:dbl)
                          n690 = local write "r7_done"(TRUE) -> ()
                          n691 = call "Write.vi"("PC Comms Port"=w830, "Zone"=w831, "Parameter"=w829, "Instance"=w832, "Write Value"="50", "Error In"=w828) -> ("Error Out"=w825:errorcluster)  [unwired: 13 in]
                        }
                      }
                      n692 = local write "Temperature Control Error - Reactor 7"(w807) -> ()
                    }
                    frame "Running" {
                      n693 = while {
                        stop <- w835 stop-if-true
                        # "Once the master time exceeds\nthe current start time plus the\ncurrent residence time, stop\nand go back to get the next\nassignment"
                        n694 = local read "r7_start_time"() -> (w840:dbl)
                        n695 = local read "r7_res_time"() -> (w839:dbl)
                        n696 = local read "Master time [s]"() -> (w837:dbl)
                        n697 = Add(x=w840, y=w839) -> (x+y=w838:dbl)
                        n698 = Greater?(x=w837, y=w838) -> (0:w836:bool)
                        n699 = case shown="False" w836 {
                          selector: w836 -> [w841 w844]
                          tunnel: [w841 w844] -> w835
                          frame False {
                            n700 = Wait (ms)(milliseconds to wait=500) -> ()  [unwired: 1 out]
                          }
                          frame True {
                            n701 = script code="reactor_7_rxns(1) = []; % remove the reaction index that just ran"("??"=errorcluster {"status"=FALSE, "code"=0, "source"=""} ("error constant")) -> ()  [unwired: 1 out]
                          }
                        }
                      }
                    }
                    frame "Done" {
                    }
                  }
                  n702 = Wait (ms)(milliseconds to wait=1000) -> ()  [unwired: 1 out]
                  n703 = local read "r7_done"() -> (w804:bool)
                }
              }
            }
            n704 = case shown="True" w709 {
              frame False {
              }
              frame True {
                # "Reactor 8"
                n705 = while {
                  shift-right: [w762] -> _
                  shift-left: Reactors_Enum_NSE."Getting next assignment" ("Enum") -> [w761]
                  stop <- w760 stop-if-true
                  n706 = case shown="\"Getting next assignment\", Default" w761 {
                    tunnel: [w769 Reactors_Enum_NSE."Getting next assignment" ("Enum") Reactors_Enum_NSE."Done" ("Enum")] -> w762
                    frame "Getting next assignment", Default {
                      n707 = local read "Temperature Control Error - Reactor 8"() -> (w764:errorcluster)
                      n708 = script code="% Get the index for the next reaction along with its start time, temperature, and residence time\nif ~isempty(reactor_8_rxns)\n     reactor_8_done = 0;\n     reactor_8_reaction = reactor_8_rxns(1);\n     reactor_8_start_time = reactors_start_times(8, reactor_8_reaction);\n     reactor_8_temperature_C = all_slugs(reactor_8_reaction).temperature;\n     reactor_8_res_time = all_slugs(reactor_8_reaction).residence_time_goal;\n     % convert temperature to degF and string for Watlow\n     reactor_8_temperature_F = num2str((reactor_8_temperature_C * 1.8) + 32);\nelse\n     reactor_8_done = 1;\nend"("??"=w764) -> ("??"=w768:errorcluster, "reactor_8_start_time"=→"r8_start_time":dbl, "reactor_8_temperature_F"=→"r8_temp_F":string, "reactor_8_res_time"=→"r8_res_time":dbl, "reactor_8_done"=w767:dbl)
                      n709 = Greater?(x=w767, y=0.0) -> (0:w765:bool)
                      n710 = case shown="True" w765 {
                        tunnel: [Reactors_Enum_NSE."Running" ("Enum") Reactors_Enum_NSE."Done" ("Enum")] -> w769
                        tunnel: w768 -> [w774 w784]
                        tunnel: [w773 w781] -> w763
                        frame False {
                          w776 = u16 7001 items=["Read temperature (F)"=4001, "Read setpoint (F)"=8029, "Write setpoint (F)"=7001, "Read autotune status"=8027, "Write start autotune"=8026]
                          n711 = local read "Watlow COM"() -> (w777:refnum<visa-resource-name>)
                          n712 = local read "Watlow Zone - Reactor 8"() -> (w778:dbl)
                          n713 = local read "Watlow Instance - Reactor 8"() -> (w779:dbl)
                          n714 = local read "r8_temp_F"() -> (w775:string)
                          n715 = call "Write.vi"("PC Comms Port"=w777, "Zone"=w778, "Parameter"=w776, "Instance"=w779, "Write Value"=w775, "Error In"=w774) -> ("Error Out"=w773:errorcluster)  [unwired: 13 in]
                        }
                        frame True {
                          w785 = u16 7001 items=["Read temperature (F)"=4001, "Read setpoint (F)"=8029, "Write setpoint (F)"=7001, "Read autotune status"=8027, "Write start autotune"=8026]
                          # "Reactor is done for now.\nWrite a low set point to cool it down"
                          n716 = local read "Watlow COM"() -> (w786:refnum<visa-resource-name>)
                          n717 = local read "Watlow Zone - Reactor 8"() -> (w787:dbl)
                          n718 = local read "Watlow Instance - Reactor 8"() -> (w788:dbl)
                          n719 = local write "r8_done"(TRUE) -> ()
                          n720 = call "Write.vi"("PC Comms Port"=w786, "Zone"=w787, "Parameter"=w785, "Instance"=w788, "Write Value"="50", "Error In"=w784) -> ("Error Out"=w781:errorcluster)  [unwired: 13 in]
                        }
                      }
                      n721 = local write "Temperature Control Error - Reactor 8"(w763) -> ()
                    }
                    frame "Running" {
                      n722 = while {
                        stop <- w791 stop-if-true
                        # "Once the master time exceeds\nthe current start time plus the\ncurrent residence time, stop\nand go back to get the next\nassignment"
                        n723 = local read "r8_start_time"() -> (w796:dbl)
                        n724 = local read "r8_res_time"() -> (w795:dbl)
                        n725 = local read "Master time [s]"() -> (w793:dbl)
                        n726 = Add(x=w796, y=w795) -> (x+y=w794:dbl)
                        n727 = Greater?(x=w793, y=w794) -> (0:w792:bool)
                        n728 = case shown="True" w792 {
                          selector: w792 -> [w797 w800]
                          tunnel: [w797 w800] -> w791
                          frame False {
                            n729 = Wait (ms)(milliseconds to wait=500) -> ()  [unwired: 1 out]
                          }
                          frame True {
                            n730 = script code="reactor_8_rxns(1) = []; % remove the reaction index that just ran"("??"=errorcluster {"status"=FALSE, "code"=0, "source"=""} ("error constant")) -> ()  [unwired: 1 out]
                          }
                        }
                      }
                    }
                    frame "Done" {
                    }
                  }
                  n731 = Wait (ms)(milliseconds to wait=1000) -> ()  [unwired: 1 out]
                  n732 = local read "r8_done"() -> (w760:bool)
                }
              }
            }
            n733 = case shown="True" w710 {
              frame False {
              }
              frame True {
                # "Reactor 9"
                n734 = while {
                  shift-right: [w718] -> _
                  shift-left: Reactors_Enum_NSE."Getting next assignment" ("Enum") -> [w717]
                  stop <- w716 stop-if-true
                  n735 = case shown="\"Getting next assignment\", Default" w717 {
                    tunnel: [w725 Reactors_Enum_NSE."Getting next assignment" ("Enum") Reactors_Enum_NSE."Done" ("Enum")] -> w718
                    frame "Getting next assignment", Default {
                      n736 = local read "Temperature Control Error - Reactor 9"() -> (w720:errorcluster)
                      n737 = script code="% Get the index for the next reaction along with its start time, temperature, and residence time\nif ~isempty(reactor_9_rxns)\n     reactor_9_done = 0;\n     reactor_9_reaction = reactor_9_rxns(1);\n     reactor_9_start_time = reactors_start_times(9, reactor_9_reaction);\n     reactor_9_temperature_C = all_slugs(reactor_9_reaction).temperature;\n     reactor_9_res_time = all_slugs(reactor_9_reaction).residence_time_goal;\n     % convert temperature to degF and string for Watlow\n     reactor_9_temperature_F = num2str((reactor_9_temperature_C * 1.8) + 32);\nelse\n     reactor_9_done = 1;\nend"("??"=w720) -> ("??"=w724:errorcluster, "reactor_9_start_time"=→"r9_start_time":dbl, "reactor_9_temperature_F"=→"r9_temp_F":string, "reactor_9_res_time"=→"r9_res_time":dbl, "reactor_9_done"=w723:dbl)
                      n738 = Greater?(x=w723, y=0.0) -> (0:w721:bool)
                      n739 = case shown="True" w721 {
                        tunnel: [Reactors_Enum_NSE."Running" ("Enum") Reactors_Enum_NSE."Done" ("Enum")] -> w725
                        tunnel: w724 -> [w730 w740]
                        tunnel: [w729 w737] -> w719
                        frame False {
                          w732 = u16 7001 items=["Read temperature (F)"=4001, "Read setpoint (F)"=8029, "Write setpoint (F)"=7001, "Read autotune status"=8027, "Write start autotune"=8026]
                          n740 = local read "Watlow COM"() -> (w733:refnum<visa-resource-name>)
                          n741 = local read "Watlow Zone - Reactor 9"() -> (w734:dbl)
                          n742 = local read "Watlow Instance - Reactor 9"() -> (w735:dbl)
                          n743 = local read "r9_temp_F"() -> (w731:string)
                          n744 = call "Write.vi"("PC Comms Port"=w733, "Zone"=w734, "Parameter"=w732, "Instance"=w735, "Write Value"=w731, "Error In"=w730) -> ("Error Out"=w729:errorcluster)  [unwired: 13 in]
                        }
                        frame True {
                          w741 = u16 7001 items=["Read temperature (F)"=4001, "Read setpoint (F)"=8029, "Write setpoint (F)"=7001, "Read autotune status"=8027, "Write start autotune"=8026]
                          # "Reactor is done for now.\nWrite a low set point to cool it down"
                          n745 = local read "Watlow COM"() -> (w742:refnum<visa-resource-name>)
                          n746 = local read "Watlow Zone - Reactor 9"() -> (w743:dbl)
                          n747 = local read "Watlow Instance - Reactor 9"() -> (w744:dbl)
                          n748 = local write "r9_done"(TRUE) -> ()
                          n749 = call "Write.vi"("PC Comms Port"=w742, "Zone"=w743, "Parameter"=w741, "Instance"=w744, "Write Value"="50", "Error In"=w740) -> ("Error Out"=w737:errorcluster)  [unwired: 13 in]
                        }
                      }
                      n750 = local write "Temperature Control Error - Reactor 9"(w719) -> ()
                    }
                    frame "Running" {
                      n751 = while {
                        stop <- w747 stop-if-true
                        # "Once the master time exceeds\nthe current start time plus the\ncurrent residence time, stop\nand go back to get the next\nassignment"
                        n752 = local read "r9_start_time"() -> (w752:dbl)
                        n753 = local read "r9_res_time"() -> (w751:dbl)
                        n754 = local read "Master time [s]"() -> (w749:dbl)
                        n755 = Add(x=w752, y=w751) -> (x+y=w750:dbl)
                        n756 = Greater?(x=w749, y=w750) -> (0:w748:bool)
                        n757 = case shown="False" w748 {
                          selector: w748 -> [w753 w756]
                          tunnel: [w753 w756] -> w747
                          frame False {
                            n758 = Wait (ms)(milliseconds to wait=500) -> ()  [unwired: 1 out]
                          }
                          frame True {
                            n759 = script code="reactor_9_rxns(1) = []; % remove the reaction index that just ran"("??"=errorcluster {"status"=FALSE, "code"=0, "source"=""} ("error constant")) -> ()  [unwired: 1 out]
                          }
                        }
                      }
                    }
                    frame "Done" {
                    }
                  }
                  n760 = Wait (ms)(milliseconds to wait=1000) -> ()  [unwired: 1 out]
                  n761 = local read "r9_done"() -> (w716:bool)
                }
              }
            }
            n762 = case shown="True" w711 {
              frame False {
              }
              frame True {
                # "Reactor 10"
                n763 = while {
                  shift-right: [w1114] -> _
                  shift-left: Reactors_Enum_NSE."Getting next assignment" ("Enum") -> [w1113]
                  stop <- w1112 stop-if-true
                  n764 = case shown="\"Getting next assignment\", Default" w1113 {
                    tunnel: [w1121 Reactors_Enum_NSE."Getting next assignment" ("Enum") Reactors_Enum_NSE."Done" ("Enum")] -> w1114
                    frame "Getting next assignment", Default {
                      n765 = local read "Temperature Control Error - Reactor 9"() -> (w1116:errorcluster)
                      n766 = script code="% Get the index for the next reaction along with its start time, temperature, and residence time\nif ~isempty(reactor_10_rxns)\n     reactor_10_done = 0;\n     reactor_10_reaction = reactor_10_rxns(1);\n     reactor_10_start_time = reactors_start_times(10, reactor_10_reaction);\n     reactor_10_temperature_C = all_slugs(reactor_10_reaction).temperature;\n     reactor_10_res_time = all_slugs(reactor_10_reaction).residence_time_goal;\n     % convert temperature to degF and string for Watlow\n     reactor_10_temperature_F = num2str((reactor_10_temperature_C * 1.8) + 32);\nelse\n     reactor_10_done = 1;\nend"("??"=w1116) -> ("??"=w1120:errorcluster, "reactor_10_start_time"=→"r10_start_time":dbl, "reactor_10_temperature_F"=→"r10_temp_F":string, "reactor_10_res_time"=→"r10_res_time":dbl, "reactor_10_done"=w1119:dbl)
                      n767 = Greater?(x=w1119, y=0.0) -> (0:w1117:bool)
                      n768 = case shown="True" w1117 {
                        tunnel: [Reactors_Enum_NSE."Running" ("Enum") Reactors_Enum_NSE."Done" ("Enum")] -> w1121
                        tunnel: w1120 -> [w1126 w1136]
                        tunnel: [w1125 w1133] -> w1115
                        frame False {
                          w1128 = u16 7001 items=["Read temperature (F)"=4001, "Read setpoint (F)"=8029, "Write setpoint (F)"=7001, "Read autotune status"=8027, "Write start autotune"=8026]
                          n769 = local read "Watlow Zone - Reactor 10"() -> (w1130:dbl)
                          n770 = local read "Watlow Instance - Reactor 10"() -> (w1131:dbl)
                          n771 = local read "r10_temp_F"() -> (w1127:string)
                          n772 = local read "Watlow COM"() -> (w1129:refnum<visa-resource-name>)
                          n773 = call "Write.vi"("PC Comms Port"=w1129, "Zone"=w1130, "Parameter"=w1128, "Instance"=w1131, "Write Value"=w1127, "Error In"=w1126) -> ("Error Out"=w1125:errorcluster)  [unwired: 13 in]
                        }
                        frame True {
                          w1137 = u16 7001 items=["Read temperature (F)"=4001, "Read setpoint (F)"=8029, "Write setpoint (F)"=7001, "Read autotune status"=8027, "Write start autotune"=8026]
                          # "Reactor is done for now.\nWrite a low set point to cool it down"
                          n774 = local read "Watlow Zone - Reactor 10"() -> (w1139:dbl)
                          n775 = local read "Watlow Instance - Reactor 10"() -> (w1140:dbl)
                          n776 = local read "Watlow COM"() -> (w1138:refnum<visa-resource-name>)
                          n777 = local write "r10_done"(TRUE) -> ()
                          n778 = call "Write.vi"("PC Comms Port"=w1138, "Zone"=w1139, "Parameter"=w1137, "Instance"=w1140, "Write Value"="50", "Error In"=w1136) -> ("Error Out"=w1133:errorcluster)  [unwired: 13 in]
                        }
                      }
                      n779 = local write "Temperature Control Error - Reactor 9"(w1115) -> ()
                    }
                    frame "Running" {
                      n780 = while {
                        stop <- w1143 stop-if-true
                        # "Once the master time exceeds\nthe current start time plus the\ncurrent residence time, stop\nand go back to get the next\nassignment"
                        n781 = local read "r10_start_time"() -> (w1148:dbl)
                        n782 = local read "r10_res_time"() -> (w1147:dbl)
                        n783 = local read "Master time [s]"() -> (w1145:dbl)
                        n784 = Add(x=w1148, y=w1147) -> (x+y=w1146:dbl)
                        n785 = Greater?(x=w1145, y=w1146) -> (0:w1144:bool)
                        n786 = case shown="True" w1144 {
                          selector: w1144 -> [w1149 w1152]
                          tunnel: [w1149 w1152] -> w1143
                          frame False {
                            n787 = Wait (ms)(milliseconds to wait=500) -> ()  [unwired: 1 out]
                          }
                          frame True {
                            n788 = script code="reactor_10_rxns(1) = []; % remove the reaction index that just ran"("??"=errorcluster {"status"=FALSE, "code"=0, "source"=""} ("error constant")) -> ()  [unwired: 1 out]
                          }
                        }
                      }
                    }
                    frame "Done" {
                    }
                  }
                  n789 = Wait (ms)(milliseconds to wait=1000) -> ()  [unwired: 1 out]
                  n790 = local read "r10_done"() -> (w1112:bool)
                }
              }
            }
            n791 = while {
              tunnel: [errorcluster {"status"=FALSE, "code"=0, "source"=""} ("error constant")] -> w701
              stop <- w1155 stop-if-true
              w1179 = u16 4001 items=["Read temperature (F)"=4001, "Read setpoint (F)"=8029, "Write setpoint (F)"=7001, "Read autotune status"=8027, "Write start autotune"=8026]
              # "update displayed\ntemperature values\nevery five seconds"
              n792 = local read "Watlow COM"() -> (w1180:refnum<visa-resource-name>)
              n793 = local read "Temperature Control Error - Reactor 1"() -> (w1178:errorcluster)
              n794 = local read "Temperature Control Error - Reactor 2"() -> (w1177:errorcluster)
              n795 = local read "Temperature Control Error - Reactor 3"() -> (w1176:errorcluster)
              n796 = local read "Temperature Control Error - Reactor 4"() -> (w1175:errorcluster)
              n797 = local read "Temperature Control Error - Reactor 5"() -> (w1174:errorcluster)
              n798 = local read "Temperature Control Error - Reactor 6"() -> (w1173:errorcluster)
              n799 = local read "Temperature Control Error - Reactor 7"() -> (w1172:errorcluster)
              n800 = local read "Temperature Control Error - Reactor 8"() -> (w1171:errorcluster)
              n801 = local read "Temperature Control Error - Reactor 9"() -> (w1170:errorcluster)
              n802 = local read "Temperature Control Error - Reactor 10"() -> (w1169:errorcluster)
              n803 = Wait (ms)(milliseconds to wait=5000) -> ()  [unwired: 1 out]
              n804 = local read "Reactor 5 enabled?"() -> (w1163:bool)
              n805 = local read "Reactor 4 enabled?"() -> (w1164:bool)
              n806 = local read "Reactor 3 enabled?"() -> (w1165:bool)
              n807 = local read "Reactor 10 enabled?"() -> (w1158:bool)
              n808 = local read "Reactor 1 enabled?"() -> (w1167:bool)
              n809 = local read "Reactor 6 enabled?"() -> (w1162:bool)
              n810 = local read "Reactor 7 enabled?"() -> (w1161:bool)
              n811 = local read "Reactor 8 enabled?"() -> (w1160:bool)
              n812 = local read "Reactor 9 enabled?"() -> (w1159:bool)
              n813 = local read "Reactor 2 enabled?"() -> (w1166:bool)
              n814 = case shown="True" w1167 {
                tunnel: w1180 -> [_ w1196]
                tunnel: w1179 -> [_ w1195]
                tunnel: w1178 -> [_ w1191]
                frame False {
                }
                frame True {
                  n815 = local read "Watlow Instance - Reactor 1"() -> (w1197:dbl)
                  n816 = local read "Watlow Zone - Reactor 1"() -> (w1198:dbl)
                  n817 = call "Read.vi"("PC Comms Port"=w1196, "Zone"=w1198, "Parameter"=w1195, "Instance"=w1197, "Error In"=w1191) -> ("Read Value"=w1193:string, "Error Out"=w1192:errorcluster)  [unwired: 13 in]
                  n818 = script code="r1_temp_degC = (str2num(r1_temp_degF) - 32) / 1.8;"("??"=w1192, "r1_temp_degF"=w1193) -> ("??"=w1190:errorcluster, "r1_temp_degC"=w1194:dbl)
                  n819 = local write "Temperature - Reactor 1"(w1194) -> ()
                  n820 = local write "Temperature Control Error - Reactor 1"(w1190) -> ()
                }
              }
              n821 = case shown="True" w1158 {
                tunnel: w1180 -> [_ w1268]
                tunnel: w1179 -> [_ w1267]
                tunnel: w1169 -> [_ w1263]
                frame False {
                }
                frame True {
                  n822 = local read "Watlow Instance - Reactor 10"() -> (w1269:dbl)
                  n823 = local read "Watlow Zone - Reactor 10"() -> (w1270:dbl)
                  n824 = call "Read.vi"("PC Comms Port"=w1268, "Zone"=w1270, "Parameter"=w1267, "Instance"=w1269, "Error In"=w1263) -> ("Read Value"=w1265:string, "Error Out"=w1264:errorcluster)  [unwired: 13 in]
                  n825 = script code="r10_temp_degC = (str2num(r10_temp_degF) - 32) / 1.8;"("??"=w1264, "r10_temp_degF"=w1265) -> ("??"=w1262:errorcluster, "r10_temp_degC"=w1266:dbl)
                  n826 = local write "Temperature - Reactor 10"(w1266) -> ()
                  n827 = local write "Temperature Control Error - Reactor 10"(w1262) -> ()
                }
              }
              n828 = case shown="True" w1159 {
                tunnel: w1180 -> [_ w1259]
                tunnel: w1179 -> [_ w1258]
                tunnel: w1170 -> [_ w1254]
                frame False {
                }
                frame True {
                  n829 = local read "Watlow Instance - Reactor 9"() -> (w1260:dbl)
                  n830 = local read "Watlow Zone - Reactor 9"() -> (w1261:dbl)
                  n831 = call "Read.vi"("PC Comms Port"=w1259, "Zone"=w1261, "Parameter"=w1258, "Instance"=w1260, "Error In"=w1254) -> ("Read Value"=w1256:string, "Error Out"=w1255:errorcluster)  [unwired: 13 in]
                  n832 = script code="r9_temp_degC = (str2num(r9_temp_degF) - 32) / 1.8;"("??"=w1255, "r9_temp_degF"=w1256) -> ("??"=w1253:errorcluster, "r9_temp_degC"=w1257:dbl)
                  n833 = local write "Temperature - Reactor 9"(w1257) -> ()
                  n834 = local write "Temperature Control Error - Reactor 9"(w1253) -> ()
                }
              }
              n835 = case shown="True" w1160 {
                tunnel: w1180 -> [_ w1250]
                tunnel: w1179 -> [_ w1249]
                tunnel: w1171 -> [_ w1245]
                frame False {
                }
                frame True {
                  n836 = local read "Watlow Instance - Reactor 8"() -> (w1251:dbl)
                  n837 = local read "Watlow Zone - Reactor 8"() -> (w1252:dbl)
                  n838 = call "Read.vi"("PC Comms Port"=w1250, "Zone"=w1252, "Parameter"=w1249, "Instance"=w1251, "Error In"=w1245) -> ("Read Value"=w1247:string, "Error Out"=w1246:errorcluster)  [unwired: 13 in]
                  n839 = script code="r8_temp_degC = (str2num(r8_temp_degF) - 32) / 1.8;"("??"=w1246, "r8_temp_degF"=w1247) -> ("??"=w1244:errorcluster, "r8_temp_degC"=w1248:dbl)
                  n840 = local write "Temperature - Reactor 8"(w1248) -> ()
                  n841 = local write "Temperature Control Error - Reactor 8"(w1244) -> ()
                }
              }
              n842 = case shown="True" w1161 {
                tunnel: w1180 -> [_ w1241]
                tunnel: w1179 -> [_ w1240]
                tunnel: w1172 -> [_ w1236]
                frame False {
                }
                frame True {
                  n843 = local read "Watlow Instance - Reactor 7"() -> (w1242:dbl)
                  n844 = local read "Watlow Zone - Reactor 7"() -> (w1243:dbl)
                  n845 = call "Read.vi"("PC Comms Port"=w1241, "Zone"=w1243, "Parameter"=w1240, "Instance"=w1242, "Error In"=w1236) -> ("Read Value"=w1238:string, "Error Out"=w1237:errorcluster)  [unwired: 13 in]
                  n846 = script code="r7_temp_degC = (str2num(r7_temp_degF) - 32) / 1.8;"("??"=w1237, "r7_temp_degF"=w1238) -> ("??"=w1235:errorcluster, "r7_temp_degC"=w1239:dbl)
                  n847 = local write "Temperature - Reactor 7"(w1239) -> ()
                  n848 = local write "Temperature Control Error - Reactor 7"(w1235) -> ()
                }
              }
              n849 = case shown="True" w1162 {
                tunnel: w1180 -> [_ w1232]
                tunnel: w1179 -> [_ w1231]
                tunnel: w1173 -> [_ w1227]
                frame False {
                }
                frame True {
                  n850 = local read "Watlow Instance - Reactor 6"() -> (w1233:dbl)
                  n851 = local read "Watlow Zone - Reactor 6"() -> (w1234:dbl)
                  n852 = call "Read.vi"("PC Comms Port"=w1232, "Zone"=w1234, "Parameter"=w1231, "Instance"=w1233, "Error In"=w1227) -> ("Read Value"=w1229:string, "Error Out"=w1228:errorcluster)  [unwired: 13 in]
                  n853 = script code="r6_temp_degC = (str2num(r6_temp_degF) - 32) / 1.8;"("??"=w1228, "r6_temp_degF"=w1229) -> ("??"=w1226:errorcluster, "r6_temp_degC"=w1230:dbl)
                  n854 = local write "Temperature - Reactor 6"(w1230) -> ()
                  n855 = local write "Temperature Control Error - Reactor 6"(w1226) -> ()
                }
              }
              n856 = case shown="True" w1163 {
                tunnel: w1180 -> [_ w1223]
                tunnel: w1179 -> [_ w1222]
                tunnel: w1174 -> [_ w1218]
                frame False {
                }
                frame True {
                  n857 = local read "Watlow Instance - Reactor 5"() -> (w1224:dbl)
                  n858 = local read "Watlow Zone - Reactor 5"() -> (w1225:dbl)
                  n859 = call "Read.vi"("PC Comms Port"=w1223, "Zone"=w1225, "Parameter"=w1222, "Instance"=w1224, "Error In"=w1218) -> ("Read Value"=w1220:string, "Error Out"=w1219:errorcluster)  [unwired: 13 in]
                  n860 = script code="r5_temp_degC = (str2num(r5_temp_degF) - 32) / 1.8;"("??"=w1219, "r5_temp_degF"=w1220) -> ("??"=w1217:errorcluster, "r5_temp_degC"=w1221:dbl)
                  n861 = local write "Temperature - Reactor 5"(w1221) -> ()
                  n862 = local write "Temperature Control Error - Reactor 5"(w1217) -> ()
                }
              }
              n863 = case shown="True" w1164 {
                tunnel: w1180 -> [_ w1214]
                tunnel: w1179 -> [_ w1213]
                tunnel: w1175 -> [_ w1209]
                frame False {
                }
                frame True {
                  n864 = local read "Watlow Instance - Reactor 4"() -> (w1215:dbl)
                  n865 = local read "Watlow Zone - Reactor 4"() -> (w1216:dbl)
                  n866 = call "Read.vi"("PC Comms Port"=w1214, "Zone"=w1216, "Parameter"=w1213, "Instance"=w1215, "Error In"=w1209) -> ("Read Value"=w1211:string, "Error Out"=w1210:errorcluster)  [unwired: 13 in]
                  n867 = script code="r4_temp_degC = (str2num(r4_temp_degF) - 32) / 1.8;"("??"=w1210, "r4_temp_degF"=w1211) -> ("??"=w1208:errorcluster, "r4_temp_degC"=w1212:dbl)
                  n868 = local write "Temperature - Reactor 4"(w1212) -> ()
                  n869 = local write "Temperature Control Error - Reactor 4"(w1208) -> ()
                }
              }
              n870 = case shown="True" w1165 {
                tunnel: w1180 -> [_ w1205]
                tunnel: w1179 -> [_ w1204]
                tunnel: w1176 -> [_ w1200]
                frame False {
                }
                frame True {
                  n871 = local read "Watlow Instance - Reactor 3"() -> (w1206:dbl)
                  n872 = local read "Watlow Zone - Reactor 3"() -> (w1207:dbl)
                  n873 = call "Read.vi"("PC Comms Port"=w1205, "Zone"=w1207, "Parameter"=w1204, "Instance"=w1206, "Error In"=w1200) -> ("Read Value"=w1202:string, "Error Out"=w1201:errorcluster)  [unwired: 13 in]
                  n874 = script code="r3_temp_degC = (str2num(r3_temp_degF) - 32) / 1.8;"("??"=w1201, "r3_temp_degF"=w1202) -> ("??"=w1199:errorcluster, "r3_temp_degC"=w1203:dbl)
                  n875 = local write "Temperature - Reactor 3"(w1203) -> ()
                  n876 = local write "Temperature Control Error - Reactor 3"(w1199) -> ()
                }
              }
              n877 = case shown="True" w1166 {
                tunnel: w1180 -> [_ w1187]
                tunnel: w1179 -> [_ w1186]
                tunnel: w1177 -> [_ w1182]
                frame False {
                }
                frame True {
                  n878 = local read "Watlow Instance - Reactor 2"() -> (w1188:dbl)
                  n879 = local read "Watlow Zone - Reactor 2"() -> (w1189:dbl)
                  n880 = call "Read.vi"("PC Comms Port"=w1187, "Zone"=w1189, "Parameter"=w1186, "Instance"=w1188, "Error In"=w1182) -> ("Read Value"=w1184:string, "Error Out"=w1183:errorcluster)  [unwired: 13 in]
                  n881 = script code="r2_temp_degC = (str2num(r2_temp_degF) - 32) / 1.8;"("??"=w1183, "r2_temp_degF"=w1184) -> ("??"=w1181:errorcluster, "r2_temp_degC"=w1185:dbl)
                  n882 = local write "Temperature - Reactor 2"(w1185) -> ()
                  n883 = local write "Temperature Control Error - Reactor 2"(w1181) -> ()
                }
              }
              n884 = local read "Stop everything"() -> (w1156:bool)
              n885 = local read "schedule_reset"() -> (w1157:bool)
              n886 = Or(x=w1157, y=w1156) -> (x .or. y?=w1155:bool)
            }
            n887 = local read "schedule_reset"() -> (w700:bool)
            n888 = case shown="False" w700 {
              tunnel: w701 -> [_ _]
              tunnel: [Reactor_Outer_Loop_Enum_NSE."Running" ("Enum") Reactor_Outer_Loop_Enum_NSE."Waiting for hardware initialization" ("Enum")] -> w699
              frame False {
              }
              frame True {
              }
            }
          }
        }
        n889 = local read "Stop everything"() -> (w646:bool)
      }
    }
  }
  n890 = while {
    stop <- w1272 stop-if-true
    n891 = local read "Ready to start schedule timer"() -> (w1273:bool)
    n892 = local read "Stop everything"() -> (w1272:bool)
    n893 = Wait (ms)(milliseconds to wait=500) -> ()  [unwired: 1 out]
    n894 = case shown="True" w1273 {
      frame False {
      }
      frame True {
        n895 = Get Date/Time In Seconds() -> (seconds since 1Jan1904=w1275:timestamp)
        n896 = To Double Precision Float(number=w1275) -> (double precision float=w1274:dbl)
        n897 = while {
          stop <- w1296 stop-if-true
          # "Same signal temporarily wired\nto R10 and analytical valve readings\ndue to hardware problem on MIT side"
          # "Express --> Sig Manip --> Split Signals"
          n898 = local read "Analog Input (NI 9205) task out"() -> (w1294:refnum<k21>)
          n899 = local read "Analog Input DAQ Error"() -> (w1292:errorcluster)
          n900 = call-poly <vilib>:"DAQmx Read.vi"("task/channels in"=w1294, "timeout"=1.0, "error in"=w1292) -> ("data"=w1291:waveform(dbl)[], "error out"=w1278:errorcluster)  [unwired: 10 in, 1 out]
          "Analog input 3" <- w1291
          n901 = local write "Analog Input DAQ Error"(w1278) -> ()
          n902 = case shown="Error .." w1278 {
            tunnel: w1294 -> [_ w1300]
            frame No Error {
            }
            frame Error {
              n903 = call "STOP_CDAQ_NIMAX_NSE_Parallel_AnalogInputOnly.vi"("Analog input DAQmx Task"=w1300, "Error In"=errorcluster {"status"=FALSE, "code"=0, "source"=""} ("error constant")) -> ("error out"=w1299:errorcluster)  [unwired: 13 in]
              n904 = call "START_CDAQ_NIMAX_NSE_Parallel.vi"("error in (no error)"=w1299) -> ("analog input (NI 9205) task out"=w1302:refnum<k21>, "analog input (NI 9205) error out"=w1298:errorcluster)  [unwired: 21 in, 4 out]
              n905 = local write "Analog Input (NI 9205) task out"(w1302) -> ()
              n906 = local write "Analog Input DAQ Error"(w1298) -> ()
              n907 = Unbundle By Name(w1298) -> ("status"=w1297:bool)
              n908 = local write "Analog input DAQ error"(w1297) -> ()
            }
          }
          n909 = Unbundle By Name(w1278) -> ("status"=w1279:bool)
          n910 = Wait (ms)(milliseconds to wait=100) -> ()  [unwired: 1 out]
          n911 = local write "Analog input DAQ error"(w1279) -> ()
          n912 = call "Select Signals"("Signals"=w1291) -> ("Signal Out"=w1290:dynamicdata)  [unwired: 9 in, 1 out]
          n913 = Split Signals(w1290) -> (w1289:dynamicdata, w1288:dynamicdata, w1287:dynamicdata, w1286:dynamicdata, w1285:dynamicdata, w1284:dynamicdata, w1283:dynamicdata, w1282:dynamicdata, w1281:dynamicdata, w1277:dynamicdata, w1280:dynamicdata, w1276:dynamicdata)  [unwired: 13 in, 1 out]
          n914 = local write "Phase Sensor Reading - Reactor 10"(w1276) -> ()
          n915 = local write "Phase Sensor Reading - Reactor 1"(w1289) -> ()
          n916 = local write "Phase Sensor Reading - Reactor 2"(w1288) -> ()
          n917 = local write "Phase Sensor Reading - Reactor 3"(w1287) -> ()
          n918 = local write "Phase Sensor Reading - Reactor 4"(w1286) -> ()
          n919 = local write "Phase Sensor Reading - Reactor 5"(w1285) -> ()
          n920 = local write "Phase Sensor Reading - Reactor 6"(w1284) -> ()
          n921 = local write "Phase Sensor Reading - Reactor 7"(w1283) -> ()
          n922 = local write "Phase Sensor Reading - Reactor 8"(w1282) -> ()
          n923 = local write "Phase Sensor Reading - Reactor 9"(w1281) -> ()
          n924 = local write "Phase Sensor Reading - Analytical Valve"(w1277) -> ()
          n925 = local write "Phase Sensor Reading - Injection Valve [V]"(w1280) -> ()
          n926 = local read "Stop everything"() -> (w1296:bool)
        }
        n927 = while {
          tunnel: w1274 -> [w1305]
          stop <- w1304 stop-if-true
          n928 = Get Date/Time In Seconds() -> (seconds since 1Jan1904=w1308:timestamp)
          n929 = To Double Precision Float(number=w1308) -> (double precision float=w1307:dbl)
          n930 = Subtract(x=w1307, y=w1305) -> (x-y=w1306:dbl)
          n931 = local write "Master time [s]"(w1306) -> ()
          n932 = Wait (ms)(milliseconds to wait=1000) -> ()  [unwired: 1 out]
          n933 = local read "Stop everything"() -> (w1304:bool)
        }
      }
    }
  }
  n934 = while {
    shift-right: [w1313] -> _
    shift-left: Rinse_Vent_Reactor_Enum_NSE."Waiting for hardware initialization" ("Enum") -> [w1312]
    shift-right: [w1310] -> _
    shift-left: Rinse_Vent_Transfer_Lines_Enum_NSE_-_Copy."Waiting for hardware initialization" ("Enum") -> [w1311]
    stop <- w1309 stop-if-true
    # "Rinse and Vent Sequence - Reactor Included"
    # "Rinse and Vent Sequence - Transfer Lines Only"
    n935 = while {
      shift-right: [w1438] -> w1310
      shift-left: w1311 -> [w1439]
      stop <- w1437 stop-if-true
      n936 = case shown="\"Rinse and vent transfer lines in progress\"" w1439 {
        tunnel: [w1440 w1451 Rinse_Vent_Transfer_Lines_Enum_NSE_-_Copy."Rinse and vent transfer lines sequence is idle" ("Enum")] -> w1438
        frame "Waiting for hardware initialization", Default {
          n937 = local read "Ready to start schedule timer"() -> (w1441:bool)
          n938 = case shown="True" w1441 {
            tunnel: [Rinse_Vent_Transfer_Lines_Enum_NSE_-_Copy."Waiting for hardware initialization" ("Enum") Rinse_Vent_Transfer_Lines_Enum_NSE_-_Copy."Rinse and vent transfer lines sequence is idle" ("Enum")] -> w1440
            frame False {
              n939 = Wait (ms)(milliseconds to wait=500) -> ()  [unwired: 1 out]
            }
            frame True {
            }
          }
        }
        frame "Rinse and vent transfer lines sequence is idle" {
          n940 = local read "Reaction number - rinse transfer lines"() -> (w1445:dbl)
          n941 = local read "Schedule - Rinse Transfer Lines"() -> (w1448:dbl[])
          n942 = script code="rinse_transfer_lines_finished = 0;\nrinse_transfer_lines_next_rxn = rinse_transfer_lines_last_rxn + 1;\nif rinse_transfer_lines_next_rxn <= numel(rinse_transfer_lines_start_times)\n    rinse_transfer_lines_next_start_time = rinse_transfer_lines_start_times(rinse_transfer_lines_next_rxn);\nelse\n    rinse_transfer_lines_finished = 1;\nend"("??"=errorcluster {"status"=FALSE, "code"=0, "source"=""} ("error constant"), "rinse_transfer_lines_start_times"=w1448, "rinse_transfer_lines_last_rxn"=w1445) -> ("??"=w1450:errorcluster, "rinse_transfer_lines_next_start_time"=w1452:dbl, "rinse_transfer_lines_finished"=w1447:dbl)
          n943 = local write "Next start time - rinse transfer lines"(w1452) -> ()
          n944 = while {
            tunnel: [w1464] -> w1451
            tunnel: w1450 -> [w1462]
            stop <- w1453 stop-if-true
            n945 = local read "rinse_transfer_lines_finished"() -> (w1456:bool)
            n946 = local read "Next start time - rinse transfer lines"() -> (w1466:dbl)
            n947 = local read "Master time [s]"() -> (w1465:dbl)
            n948 = Less Or Equal?(x=w1466, y=w1465) -> (x <= y?=w1459:bool)
            n949 = call "Time Delay36"("error in (no error)"=w1462, "Delay Time (s)"=0.5) -> ("error out"=w1460:errorcluster)  [unwired: 9 in]
            n950 = Not(x=w1456) -> (.not. x?=w1457:bool)
            n951 = And(x=w1459, y=w1457) -> (x .and. y?=w1458:bool)
            n952 = case shown="False" w1458 {
              selector: w1458 -> [w1467 w1472]
              tunnel: [Rinse_Vent_Transfer_Lines_Enum_NSE_-_Copy."Rinse and vent transfer lines sequence is idle" ("Enum") Rinse_Vent_Transfer_Lines_Enum_NSE_-_Copy."Rinse and vent transfer lines in progress" ("Enum")] -> w1464
              tunnel: [w1467 w1472] -> w1455
              tunnel: w1460 -> [_ w1471]
              frame False {
                n953 = Wait (ms)(milliseconds to wait=500) -> ()  [unwired: 1 out]
              }
              frame True {
                n954 = call "Time Delay13"("error in (no error)"=w1471, "Delay Time (s)"=0.5) -> ()  [unwired: 9 in, 1 out]
              }
            }
            n955 = Wait (ms)(milliseconds to wait=1000) -> ()  [unwired: 1 out]
            n956 = local read "schedule_reset"() -> (w1454:bool)
            n957 = Or(x=w1455, y=w1454) -> (x .or. y?=w1453:bool)
          }
          n958 = Not Equal To 0?(x=w1447) -> (x != 0?=w1446:bool)
          n959 = local write "rinse_transfer_lines_finished"(w1446) -> ()
        }
        frame "Rinse and vent transfer lines in progress" {
          n960 = local read "Carrier Syringe Infuse\nRate (Rinse) (uL/min)"() -> (w1519:dbl)
          n961 = local read "Carrier Pump COM"() -> (w1521:refnum<visa-resource-name>)
          n962 = local read "Carrier Pump ID"() -> (w1520:i32)
          n963 = local read "Number of rinse droplets"() -> (w1550:i32)
          n964 = call "HARVARD_SETFLOWRATE_INFUSE.vi"("VISA resource name"=w1521, "Pump address (0)"=w1520, "Infuse Flow Rate (80)"=w1519, "error in (no error)"=errorcluster {"status"=FALSE, "code"=0, "source"=""} ("error constant")) -> ("error out"=w1522:errorcluster)  [unwired: 9 in, 2 out]
          n965 = for {
            N: w1550 -> [_]
            shift-right: [w1561] -> w1491
            shift-left: w1522 -> [w1552]
            n966 = local read "Rinse Pump COM"() -> (w1560:refnum<visa-resource-name>)
            n967 = local read "Rinse Pump ID"() -> (w1559:i32)
            n968 = local read "Rinse droplet volume [uL]"() -> (w1558:dbl)
            n969 = call "Time Delay25"("error in (no error)"=w1552, "Delay Time (s)"=0.5) -> ("error out"=w1551:errorcluster)  [unwired: 9 in]
            n970 = call "HARVARD_INFUSE_VOLUME_Rinse.vi"("error in (no error)"=w1551, "Volume (uL)"=w1558, "Pump ID"=w1559, "Pump COM"=w1560) -> ("error out"=w1555:errorcluster)  [unwired: 5 in, 2 out]
            n971 = local read "Volume between rinse droplets [uL]"() -> (w1554:dbl)
            n972 = local read "Carrier Pump COM"() -> (w1557:refnum<visa-resource-name>)
            n973 = local read "Carrier Pump ID"() -> (w1556:i32)
            n974 = call "HARVARD_INFUSE_VOLUME.vi"("error in (no error)"=w1555, "Volume (uL)"=w1554, "Pump ID"=w1556, "Pump COM"=w1557) -> ("error out"=w1561:errorcluster)  [unwired: 5 in, 2 out]
          }
          n975 = local read "Transfer lines volume - for rinse/vent operation [uL]"() -> (w1549:dbl)
          n976 = local read "Carrier Pump COM"() -> (w1493:refnum<visa-resource-name>)
          n977 = local read "Carrier Pump ID"() -> (w1492:i32)
          n978 = call "Time Delay26"("error in (no error)"=w1491, "Delay Time (s)"=0.5) -> ("error out"=w1490:errorcluster)  [unwired: 9 in]
          n979 = call "HARVARD_INFUSE_VOLUME.vi"("error in (no error)"=w1490, "Volume (uL)"=w1549, "Pump ID"=w1492, "Pump COM"=w1493) -> ("error out"=w1488:errorcluster, "Pump ID  out"=w1547:u16, "Pump COM out"=w1548:refnum<visa-resource-name>)  [unwired: 5 in]
          n980 = call "Time Delay27"("error in (no error)"=w1488, "Delay Time (s)"=0.5) -> ("error out"=w1487:errorcluster)  [unwired: 9 in]
          n981 = local read "Vent time [s]"() -> (w1533:dbl)
          n982 = local read "Vent Valve Position - Vent"() -> (w1542:string)
          n983 = call "HARVARD_STOP.vi"("error in (no error)"=w1487, "Pump address (0)"=w1547, "VISA resource name"=w1548) -> ("error out"=w1545:errorcluster)  [unwired: 5 in, 2 out]
          n984 = local read "Vent Valve COM"() -> (w1544:refnum<visa-resource-name>)
          n985 = local read "Vent Valve ID"() -> (w1543:i32)
          n986 = Divide(x=w1533, y=2.0) -> (x/y=w1504:dbl)
          n987 = call "VALCO_SET_POS_232.vi"("Error In"=w1545, "New Position (as string)"=w1542, "Valve ID"=w1543, "COM Port In"=w1544) -> ("Error Out"=w1507:errorcluster, "Valve ID out"=w1540:u8, "COM Port Out"=w1541:refnum<visa-resource-name>)  [unwired: 5 in]
          n988 = local read "Transfer lines volume - for rinse/vent operation [uL]"() -> (w1513:dbl)
          n989 = local read "Entrance Volume (reactor phase sensor to reactor center) [uL]"() -> (w1512:dbl)
          n990 = local read "Entrance Volume (sample loop to reactor phase sensor) [uL]"() -> (w1510:dbl)
          n991 = Divide(x=w1504, y=2.0) -> (x/y=w1495:dbl)
          n992 = call "Time Delay10"("error in (no error)"=w1507, "Delay Time (s)"=w1495) -> ("error out"=w1506:errorcluster)  [unwired: 9 in]
          n993 = call "Time Delay33"("error in (no error)"=w1507, "Delay Time (s)"=w1504) -> ("error out"=w1535:errorcluster)  [unwired: 9 in]
          n994 = local read "Vent Valve Position - System"() -> (w1539:string)
          n995 = call "HARVARD_SETFLOWRATE_WITHDRAW.vi"("VISA resource name"=w1493, "Pump address (0)"=w1492, "Withdraw Flow Rate (80)"=7000.0, "error in (no error)"=w1506) -> ("VISA resource name out"=w1517:refnum<visa-resource-name>, "Pump address  out"=w1515:u16, "error out"=w1485:errorcluster)  [unwired: 9 in]
          n996 = call "Time Delay28"("error in (no error)"=w1485, "Delay Time (s)"=0.5) -> ("error out"=w1484:errorcluster)  [unwired: 9 in]
          n997 = Add(x=w1513, y=w1512) -> (x+y=w1511:dbl)
          n998 = local read "Carrier Valve COM"() -> (w1537:refnum<visa-resource-name>)
          n999 = local read "Carrier Valve ID"() -> (w1536:i32)
          n1000 = Add(x=w1511, y=w1510) -> (x+y=w1509:dbl)
          n1001 = local read "Carrier Valve Position - Refill"() -> (w1538:string)
          n1002 = Divide(x=w1509, y=2.0) -> (x/y=w1494:dbl)
          n1003 = call "HARVARD_WITHDRAW_VOLUME.vi"("error in (no error)"=w1484, "Volume (uL)"=w1494, "Pump ID"=w1515, "Pump COM"=w1517) -> ("error out"=w1481:errorcluster, "Pump ID  out"=w1514:u16, "Pump COM out"=w1516:refnum<visa-resource-name>)  [unwired: 5 in]
          n1004 = local read "Carrier Valve Position - System"() -> (w1527:string)
          n1005 = call "Time Delay29"("error in (no error)"=w1481, "Delay Time (s)"=0.5) -> ("error out"=w1480:errorcluster)  [unwired: 9 in]
          n1006 = local read "Carrier Valve COM"() -> (w1528:refnum<visa-resource-name>)
          n1007 = local read "Carrier Valve ID"() -> (w1529:i32)
          n1008 = call "HARVARD_STOP.vi"("error in (no error)"=w1480, "Pump address (0)"=w1514, "VISA resource name"=w1516) -> ()  [unwired: 5 in, 3 out]
          n1009 = call "VALCO_SET_POS_232.vi"("Error In"=w1535, "New Position (as string)"=w1538, "Valve ID"=w1536, "COM Port In"=w1537) -> ("Error Out"=w1496:errorcluster)  [unwired: 5 in, 2 out]
          n1010 = call "Time Delay15"("error in (no error)"=w1496, "Delay Time (s)"=w1495) -> ("error out"=w1501:errorcluster)  [unwired: 9 in]
          n1011 = local read "Vent time [s]"() -> (w1531:dbl)
          n1012 = call "HARVARD_SETFLOWRATE_WITHDRAW.vi"("VISA resource name"=w1493, "Pump address (0)"=w1492, "Withdraw Flow Rate (80)"=7000.0, "error in (no error)"=w1501) -> ("VISA resource name out"=w1497:refnum<visa-resource-name>, "Pump address  out"=w1499:u16, "error out"=w1479:errorcluster)  [unwired: 9 in]
          n1013 = call "Time Delay46"("error in (no error)"=w1479, "Delay Time (s)"=0.5) -> ("error out"=w1478:errorcluster)  [unwired: 9 in]
          n1014 = Divide(x=w1531, y=2.0) -> (x/y=w1532:dbl)
          n1015 = call "Time Delay39"("error in (no error)"=w1496, "Delay Time (s)"=w1532) -> ("error out"=w1530:errorcluster)  [unwired: 9 in]
          n1016 = call "VALCO_SET_POS_232.vi"("Error In"=w1530, "New Position (as string)"=w1539, "Valve ID"=w1540, "COM Port In"=w1541) -> ("Error Out"=w1525:errorcluster)  [unwired: 5 in, 2 out]
          n1017 = call "VALCO_SET_POS_232.vi"("Error In"=w1525, "New Position (as string)"=w1527, "Valve ID"=w1529, "COM Port In"=w1528) -> ("Error Out"=w1524:errorcluster)  [unwired: 5 in, 2 out]
          n1018 = script code="rinse_transfer_lines_last_rxn = rinse_transfer_lines_last_rxn + 1;"("??"=w1524) -> ("rinse_transfer_lines_last_rxn"=w1518:dbl)  [unwired: 1 out]
          n1019 = local write "Reaction number - rinse transfer lines"(w1518) -> ()
          n1020 = call "HARVARD_WITHDRAW_VOLUME.vi"("error in (no error)"=w1478, "Volume (uL)"=w1494, "Pump ID"=w1499, "Pump COM"=w1497) -> ("error out"=w1477:errorcluster, "Pump ID  out"=w1500:u16, "Pump COM out"=w1498:refnum<visa-resource-name>)  [unwired: 5 in]
          n1021 = call "Time Delay65"("error in (no error)"=w1477, "Delay Time (s)"=0.5) -> ("error out"=w1476:errorcluster)  [unwired: 9 in]
          n1022 = call "HARVARD_STOP.vi"("error in (no error)"=w1476, "Pump address (0)"=w1500, "VISA resource name"=w1498) -> ()  [unwired: 5 in, 3 out]
        }
      }
      n1023 = local read "Stop everything"() -> (w1437:bool)
    }
    n1024 = local read "Stop everything"() -> (w1309:bool)
    n1025 = while {
      shift-right: [w1316] -> w1313
      shift-left: w1312 -> [w1315]
      tunnel: w1309 -> [w1314]
      stop <- w1314 stop-if-true
      n1026 = case shown="\"Rinse and vent reactor in progress\"" w1315 {
        tunnel: [w1317 w1326 Rinse_Vent_Reactor_Enum_NSE."Rinse and vent reactor sequence is idle" ("Enum")] -> w1316
        frame "Waiting for hardware initialization", Default {
          n1027 = local read "Ready to start schedule timer"() -> (w1318:bool)
          n1028 = case shown="False" w1318 {
            tunnel: [Rinse_Vent_Reactor_Enum_NSE."Waiting for hardware initialization" ("Enum") Rinse_Vent_Reactor_Enum_NSE."Rinse and vent reactor sequence is idle" ("Enum")] -> w1317
            frame False {
              n1029 = Wait (ms)(milliseconds to wait=500) -> ()  [unwired: 1 out]
            }
            frame True {
              n1030 = script code="rinse_reactor_last_rxn = 0;"("??"=errorcluster {"status"=FALSE, "code"=0, "source"=""} ("error constant")) -> ()  [unwired: 1 out]
            }
          }
        }
        frame "Rinse and vent reactor sequence is idle" {
          n1031 = local read "Schedule - Rinse Reactor"() -> (w1328:dbl[])
          n1032 = script code="rinse_reactor_finished = 0;\nrinse_reactor_next_rxn = rinse_reactor_last_rxn + 1;\nif rinse_reactor_next_rxn <= numel(rinse_reactor_start_times)\n    rinse_reactor_start_times_sorted = sort(rinse_reactor_start_times);\n    rinse_reactor_next_start_time = rinse_reactor_start_times_sorted(rinse_reactor_next_rxn);\nelse\n    rinse_reactor_finished = 1;\nend"("rinse_reactor_start_times"=w1328) -> ("??"=w1325:errorcluster, "rinse_reactor_next_start_time"=w1327:dbl, "rinse_reactor_finished"=w1324:dbl)  [unwired: 1 in]
          n1033 = local write "Next start time - rinse reactor"(w1327) -> ()
          n1034 = Not Equal To 0?(x=w1324) -> (x != 0?=w1323:bool)
          n1035 = local write "rinse_reactor_finished"(w1323) -> ()
          n1036 = while {
            tunnel: [w1339] -> w1326
            tunnel: w1325 -> [w1337]
            stop <- w1329 stop-if-true
            n1037 = local read "Next start time - rinse reactor"() -> (w1340:dbl)
            n1038 = local read "rinse_reactor_finished"() -> (w1335:bool)
            n1039 = local read "Master time [s]"() -> (w1341:dbl)
            n1040 = Less Or Equal?(x=w1340, y=w1341) -> (x <= y?=w1333:bool)
            n1041 = call "Time Delay37"("error in (no error)"=w1337, "Delay Time (s)"=0.5) -> ()  [unwired: 9 in, 1 out]
            n1042 = Not(x=w1335) -> (.not. x?=w1334:bool)
            n1043 = And(x=w1333, y=w1334) -> (x .and. y?=w1332:bool)
            n1044 = case shown="False" w1332 {
              selector: w1332 -> [w1342 w1345]
              tunnel: [Rinse_Vent_Reactor_Enum_NSE."Rinse and vent reactor sequence is idle" ("Enum") Rinse_Vent_Reactor_Enum_NSE."Rinse and vent reactor in progress" ("Enum")] -> w1339
              tunnel: [w1342 w1345] -> w1331
              frame False {
                n1045 = Wait (ms)(milliseconds to wait=500) -> ()  [unwired: 1 out]
              }
              frame True {
              }
            }
            n1046 = Wait (ms)(milliseconds to wait=1000) -> ()  [unwired: 1 out]
            n1047 = local read "schedule_reset"() -> (w1330:bool)
            n1048 = Or(x=w1331, y=w1330) -> (x .or. y?=w1329:bool)
          }
        }
        frame "Rinse and vent reactor in progress" {
          n1049 = local read "Carrier Syringe Infuse\nRate (Rinse) (uL/min)"() -> (w1397:dbl)
          n1050 = local read "Carrier Pump COM"() -> (w1395:refnum<visa-resource-name>)
          n1051 = local read "Carrier Pump ID"() -> (w1396:i32)
          n1052 = local read "Number of rinse droplets"() -> (w1419:i32)
          n1053 = call "HARVARD_SETFLOWRATE_INFUSE.vi"("VISA resource name"=w1395, "Pump address (0)"=w1396, "Infuse Flow Rate (80)"=w1397, "error in (no error)"=errorcluster {"status"=FALSE, "code"=0, "source"=""} ("error constant")) -> ("error out"=w1393:errorcluster)  [unwired: 9 in, 2 out]
          n1054 = for {
            N: w1419 -> [_]
            shift-right: [w1436] -> w1368
            shift-left: w1393 -> [w1427]
            n1055 = local read "Rinse Pump COM"() -> (w1435:refnum<visa-resource-name>)
            n1056 = local read "Rinse Pump ID"() -> (w1434:i32)
            n1057 = local read "Rinse droplet volume [uL]"() -> (w1433:dbl)
            n1058 = call "Time Delay66"("error in (no error)"=w1427, "Delay Time (s)"=0.5) -> ("error out"=w1426:errorcluster)  [unwired: 9 in]
            n1059 = call "HARVARD_INFUSE_VOLUME_Rinse.vi"("error in (no error)"=w1426, "Volume (uL)"=w1433, "Pump ID"=w1434, "Pump COM"=w1435) -> ("error out"=w1430:errorcluster)  [unwired: 5 in, 2 out]
            n1060 = local read "Volume between rinse droplets [uL]"() -> (w1429:dbl)
            n1061 = local read "Carrier Pump COM"() -> (w1432:refnum<visa-resource-name>)
            n1062 = local read "Carrier Pump ID"() -> (w1431:i32)
            n1063 = call "HARVARD_INFUSE_VOLUME.vi"("error in (no error)"=w1430, "Volume (uL)"=w1429, "Pump ID"=w1431, "Pump COM"=w1432) -> ("error out"=w1436:errorcluster)  [unwired: 5 in, 2 out]
          }
          n1064 = local read "Transfer lines plus reactor volume - for rinse/vent operation"() -> (w1423:dbl)
          n1065 = local read "Carrier Pump COM"() -> (w1421:refnum<visa-resource-name>)
          n1066 = local read "Carrier Pump COM"() -> (w1370:refnum<visa-resource-name>)
          n1067 = local read "Carrier Pump ID"() -> (w1422:i32)
          n1068 = local read "Carrier Pump ID"() -> (w1369:i32)
          n1069 = call "Time Delay67"("error in (no error)"=w1368, "Delay Time (s)"=0.5) -> ("error out"=w1367:errorcluster)  [unwired: 9 in]
          n1070 = call "HARVARD_INFUSE_VOLUME.vi"("error in (no error)"=w1367, "Volume (uL)"=w1423, "Pump ID"=w1422, "Pump COM"=w1421) -> ("error out"=w1365:errorcluster, "Pump ID  out"=w1425:u16, "Pump COM out"=w1424:refnum<visa-resource-name>)  [unwired: 5 in]
          n1071 = call "Time Delay68"("error in (no error)"=w1365, "Delay Time (s)"=0.5) -> ("error out"=w1364:errorcluster)  [unwired: 9 in]
          n1072 = local read "Vent Valve Position - Vent"() -> (w1402:string)
          n1073 = local read "Vent time [s]"() -> (w1410:dbl)
          n1074 = call "HARVARD_STOP.vi"("error in (no error)"=w1364, "Pump address (0)"=w1425, "VISA resource name"=w1424) -> ("error out"=w1399:errorcluster)  [unwired: 5 in, 2 out]
          n1075 = local read "Vent Valve COM"() -> (w1400:refnum<visa-resource-name>)
          n1076 = local read "Vent Valve ID"() -> (w1401:i32)
          n1077 = Divide(x=w1410, y=2.0) -> (x/y=w1375:dbl)
          n1078 = call "VALCO_SET_POS_232.vi"("Error In"=w1399, "New Position (as string)"=w1402, "Valve ID"=w1401, "COM Port In"=w1400) -> ("Error Out"=w1373:errorcluster, "Valve ID out"=w1404:u8, "COM Port Out"=w1403:refnum<visa-resource-name>)  [unwired: 5 in]
          n1079 = call "Time Delay34"("error in (no error)"=w1373, "Delay Time (s)"=w1375) -> ("error out"=w1372:errorcluster)  [unwired: 9 in]
          n1080 = local read "Vent Valve Position - System"() -> (w1405:string)
          n1081 = local read "Exit Volume (reactor to sampling valve) [uL]"() -> (w1374:dbl)
          n1082 = local read "Transfer lines plus reactor volume - for rinse/vent operation"() -> (w1348:dbl)
          n1083 = Divide(x=w1375, y=2.0) -> (x/y=w1391:dbl)
          n1084 = local read "Carrier Valve Position - Refill"() -> (w1406:string)
          n1085 = local read "Carrier Valve COM"() -> (w1407:refnum<visa-resource-name>)
          n1086 = local read "Carrier Valve ID"() -> (w1408:i32)
          n1087 = local read "Carrier Valve Position - System"() -> (w1416:string)
          n1088 = call "Time Delay16"("error in (no error)"=w1373, "Delay Time (s)"=w1391) -> ("error out"=w1382:errorcluster)  [unwired: 9 in]
          n1089 = call "HARVARD_SETFLOWRATE_WITHDRAW.vi"("VISA resource name"=w1370, "Pump address (0)"=w1369, "Withdraw Flow Rate (80)"=7000.0, "error in (no error)"=w1382) -> ("VISA resource name out"=w1376:refnum<visa-resource-name>, "Pump address  out"=w1378:u16, "error out"=w1360:errorcluster)  [unwired: 9 in]
          n1090 = call "Time Delay70"("error in (no error)"=w1360, "Delay Time (s)"=0.5) -> ("error out"=w1359:errorcluster)  [unwired: 9 in]
          n1091 = Add(x=w1348, y=50.0) -> (x+y=w1347:dbl)
          n1092 = Add(x=w1374, y=w1347) -> (x+y=w1380:dbl)
          n1093 = Divide(x=w1380, y=2.0) -> (x/y=w1392:dbl)
          n1094 = call "HARVARD_WITHDRAW_VOLUME.vi"("error in (no error)"=w1359, "Volume (uL)"=w1392, "Pump ID"=w1378, "Pump COM"=w1376) -> ("error out"=w1357:errorcluster, "Pump ID  out"=w1379:u16, "Pump COM out"=w1377:refnum<visa-resource-name>)  [unwired: 5 in]
          n1095 = call "Time Delay71"("error in (no error)"=w1357, "Delay Time (s)"=0.5) -> ("error out"=w1356:errorcluster)  [unwired: 9 in]
          n1096 = call "Time Delay69"("Delay Time (s)"=0.5) -> ()  [unwired: 10 in, 1 out]
          n1097 = call "HARVARD_STOP.vi"("error in (no error)"=w1356, "Pump address (0)"=w1379, "VISA resource name"=w1377) -> ()  [unwired: 5 in, 3 out]
          n1098 = local read "Carrier Valve COM"() -> (w1415:refnum<visa-resource-name>)
          n1099 = local read "Vent time [s]"() -> (w1412:dbl)
          n1100 = local read "Carrier Valve ID"() -> (w1414:i32)
          n1101 = call "VALCO_SET_POS_232.vi"("Error In"=w1372, "New Position (as string)"=w1406, "Valve ID"=w1408, "COM Port In"=w1407) -> ("Error Out"=w1371:errorcluster)  [unwired: 5 in, 2 out]
          n1102 = call "Time Delay17"("error in (no error)"=w1371, "Delay Time (s)"=w1391) -> ("error out"=w1386:errorcluster)  [unwired: 9 in]
          n1103 = Divide(x=w1412, y=2.0) -> (x/y=w1411:dbl)
          n1104 = call "Time Delay40"("error in (no error)"=w1371, "Delay Time (s)"=w1411) -> ("error out"=w1413:errorcluster)  [unwired: 9 in]
          n1105 = call "VALCO_SET_POS_232.vi"("Error In"=w1413, "New Position (as string)"=w1405, "Valve ID"=w1404, "COM Port In"=w1403) -> ("Error Out"=w1418:errorcluster)  [unwired: 5 in, 2 out]
          n1106 = call "VALCO_SET_POS_232.vi"("Error In"=w1418, "New Position (as string)"=w1416, "Valve ID"=w1414, "COM Port In"=w1415) -> ("Error Out"=w1398:errorcluster)  [unwired: 5 in, 2 out]
          n1107 = script code="rinse_reactor_last_rxn = rinse_reactor_last_rxn + 1;"("??"=w1398) -> ()  [unwired: 1 out]
          n1108 = call "HARVARD_SETFLOWRATE_WITHDRAW.vi"("VISA resource name"=w1370, "Pump address (0)"=w1369, "Withdraw Flow Rate (80)"=7000.0, "error in (no error)"=w1386) -> ("VISA resource name out"=w1390:refnum<visa-resource-name>, "Pump address  out"=w1388:u16, "error out"=w1353:errorcluster)  [unwired: 9 in]
          n1109 = call "Time Delay72"("error in (no error)"=w1353, "Delay Time (s)"=0.5) -> ("error out"=w1352:errorcluster)  [unwired: 9 in]
          n1110 = call "HARVARD_WITHDRAW_VOLUME.vi"("error in (no error)"=w1352, "Volume (uL)"=w1392, "Pump ID"=w1388, "Pump COM"=w1390) -> ("error out"=w1351:errorcluster, "Pump ID  out"=w1387:u16, "Pump COM out"=w1389:refnum<visa-resource-name>)  [unwired: 5 in]
          n1111 = call "Time Delay73"("error in (no error)"=w1351, "Delay Time (s)"=0.5) -> ("error out"=w1350:errorcluster)  [unwired: 9 in]
          n1112 = call "HARVARD_STOP.vi"("error in (no error)"=w1350, "Pump address (0)"=w1387, "VISA resource name"=w1389) -> ()  [unwired: 5 in, 3 out]
        }
      }
    }
  }
  n1113 = while {
    shift-right: [w1565] -> _
    shift-left: Transport_to_Analysis_Enum_NSE."Waiting for hardware initialization" ("Enum") -> [w1563]
    stop <- w1564 stop-if-true
    n1114 = case shown="\"Transport sequence is idle\"" w1563 {
      tunnel: [w1566 w1582 Transport_to_Analysis_Enum_NSE."Transport sequence is idle" ("Enum")] -> w1565
      frame "Waiting for hardware initialization", Default {
        n1115 = local read "Ready to start schedule timer"() -> (w1567:bool)
        n1116 = case shown="False" w1567 {
          tunnel: [Transport_to_Analysis_Enum_NSE."Waiting for hardware initialization" ("Enum") Transport_to_Analysis_Enum_NSE."Transport sequence is idle" ("Enum")] -> w1566
          frame False {
          }
          frame True {
          }
        }
      }
      frame "Transport sequence is idle" {
        n1117 = local read "Reaction number - transport from reactor to analysis"() -> (w1584:dbl)
        n1118 = local read "Analytical method length [s]"() -> (w1574:dbl)
        n1119 = local read "Schedule - Reactor to Analysis"() -> (w1585:dbl[])
        n1120 = script code="reactor_to_analysis_finished = 0;\nanalysis_finished = 0;\nreactor_to_analysis_next_rxn = reactor_to_analysis_last_rxn + 1;\nif reactor_to_analysis_next_rxn <= numel(reactor_to_analysis_start_times)\n    reactor_to_analysis_start_times_sorted = sort(reactor_to_analysis_start_times);\n    reactor_to_analysis_next_start_time = reactor_to_analysis_start_times_sorted(reactor_to_analysis_next_rxn);\n    index_reactor_to_analysis_next_rxn = find(reactor_to_analysis_start_times == reactor_to_analysis_next_start_time);\n    next_analysis_time = reactor_to_analysis_next_start_time + ana_time + 30; % 30s buffer for processing\n    reactor_to_analysis_reactor_assignment = num2str(all_slugs(index_reactor_to_analysis_next_rxn).assigned_reactor);\nelse\n    reactor_to_analysis_finished = 1;\n    reactor_to_analysis_reactor_assignment = 0;\nend"("??"=errorcluster {"status"=FALSE, "code"=0, "source"=""} ("error constant"), "reactor_to_analysis_start_times"=w1585, "reactor_to_analysis_last_rxn"=w1584, "ana_time"=w1574) -> ("??"=w1579:errorcluster, "reactor_to_analysis_next_start_time"=w1583:dbl, "reactor_to_analysis_reactor_assignment"=w1581:string, "reactor_to_analysis_finished"=w1576:dbl, "next_analysis_time"=w1573:dbl, "analysis_finished"=w1572:dbl, "index_reactor_to_analysis_next_rxn"=w1570:dbl)
        n1121 = local write "Index_Ana_Rxn"(w1570) -> ()
        n1122 = local write "Reactor assignment - transport from reactor to analysis"(w1581) -> ()
        n1123 = local write "Next start time - transport from reactor to analysis"(w1583) -> ()
        n1124 = local write "Next analysis time"(w1573) -> ()
        n1125 = call "Time Delay31"("error in (no error)"=w1579, "Delay Time (s)"=1.0) -> ("error out"=w1578:errorcluster)  [unwired: 9 in]
        n1126 = Not Equal To 0?(x=w1572) -> (x != 0?=w1571:bool)
        n1127 = Not Equal To 0?(x=w1576) -> (x != 0?=w1575:bool)
        n1128 = while {
          tunnel: [w1597] -> w1582
          tunnel: w1578 -> [w1596]
          stop <- w1586 stop-if-true
          n1129 = local read "Next start time - transport from reactor to analysis"() -> (w1599:dbl)
          n1130 = local read "Master time [s]"() -> (w1598:dbl)
          n1131 = call "Time Delay14"("error in (no error)"=w1596, "Delay Time (s)"=0.5) -> ()  [unwired: 9 in, 1 out]
          n1132 = local read "reactor_to_analysis_finished"() -> (w1590:bool)
          n1133 = local write "Phase Sensor Reading Start - Analytical Valve [s]"(1000000000000000.0) -> ()
          n1134 = local write "Phase Sensor Detection - Analytical Valve"(FALSE) -> ()
          n1135 = Not(x=w1590) -> (.not. x?=w1589:bool)
          n1136 = Less Or Equal?(x=w1599, y=w1598) -> (x <= y?=w1592:bool)
          n1137 = And(x=w1592, y=w1589) -> (x .and. y?=w1591:bool)
          n1138 = local read "schedule_reset"() -> (w1587:bool)
          n1139 = case shown="False" w1591 {
            selector: w1591 -> [w1601 w1604]
            tunnel: [Transport_to_Analysis_Enum_NSE."Transport sequence is idle" ("Enum") Transport_to_Analysis_Enum_NSE."Transport in progress" ("Enum")] -> w1597
            tunnel: [w1601 w1604] -> w1588
            frame False {
              n1140 = Wait (ms)(milliseconds to wait=500) -> ()  [unwired: 1 out]
            }
            frame True {
              n1141 = Wait (ms)(milliseconds to wait=500) -> ()  [unwired: 1 out]
            }
          }
          n1142 = Or(x=w1588, y=w1587) -> (x .or. y?=w1586:bool)
        }
        n1143 = local write "reactor_to_analysis_finished"(w1575) -> ()
        n1144 = local write "analysis_finished"(w1571) -> ()
      }
      frame "Transport in progress" {
        # "Switch analytical valve to HPLC and back"
        n1145 = local read "Reactor assignment - transport from reactor to analysis"() -> (w1637:string)
        n1146 = local read "Reactor Selector Valve\n - Upstream - COM"() -> (w1639:refnum<visa-resource-name>)
        n1147 = local read "Reactor Selector Valve Upstream ID"() -> (w1638:i32)
        n1148 = call "VALCO_SET_POS_232.vi"("Error In"=errorcluster {"status"=FALSE, "code"=0, "source"=""} ("error constant"), "New Position (as string)"=w1637, "Valve ID"=w1638, "COM Port In"=w1639) -> ("Error Out"=w1634:errorcluster)  [unwired: 5 in, 2 out]
        n1149 = local read "Reactor Selector Valve Downstream COM"() -> (w1636:refnum<visa-resource-name>)
        n1150 = local read "Reactor Selector Valve Downstream ID"() -> (w1635:i32)
        n1151 = local read "Carrier Syringe Infuse Rate\n(Droplet Transport) [uL/min]"() -> (w1612:dbl)
        n1152 = call "VALCO_SET_POS_232.vi"("Error In"=w1634, "New Position (as string)"=w1637, "Valve ID"=w1635, "COM Port In"=w1636) -> ("Error Out"=w1617:errorcluster)  [unwired: 5 in, 2 out]
        n1153 = call "Time Delay41"("error in (no error)"=w1617, "Delay Time (s)"=5) -> ("error out"=w1616:errorcluster)  [unwired: 9 in]
        n1154 = case shown="\"1\", Default" w1637 {
          tunnel: w1616 -> [w1668 w1673 w1678 w1683 w1688 w1693 w1698 w1703 w1708 w1713]
          tunnel: [w1667 w1672 w1677 w1682 w1687 w1692 w1697 w1702 w1707 w1712] -> w1611
          frame "1", Default {
            n1155 = local read "Reactor Valve 1 Position - System"() -> (w1669:string)
            n1156 = local read "Reactor Valve 1 COM"() -> (w1671:refnum<visa-resource-name>)
            n1157 = local read "Reactor Valve 1 ID"() -> (w1670:i32)
            n1158 = call "VALCO_SET_POS_232.vi"("Error In"=w1668, "New Position (as string)"=w1669, "Valve ID"=w1670, "COM Port In"=w1671) -> ("Error Out"=w1667:errorcluster)  [unwired: 5 in, 2 out]
          }
          frame "2" {
            n1159 = local read "Reactor Valve 2 Position - System"() -> (w1674:string)
            n1160 = local read "Reactor Valve 2 COM"() -> (w1676:refnum<visa-resource-name>)
            n1161 = local read "Reactor Valve 2 ID"() -> (w1675:i32)
            n1162 = call "VALCO_SET_POS_232.vi"("Error In"=w1673, "New Position (as string)"=w1674, "Valve ID"=w1675, "COM Port In"=w1676) -> ("Error Out"=w1672:errorcluster)  [unwired: 5 in, 2 out]
          }
          frame "3" {
            n1163 = local read "Reactor Valve 3 Position - System"() -> (w1679:string)
            n1164 = local read "Reactor Valve 3 COM"() -> (w1681:refnum<visa-resource-name>)
            n1165 = local read "Reactor Valve 3 ID"() -> (w1680:dbl)
            n1166 = call "VALCO_SET_POS_232.vi"("Error In"=w1678, "New Position (as string)"=w1679, "Valve ID"=w1680, "COM Port In"=w1681) -> ("Error Out"=w1677:errorcluster)  [unwired: 5 in, 2 out]
          }
          frame "4" {
            n1167 = local read "Reactor Valve 4 Position - System"() -> (w1684:string)
            n1168 = local read "Reactor Valve 4 COM"() -> (w1686:refnum<visa-resource-name>)
            n1169 = local read "Reactor Valve 4 ID"() -> (w1685:dbl)
            n1170 = call "VALCO_SET_POS_232.vi"("Error In"=w1683, "New Position (as string)"=w1684, "Valve ID"=w1685, "COM Port In"=w1686) -> ("Error Out"=w1682:errorcluster)  [unwired: 5 in, 2 out]
          }
          frame "5" {
            n1171 = local read "Reactor Valve 5 Position - System"() -> (w1689:string)
            n1172 = local read "Reactor Valve 5 COM"() -> (w1691:refnum<visa-resource-name>)
            n1173 = local read "Reactor Valve 5 ID"() -> (w1690:dbl)
            n1174 = call "VALCO_SET_POS_232.vi"("Error In"=w1688, "New Position (as string)"=w1689, "Valve ID"=w1690, "COM Port In"=w1691) -> ("Error Out"=w1687:errorcluster)  [unwired: 5 in, 2 out]
          }
          frame "6" {
            n1175 = local read "Reactor Valve 6 Position - System"() -> (w1694:string)
            n1176 = local read "Reactor Valve 6 COM"() -> (w1696:refnum<visa-resource-name>)
            n1177 = local read "Reactor Valve 6 ID"() -> (w1695:dbl)
            n1178 = call "VALCO_SET_POS_232.vi"("Error In"=w1693, "New Position (as string)"=w1694, "Valve ID"=w1695, "COM Port In"=w1696) -> ("Error Out"=w1692:errorcluster)  [unwired: 5 in, 2 out]
          }
          frame "7" {
            n1179 = local read "Reactor Valve 7 Position - System"() -> (w1699:string)
            n1180 = local read "Reactor Valve 7 COM"() -> (w1701:refnum<visa-resource-name>)
            n1181 = local read "Reactor Valve 7 ID"() -> (w1700:dbl)
            n1182 = call "VALCO_SET_POS_232.vi"("Error In"=w1698, "New Position (as string)"=w1699, "Valve ID"=w1700, "COM Port In"=w1701) -> ("Error Out"=w1697:errorcluster)  [unwired: 5 in, 2 out]
          }
          frame "8" {
            n1183 = local read "Reactor Valve 8 Position - System"() -> (w1704:string)
            n1184 = local read "Reactor Valve 8 COM"() -> (w1706:refnum<visa-resource-name>)
            n1185 = local read "Reactor Valve 8 ID"() -> (w1705:dbl)
            n1186 = call "VALCO_SET_POS_232.vi"("Error In"=w1703, "New Position (as string)"=w1704, "Valve ID"=w1705, "COM Port In"=w1706) -> ("Error Out"=w1702:errorcluster)  [unwired: 5 in, 2 out]
          }
          frame "9" {
            n1187 = local read "Reactor Valve 9 Position - System"() -> (w1711:string)
            n1188 = local read "Reactor Valve 9 COM"() -> (w1709:refnum<visa-resource-name>)
            n1189 = local read "Reactor Valve 9 ID"() -> (w1710:dbl)
            n1190 = call "VALCO_SET_POS_232.vi"("Error In"=w1708, "New Position (as string)"=w1711, "Valve ID"=w1710, "COM Port In"=w1709) -> ("Error Out"=w1707:errorcluster)  [unwired: 5 in, 2 out]
          }
          frame "10" {
            n1191 = local read "Reactor Valve 10 Position - System"() -> (w1714:string)
            n1192 = local read "Reactor Valve 10 COM"() -> (w1716:refnum<visa-resource-name>)
            n1193 = local read "Reactor Valve 10 ID"() -> (w1715:dbl)
            n1194 = call "VALCO_SET_POS_232.vi"("Error In"=w1713, "New Position (as string)"=w1714, "Valve ID"=w1715, "COM Port In"=w1716) -> ("Error Out"=w1712:errorcluster)  [unwired: 5 in, 2 out]
          }
        }
        n1195 = local read "Carrier Pump COM"() -> (w1614:refnum<visa-resource-name>)
        n1196 = local read "Carrier Pump ID"() -> (w1613:i32)
        n1197 = call "HARVARD_SETFLOWRATE_INFUSE.vi"("VISA resource name"=w1614, "Pump address (0)"=w1613, "Infuse Flow Rate (80)"=w1612, "error in (no error)"=w1611) -> ("error out"=w1607:errorcluster)  [unwired: 9 in, 2 out]
        n1198 = local read "Carrier Pump COM"() -> (w1632:refnum<visa-resource-name>)
        n1199 = local read "Carrier Pump ID"() -> (w1631:i32)
        n1200 = call "Time Delay74"("error in (no error)"=w1607, "Delay Time (s)"=0.5) -> ("error out"=w1606:errorcluster)  [unwired: 9 in]
        n1201 = local read "Exit Volume (reactor to sampling valve) [uL]"() -> (w1630:dbl)
        n1202 = call "HARVARD_INFUSE_VOLUME.vi"("error in (no error)"=w1606, "Volume (uL)"=w1630, "Pump ID"=w1631, "Pump COM"=w1632) -> ("error out"=w1619:errorcluster)  [unwired: 5 in, 2 out]
        n1203 = while {
          tunnel: w1619 -> [w1642]
          tunnel: [w1640] -> w1620
          stop <- w1647 stop-if-true
          n1204 = local read "Phase Sensor Liquid Threshold - Analytical Valve"() -> (w1645:dbl)
          n1205 = local read "Phase Sensor Reading - Analytical Valve"() -> (w1646:dbl)
          n1206 = Greater?(x=w1646, y=w1645) -> (0:w1644:bool)
          n1207 = call "Time Delay35"("error in (no error)"=w1642, "Delay Time (s)"=0.5) -> ("error out"=w1641:errorcluster)  [unwired: 9 in]
          n1208 = case shown="False" w1644 {
            tunnel: w1641 -> [w1649 w1657]
            tunnel: [w1648 w1657] -> w1640
            frame False {
              n1209 = local read "Master time [s]"() -> (w1653:dbl)
              n1210 = local read "Carrier Pump ID"() -> (w1652:i32)
              n1211 = local read "Carrier Pump COM"() -> (w1651:refnum<visa-resource-name>)
              n1212 = call "HARVARD_INFUSE_VOLUME.vi"("error in (no error)"=w1649, "Volume (uL)"=10.0, "Pump ID"=w1652, "Pump COM"=w1651) -> ("error out"=w1648:errorcluster)  [unwired: 5 in, 2 out]
              n1213 = local write "Phase Sensor Reading Start - Analytical Valve [s]"(w1653) -> ()
            }
            frame True {
              n1214 = local read "Phase Sensor - Analytical Valve - Minimum Liquid Length [s]"() -> (w1659:dbl)
              n1215 = local read "Phase Sensor Reading Start - Analytical Valve [s]"() -> (w1655:dbl)
              n1216 = local read "Master time [s]"() -> (w1654:dbl)
              n1217 = local read "Phase Sensor Reading Start - Analytical Valve [s]"() -> (w1661:dbl)
              n1218 = local read "Master time [s]"() -> (w1662:dbl)
              n1219 = Less?(x=w1654, y=w1655) -> (x < y?=w1656:bool)
              n1220 = case shown="True" w1656 {
                frame False {
                }
                frame True {
                  n1221 = local read "Master time [s]"() -> (w1663:dbl)
                  n1222 = local write "Phase Sensor Reading Start - Analytical Valve [s]"(w1663) -> ()
                }
              }
              n1223 = Subtract(x=w1662, y=w1661) -> (x-y=w1660:dbl)
              n1224 = Greater?(x=w1660, y=w1659) -> (0:w1658:bool)
              n1225 = case shown="True" w1658 {
                frame False {
                  n1226 = Wait (ms)(milliseconds to wait=50) -> ()  [unwired: 1 out]
                }
                frame True {
                  n1227 = local write "Phase Sensor Detection - Analytical Valve"(TRUE) -> ()
                  n1228 = Wait (ms)(milliseconds to wait=50) -> ()  [unwired: 1 out]
                }
              }
            }
          }
          n1229 = local read "Phase Sensor Detection - Analytical Valve"() -> (w1647:bool)
        }
        n1230 = script code="reactor_to_analysis_last_rxn = reactor_to_analysis_last_rxn + 1;"("??"=w1619) -> ("reactor_to_analysis_last_rxn"=w1618:dbl)  [unwired: 1 out]
        n1231 = local write "Reaction number - transport from reactor to analysis"(w1618) -> ()
        n1232 = local read "Analytical Valve Position - HPLC"() -> (w1626:string)
        n1233 = local read "Analytical Valve COM"() -> (w1628:refnum<visa-resource-name>)
        n1234 = local read "Analytical Valve ID"() -> (w1627:i32)
        n1235 = call "VALCO_SET_POS_232.vi"("Error In"=w1620, "New Position (as string)"=w1626, "Valve ID"=w1627, "COM Port In"=w1628) -> ("Error Out"=w1610:errorcluster, "Valve ID out"=w1622:u8, "COM Port Out"=w1623:refnum<visa-resource-name>)  [unwired: 5 in]
        n1236 = local read "Analytical Valve Position - System"() -> (w1621:string)
        n1237 = call "Start_Stop_HPLC.vi"("ChemStation Name"="ChemStation Name", "error in (no error)"=w1610) -> ()  [unwired: 9 in]
        n1238 = call "Time Delay4"("error in (no error)"=w1610, "Delay Time (s)"=0.5) -> ("error out"=w1624:errorcluster)  [unwired: 9 in]
        n1239 = call "VALCO_SET_POS_232.vi"("Error In"=w1624, "New Position (as string)"=w1621, "Valve ID"=w1622, "COM Port In"=w1623) -> ()  [unwired: 5 in, 3 out]
      }
    }
    n1240 = Wait (ms)(milliseconds to wait=1000) -> ()  [unwired: 1 out]
    n1241 = local read "Stop everything"() -> (w1564:bool)
  }
  n1242 = while {
    shift-right: [w1720] -> _
    shift-left: Transport_to_Reactor_Enum_NSE."Waiting for hardware initialization" ("Enum") -> [w1717]
    stop <- w1719 stop-if-true
    n1243 = case shown="\"Transport in progress\"" w1717 {
      tunnel: [w1721 w1733 Transport_to_Reactor_Enum_NSE."Transport sequence is idle" ("Enum")] -> w1720
      frame "Waiting for hardware initialization", Default {
        n1244 = local read "Ready to start schedule timer"() -> (w1722:bool)
        n1245 = case shown="True" w1722 {
          tunnel: [Transport_to_Reactor_Enum_NSE."Waiting for hardware initialization" ("Enum") Transport_to_Reactor_Enum_NSE."Transport sequence is idle" ("Enum")] -> w1721
          frame False {
            n1246 = Wait (ms)(milliseconds to wait=500) -> ()  [unwired: 1 out]
          }
          frame True {
          }
        }
      }
      frame "Transport sequence is idle" {
        # "Reset reactor phase sensor detection boolean to false\nand the phase sensor reading start time to a large number"
        n1247 = local read "Reaction number - transport to reactor"() -> (w1735:dbl)
        n1248 = local read "Schedule - Liquid Handler to Reactor"() -> (w1736:dbl[])
        n1249 = local write "Phase Sensor Reading Start - Reactor [s]"(1000000000000000.0) -> ()
        n1250 = local write "Phase Sensor Detection - Reactor"(FALSE) -> ()
        n1251 = script code="loop_to_reactor_finished = 0;\nloop_to_reactor_next_rxn = loop_to_reactor_last_rxn + 1;\nif loop_to_reactor_next_rxn <= numel(loop_to_reactor_start_times)\n    loop_to_reactor_next_start_time = loop_to_reactor_start_times(loop_to_reactor_next_rxn);\n    loop_to_reactor_reactor_assignment = num2str(all_slugs(loop_to_reactor_next_rxn).assigned_reactor);\nelse\n    loop_to_reactor_finished = 1;\n    loop_to_reactor_reactor_assignment = 0;\nend"("??"=errorcluster {"status"=FALSE, "code"=0, "source"=""} ("error constant"), "loop_to_reactor_start_times"=w1736, "loop_to_reactor_last_rxn"=w1735) -> ("??"=w1728:errorcluster, "loop_to_reactor_next_start_time"=w1734:dbl, "loop_to_reactor_reactor_assignment"=w1732:string, "loop_to_reactor_finished"=w1727:dbl)
        n1252 = local write "Reactor assignment - transport from loop to reactor"(w1732) -> ()
        n1253 = local write "Next start time - transport from loop to reactor"(w1734) -> ()
        n1254 = Not Equal To 0?(x=w1727) -> (x != 0?=w1726:bool)
        n1255 = while {
          tunnel: [w1749] -> w1733
          tunnel: w1728 -> [w1745]
          stop <- w1737 stop-if-true
          n1256 = local read "Next start time - transport from loop to reactor"() -> (w1751:dbl)
          n1257 = call "Time Delay32"("error in (no error)"=w1745, "Delay Time (s)"=0.5) -> ()  [unwired: 9 in, 1 out]
          n1258 = local read "Phase Sensor Detection - Injection Valve"() -> (w1747:bool)
          n1259 = local read "Master time [s]"() -> (w1750:dbl)
          n1260 = local read "loop_to_reactor_finished"() -> (w1741:bool)
          n1261 = Less Or Equal?(x=w1751, y=w1750) -> (x <= y?=w1748:bool)
          n1262 = And(x=w1748, y=w1747) -> (x .and. y?=w1743:bool)
          n1263 = Not(x=w1741) -> (.not. x?=w1740:bool)
          n1264 = And(x=w1743, y=w1740) -> (x .and. y?=w1742:bool)
          n1265 = Wait (ms)(milliseconds to wait=500) -> ()  [unwired: 1 out]
          n1266 = case shown="False" w1742 {
            selector: w1742 -> [w1752 w1754]
            tunnel: [Transport_to_Reactor_Enum_NSE."Transport sequence is idle" ("Enum") Transport_to_Reactor_Enum_NSE."Transport in progress" ("Enum")] -> w1749
            tunnel: [w1752 w1754] -> w1738
            frame False {
            }
            frame True {
              # "Reset injection valve phase sensor detection boolean to false"
              n1267 = local write "Phase Sensor Detection - Injection Valve"(FALSE) -> ()
            }
          }
          n1268 = local read "schedule_reset"() -> (w1739:bool)
          n1269 = Or(x=w1738, y=w1739) -> (x .or. y?=w1737:bool)
        }
        n1270 = local write "loop_to_reactor_finished"(w1726) -> ()
      }
      frame "Transport in progress" {
        w1786 = errorcluster {"status"=FALSE, "code"=0, "source"=""} ("error constant")
        # "pause briefly between setting the\nselector valve positions and switching\nthe injection valve - to allow pressure\non the new reactor line to equilibrate"
        # "Once phase sensor detects droplet,\ninfuse a little more to get the droplet\ncentered in the reactor"
        # "Before opening the injection\nvalve, open selector valve to\ncorrect reactor, and open\ncorrect reactor's reactor valve\nto system"
        n1271 = local read "Reactor assignment - transport from loop to reactor"() -> (w1779:string)
        n1272 = case shown="\"1\", Default" w1779 {
          tunnel: w1786 -> [w1798 w1802 w1806 w1810 w1814 w1818 w1822 w1826 w1830 w1834]
          frame "1", Default {
            n1273 = local read "Reactor Valve 1 Position - System"() -> (w1799:string)
            n1274 = local read "Reactor Valve 1 COM"() -> (w1801:refnum<visa-resource-name>)
            n1275 = local read "Reactor Valve 1 ID"() -> (w1800:i32)
            n1276 = call "VALCO_SET_POS_232.vi"("Error In"=w1798, "New Position (as string)"=w1799, "Valve ID"=w1800, "COM Port In"=w1801) -> ()  [unwired: 5 in, 3 out]
          }
          frame "2" {
            n1277 = local read "Reactor Valve 2 Position - System"() -> (w1803:string)
            n1278 = local read "Reactor Valve 2 COM"() -> (w1805:refnum<visa-resource-name>)
            n1279 = local read "Reactor Valve 2 ID"() -> (w1804:i32)
            n1280 = call "VALCO_SET_POS_232.vi"("Error In"=w1802, "New Position (as string)"=w1803, "Valve ID"=w1804, "COM Port In"=w1805) -> ()  [unwired: 5 in, 3 out]
          }
          frame "3" {
            n1281 = local read "Reactor Valve 3 Position - System"() -> (w1807:string)
            n1282 = local read "Reactor Valve 3 COM"() -> (w1809:refnum<visa-resource-name>)
            n1283 = local read "Reactor Valve 3 ID"() -> (w1808:dbl)
            n1284 = call "VALCO_SET_POS_232.vi"("Error In"=w1806, "New Position (as string)"=w1807, "Valve ID"=w1808, "COM Port In"=w1809) -> ()  [unwired: 5 in, 3 out]
          }
          frame "4" {
            n1285 = local read "Reactor Valve 4 Position - System"() -> (w1811:string)
            n1286 = local read "Reactor Valve 4 COM"() -> (w1813:refnum<visa-resource-name>)
            n1287 = local read "Reactor Valve 4 ID"() -> (w1812:dbl)
            n1288 = call "VALCO_SET_POS_232.vi"("Error In"=w1810, "New Position (as string)"=w1811, "Valve ID"=w1812, "COM Port In"=w1813) -> ()  [unwired: 5 in, 3 out]
          }
          frame "5" {
            n1289 = local read "Reactor Valve 5 Position - System"() -> (w1815:string)
            n1290 = local read "Reactor Valve 5 COM"() -> (w1817:refnum<visa-resource-name>)
            n1291 = local read "Reactor Valve 5 ID"() -> (w1816:dbl)
            n1292 = call "VALCO_SET_POS_232.vi"("Error In"=w1814, "New Position (as string)"=w1815, "Valve ID"=w1816, "COM Port In"=w1817) -> ()  [unwired: 5 in, 3 out]
          }
          frame "6" {
            n1293 = local read "Reactor Valve 6 Position - System"() -> (w1819:string)
            n1294 = local read "Reactor Valve 6 COM"() -> (w1821:refnum<visa-resource-name>)
            n1295 = local read "Reactor Valve 6 ID"() -> (w1820:dbl)
            n1296 = call "VALCO_SET_POS_232.vi"("Error In"=w1818, "New Position (as string)"=w1819, "Valve ID"=w1820, "COM Port In"=w1821) -> ()  [unwired: 5 in, 3 out]
          }
          frame "7" {
            n1297 = local read "Reactor Valve 7 Position - System"() -> (w1823:string)
            n1298 = local read "Reactor Valve 7 COM"() -> (w1825:refnum<visa-resource-name>)
            n1299 = local read "Reactor Valve 7 ID"() -> (w1824:dbl)
            n1300 = call "VALCO_SET_POS_232.vi"("Error In"=w1822, "New Position (as string)"=w1823, "Valve ID"=w1824, "COM Port In"=w1825) -> ()  [unwired: 5 in, 3 out]
          }
          frame "8" {
            n1301 = local read "Reactor Valve 8 Position - System"() -> (w1827:string)
            n1302 = local read "Reactor Valve 8 COM"() -> (w1829:refnum<visa-resource-name>)
            n1303 = local read "Reactor Valve 8 ID"() -> (w1828:dbl)
            n1304 = call "VALCO_SET_POS_232.vi"("Error In"=w1826, "New Position (as string)"=w1827, "Valve ID"=w1828, "COM Port In"=w1829) -> ()  [unwired: 5 in, 3 out]
          }
          frame "9" {
            n1305 = local read "Reactor Valve 9 Position - System"() -> (w1833:string)
            n1306 = local read "Reactor Valve 9 COM"() -> (w1831:refnum<visa-resource-name>)
            n1307 = local read "Reactor Valve 9 ID"() -> (w1832:dbl)
            n1308 = call "VALCO_SET_POS_232.vi"("Error In"=w1830, "New Position (as string)"=w1833, "Valve ID"=w1832, "COM Port In"=w1831) -> ()  [unwired: 5 in, 3 out]
          }
          frame "10" {
            n1309 = local read "Reactor Valve 10 Position - System"() -> (w1835:string)
            n1310 = local read "Reactor Valve 10 COM"() -> (w1837:refnum<visa-resource-name>)
            n1311 = local read "Reactor Valve 10 ID"() -> (w1836:dbl)
            n1312 = call "VALCO_SET_POS_232.vi"("Error In"=w1834, "New Position (as string)"=w1835, "Valve ID"=w1836, "COM Port In"=w1837) -> ()  [unwired: 5 in, 3 out]
          }
        }
        n1313 = local read "Reactor Selector Valve Downstream COM"() -> (w1791:refnum<visa-resource-name>)
        n1314 = local read "Reactor Selector Valve Downstream ID"() -> (w1790:i32)
        n1315 = local read "Reactor Selector Valve\n - Upstream - COM"() -> (w1793:refnum<visa-resource-name>)
        n1316 = local read "Reactor Selector Valve Upstream ID"() -> (w1792:i32)
        n1317 = call "VALCO_SET_POS_232.vi"("Error In"=w1786, "New Position (as string)"=w1779, "Valve ID"=w1790, "COM Port In"=w1791) -> ("Error Out"=w1777:errorcluster)  [unwired: 5 in, 2 out]
        n1318 = call "VALCO_SET_POS_232.vi"("Error In"=w1786, "New Position (as string)"=w1779, "Valve ID"=w1792, "COM Port In"=w1793) -> ()  [unwired: 5 in, 3 out]
        n1319 = local read "Injection Valve COM"() -> (w1795:refnum<visa-resource-name>)
        n1320 = local read "Injection Valve ID"() -> (w1796:i32)
        n1321 = local read "Injection Valve Position - System"() -> (w1797:string)
        n1322 = call "Time Delay38"("error in (no error)"=w1777, "Delay Time (s)"=5.0) -> ("error out"=w1776:errorcluster)  [unwired: 9 in]
        n1323 = local read "Carrier Syringe Infuse Rate\n(Droplet Transport) [uL/min]"() -> (w1772:dbl)
        n1324 = local read "Entrance Volume (sample loop to reactor phase sensor) [uL]"() -> (w1782:dbl)
        n1325 = call "VALCO_SET_POS_232.vi"("Error In"=w1776, "New Position (as string)"=w1797, "Valve ID"=w1796, "COM Port In"=w1795) -> ("Error Out"=w1775:errorcluster)  [unwired: 5 in, 2 out]
        n1326 = local read "Carrier Pump ID"() -> (w1774:i32)
        n1327 = local read "Carrier Pump COM"() -> (w1773:refnum<visa-resource-name>)
        n1328 = call "HARVARD_SETFLOWRATE_INFUSE.vi"("VISA resource name"=w1773, "Pump address (0)"=w1774, "Infuse Flow Rate (80)"=w1772, "error in (no error)"=w1775) -> ("error out"=w1762:errorcluster)  [unwired: 9 in, 2 out]
        n1329 = call "Time Delay23"("error in (no error)"=w1762, "Delay Time (s)"=0.5) -> ("error out"=w1761:errorcluster)  [unwired: 9 in]
        n1330 = call "HARVARD_INFUSE_VOLUME.vi"("error in (no error)"=w1761, "Volume (uL)"=w1782, "Pump ID"=w1774, "Pump COM"=w1773) -> ("error out"=w1767:errorcluster, "Pump ID  out"=w1780:u16, "Pump COM out"=w1781:refnum<visa-resource-name>)  [unwired: 5 in]
        n1331 = call "Time Delay19"("error in (no error)"=w1767, "Delay Time (s)"=1.0) -> ("error out"=w1768:errorcluster)  [unwired: 9 in]
        n1332 = while {
          tunnel: w1779 -> [w1893]
          tunnel: w1768 -> [w1890]
          tunnel: [w1888] -> w1764
          stop <- w1895 stop-if-true
          n1333 = case shown="\"6\"" w1893 {
            tunnel: [w1897 w1899 w1901 w1903 w1905 w1907 w1909 w1911 w1913 w1915] -> w1892
            tunnel: [w1896 w1898 w1900 w1902 w1904 w1906 w1908 w1910 w1912 w1914] -> w1891
            frame "1", Default {
              n1334 = local read "Phase Sensor Liquid Threshold - Reactor 1"() -> (w1896:dbl)
              n1335 = local read "Phase Sensor Reading - Reactor 1"() -> (w1897:dbl)
            }
            frame "2" {
              n1336 = local read "Phase Sensor Liquid Threshold - Reactor 2"() -> (w1898:dbl)
              n1337 = local read "Phase Sensor Reading - Reactor 2"() -> (w1899:dbl)
            }
            frame "3" {
              n1338 = local read "Phase Sensor Liquid Threshold - Reactor 3"() -> (w1900:dbl)
              n1339 = local read "Phase Sensor Reading - Reactor 3"() -> (w1901:dbl)
            }
            frame "4" {
              n1340 = local read "Phase Sensor Liquid Threshold - Reactor 4"() -> (w1902:dbl)
              n1341 = local read "Phase Sensor Reading - Reactor 4"() -> (w1903:dbl)
            }
            frame "5" {
              n1342 = local read "Phase Sensor Liquid Threshold - Reactor 5"() -> (w1904:dbl)
              n1343 = local read "Phase Sensor Reading - Reactor 5"() -> (w1905:dbl)
            }
            frame "6" {
              n1344 = local read "Phase Sensor Liquid Threshold - Reactor 6"() -> (w1906:dbl)
              n1345 = local read "Phase Sensor Reading - Reactor 6"() -> (w1907:dbl)
            }
            frame "7" {
              n1346 = local read "Phase Sensor Liquid Threshold - Reactor 7"() -> (w1908:dbl)
              n1347 = local read "Phase Sensor Reading - Reactor 7"() -> (w1909:dbl)
            }
            frame "8" {
              n1348 = local read "Phase Sensor Liquid Threshold - Reactor 8"() -> (w1910:dbl)
              n1349 = local read "Phase Sensor Reading - Reactor 8"() -> (w1911:dbl)
            }
            frame "9" {
              n1350 = local read "Phase Sensor Liquid Threshold - Reactor 9"() -> (w1912:dbl)
              n1351 = local read "Phase Sensor Reading - Reactor 9"() -> (w1913:dbl)
            }
            frame "10" {
              n1352 = local read "Phase Sensor Liquid Threshold - Reactor 10"() -> (w1914:dbl)
              n1353 = local read "Phase Sensor Reading - Reactor 10"() -> (w1915:dbl)
            }
          }
          n1354 = Wait (ms)(milliseconds to wait=100) -> ()  [unwired: 1 out]
          n1355 = Greater?(x=w1892, y=w1891) -> (0:w1894:bool)
          n1356 = case shown="False" w1894 {
            tunnel: w1890 -> [w1922 w1927]
            tunnel: [w1917 w1927] -> w1888
            frame False {
              n1357 = local read "Master time [s]"() -> (w1923:dbl)
              n1358 = local read "Carrier Pump ID"() -> (w1919:i32)
              n1359 = local read "Carrier Pump COM"() -> (w1920:refnum<visa-resource-name>)
              n1360 = local write "Phase Sensor Reading Start - Reactor [s]"(w1923) -> ()
              n1361 = call "HARVARD_INFUSE_VOLUME.vi"("error in (no error)"=w1922, "Volume (uL)"=5.0, "Pump ID"=w1919, "Pump COM"=w1920) -> ("error out"=w1918:errorcluster)  [unwired: 5 in, 2 out]
              n1362 = call "Time Delay20"("error in (no error)"=w1918, "Delay Time (s)"=1.0) -> ("error out"=w1917:errorcluster)  [unwired: 9 in]
            }
            frame True {
              n1363 = local read "Phase Sensor - Reactor - Minimum Liquid Length [s]"() -> (w1928:dbl)
              n1364 = local read "Master time [s]"() -> (w1931:dbl)
              n1365 = local read "Phase Sensor Reading Start - Reactor [s]"() -> (w1930:dbl)
              n1366 = local read "Phase Sensor Reading Start - Reactor [s]"() -> (w1925:dbl)
              n1367 = local read "Master time [s]"() -> (w1926:dbl)
              n1368 = Subtract(x=w1931, y=w1930) -> (x-y=w1929:dbl)
              n1369 = Less?(x=w1926, y=w1925) -> (x < y?=w1924:bool)
              n1370 = Greater?(x=w1929, y=w1928) -> (0:w1932:bool)
              n1371 = case shown="True" w1924 {
                frame False {
                }
                frame True {
                  n1372 = local read "Master time [s]"() -> (w1933:dbl)
                  n1373 = local write "Phase Sensor Reading Start - Reactor [s]"(w1933) -> ()
                }
              }
              n1374 = case shown="False" w1932 {
                frame False {
                  n1375 = Wait (ms)(milliseconds to wait=50) -> ()  [unwired: 1 out]
                }
                frame True {
                  n1376 = local write "Phase Sensor Detection - Reactor"(TRUE) -> ()
                }
              }
            }
          }
          n1377 = local read "Phase Sensor Detection - Reactor"() -> (w1895:bool)
        }
        n1378 = local read "Entrance Volume (reactor phase sensor to reactor center) [uL]"() -> (w1789:dbl)
        n1379 = call "Time Delay21"("error in (no error)"=w1764, "Delay Time (s)"=1.0) -> ("error out"=w1763:errorcluster)  [unwired: 9 in]
        n1380 = call "HARVARD_INFUSE_VOLUME.vi"("error in (no error)"=w1763, "Volume (uL)"=w1789, "Pump ID"=w1780, "Pump COM"=w1781) -> ("error out"=w1759:errorcluster, "Pump ID  out"=w1788:u16, "Pump COM out"=w1787:refnum<visa-resource-name>)  [unwired: 5 in]
        n1381 = call "Time Delay24"("error in (no error)"=w1759, "Delay Time (s)"=0.5) -> ("error out"=w1758:errorcluster)  [unwired: 9 in]
        n1382 = call "HARVARD_STOP.vi"("error in (no error)"=w1758, "Pump address (0)"=w1788, "VISA resource name"=w1787) -> ("error out"=w1771:errorcluster)  [unwired: 5 in, 2 out]
        n1383 = call "Time Delay9"("error in (no error)"=w1771, "Delay Time (s)"=4.0) -> ("error out"=w1770:errorcluster)  [unwired: 9 in]
        n1384 = case shown="\"3\"" w1779 {
          tunnel: w1770 -> [w1839 w1844 w1849 w1854 w1859 w1864 w1869 w1874 w1879 w1884]
          tunnel: [w1838 w1843 w1848 w1853 w1858 w1863 w1868 w1873 w1878 w1883] -> w1784
          frame "1", Default {
            n1385 = local read "Reactor Valve 1 Position - Reaction"() -> (w1840:string)
            n1386 = local read "Reactor Valve 1 COM"() -> (w1842:refnum<visa-resource-name>)
            n1387 = local read "Reactor Valve 1 ID"() -> (w1841:i32)
            n1388 = call "VALCO_SET_POS_232.vi"("Error In"=w1839, "New Position (as string)"=w1840, "Valve ID"=w1841, "COM Port In"=w1842) -> ("Error Out"=w1838:errorcluster)  [unwired: 5 in, 2 out]
          }
          frame "2" {
            n1389 = local read "Reactor Valve 2 Position - Reaction"() -> (w1845:string)
            n1390 = local read "Reactor Valve 2 COM"() -> (w1847:refnum<visa-resource-name>)
            n1391 = local read "Reactor Valve 2 ID"() -> (w1846:i32)
            n1392 = call "VALCO_SET_POS_232.vi"("Error In"=w1844, "New Position (as string)"=w1845, "Valve ID"=w1846, "COM Port In"=w1847) -> ("Error Out"=w1843:errorcluster)  [unwired: 5 in, 2 out]
          }
          frame "3" {
            n1393 = local read "Reactor Valve 3 Position - Reaction"() -> (w1850:string)
            n1394 = local read "Reactor Valve 3 COM"() -> (w1852:refnum<visa-resource-name>)
            n1395 = local read "Reactor Valve 3 ID"() -> (w1851:dbl)
            n1396 = call "VALCO_SET_POS_232.vi"("Error In"=w1849, "New Position (as string)"=w1850, "Valve ID"=w1851, "COM Port In"=w1852) -> ("Error Out"=w1848:errorcluster)  [unwired: 5 in, 2 out]
          }
          frame "4" {
            n1397 = local read "Reactor Valve 4 Position - Reaction"() -> (w1855:string)
            n1398 = local read "Reactor Valve 4 COM"() -> (w1857:refnum<visa-resource-name>)
            n1399 = local read "Reactor Valve 4 ID"() -> (w1856:dbl)
            n1400 = call "VALCO_SET_POS_232.vi"("Error In"=w1854, "New Position (as string)"=w1855, "Valve ID"=w1856, "COM Port In"=w1857) -> ("Error Out"=w1853:errorcluster)  [unwired: 5 in, 2 out]
          }
          frame "5" {
            n1401 = local read "Reactor Valve 5 Position - Reaction"() -> (w1860:string)
            n1402 = local read "Reactor Valve 5 COM"() -> (w1862:refnum<visa-resource-name>)
            n1403 = local read "Reactor Valve 5 ID"() -> (w1861:dbl)
            n1404 = call "VALCO_SET_POS_232.vi"("Error In"=w1859, "New Position (as string)"=w1860, "Valve ID"=w1861, "COM Port In"=w1862) -> ("Error Out"=w1858:errorcluster)  [unwired: 5 in, 2 out]
          }
          frame "6" {
            n1405 = local read "Reactor Valve 6 Position - Reaction"() -> (w1865:string)
            n1406 = local read "Reactor Valve 6 COM"() -> (w1867:refnum<visa-resource-name>)
            n1407 = local read "Reactor Valve 6 ID"() -> (w1866:dbl)
            n1408 = call "VALCO_SET_POS_232.vi"("Error In"=w1864, "New Position (as string)"=w1865, "Valve ID"=w1866, "COM Port In"=w1867) -> ("Error Out"=w1863:errorcluster)  [unwired: 5 in, 2 out]
          }
          frame "7" {
            n1409 = local read "Reactor Valve 7 Position - Reaction"() -> (w1870:string)
            n1410 = local read "Reactor Valve 7 COM"() -> (w1872:refnum<visa-resource-name>)
            n1411 = local read "Reactor Valve 7 ID"() -> (w1871:dbl)
            n1412 = call "VALCO_SET_POS_232.vi"("Error In"=w1869, "New Position (as string)"=w1870, "Valve ID"=w1871, "COM Port In"=w1872) -> ("Error Out"=w1868:errorcluster)  [unwired: 5 in, 2 out]
          }
          frame "8" {
            n1413 = local read "Reactor Valve 8 Position - Reaction"() -> (w1875:string)
            n1414 = local read "Reactor Valve 8 COM"() -> (w1877:refnum<visa-resource-name>)
            n1415 = local read "Reactor Valve 8 ID"() -> (w1876:dbl)
            n1416 = call "VALCO_SET_POS_232.vi"("Error In"=w1874, "New Position (as string)"=w1875, "Valve ID"=w1876, "COM Port In"=w1877) -> ("Error Out"=w1873:errorcluster)  [unwired: 5 in, 2 out]
          }
          frame "9" {
            n1417 = local read "Reactor Valve 9 Position - Reaction"() -> (w1882:string)
            n1418 = local read "Reactor Valve 9 COM"() -> (w1880:refnum<visa-resource-name>)
            n1419 = local read "Reactor Valve 9 ID"() -> (w1881:dbl)
            n1420 = call "VALCO_SET_POS_232.vi"("Error In"=w1879, "New Position (as string)"=w1882, "Valve ID"=w1881, "COM Port In"=w1880) -> ("Error Out"=w1878:errorcluster)  [unwired: 5 in, 2 out]
          }
          frame "10" {
            n1421 = local read "Reactor Valve 10 Position - Reaction"() -> (w1885:string)
            n1422 = local read "Reactor Valve 10 COM"() -> (w1887:refnum<visa-resource-name>)
            n1423 = local read "Reactor Valve 10 ID"() -> (w1886:dbl)
            n1424 = call "VALCO_SET_POS_232.vi"("Error In"=w1884, "New Position (as string)"=w1885, "Valve ID"=w1886, "COM Port In"=w1887) -> ("Error Out"=w1883:errorcluster)  [unwired: 5 in, 2 out]
          }
        }
        n1425 = local read "Reaction number - transport to reactor"() -> (w1785:dbl)
        n1426 = script code="loop_to_reactor_last_rxn = loop_to_reactor_last_rxn + 1;"("??"=w1784, "loop_to_reactor_last_rxn"=w1785) -> ("loop_to_reactor_last_rxn"=w1783:dbl)  [unwired: 1 out]
        n1427 = local write "Reaction number - transport to reactor"(w1783) -> ()
      }
    }
    n1428 = Wait (ms)(milliseconds to wait=1000) -> ()  [unwired: 1 out]
    n1429 = local read "Stop everything"() -> (w1719:bool)
  }
  n1430 = while {
    tunnel: w3 -> [w1936]
    stop <- w1938 stop-if-true
    n1431 = local read "Stop everything"() -> (w1939:bool)
    n1432 = Wait (ms)(milliseconds to wait=25) -> ()  [unwired: 1 out]
    n1433 = case shown="True" w1939 {
      tunnel: w1936 -> [_ w1940]
      frame False {
      }
      frame True {
        w1973 = "0"
        w1974 = u16 7001 items=["Read temperature (F)"=4001, "Read setpoint (F)"=8029, "Write setpoint (F)"=7001, "Read autotune status"=8027, "Write start autotune"=8026]
        w1975 = errorcluster {"status"=FALSE, "code"=0, "source"=""} ("error constant")
        w1979 = 0.0
        w1943 = FALSE
        # "TODO:\nUse the \"reactor enabled\"\nbooleans to enable or\ndisable these temperature\nchannel initializations"
        # "Write low temperature setpoints"
        # "Stop cDAQ tasks"
        # "Reset parameters"
        n1434 = local write "Master time [s]"(w1979) -> ()
        n1435 = local write "Reaction number - rinse reactor"(w1979) -> ()
        n1436 = local write "Reaction number - rinse transfer lines"(w1979) -> ()
        n1437 = local write "Reaction number - transport from reactor to analysis"(w1979) -> ()
        n1438 = local write "Reaction number - transport to reactor"(w1979) -> ()
        n1439 = local write "Converged?"(w1943) -> ()
        n1440 = property on="Initiate hardware communication" class="Bool (strict)"(error in=w1975, "DisabledEnum"=T8."Disabled and Grayed Out") -> ()  [unwired: 1 in, 2 out]
        n1441 = property on="Pressurization confirmed" class="Bool (strict)"(error in=w1975, "DisabledEnum"=T8."Disabled and Grayed Out") -> ()  [unwired: 1 in, 2 out]
        n1442 = local write "Initiate hardware communication"(w1943) -> ()
        n1443 = local write "Pressurization confirmed"(w1943) -> ()
        n1444 = local write "Hardware communication established"(w1943) -> ()
        n1445 = local write "Ready to start schedule timer"(w1943) -> ()
        n1446 = local write "Phase Sensor Detection - Injection Valve"(w1943) -> ()
        n1447 = local write "Stop everything"(w1943) -> ()
        n1448 = local write "Phase Sensor Detection - Reactor"(w1943) -> ()
        n1449 = local write "Phase Sensor Detection - Analytical Valve"(w1943) -> ()
        n1450 = local read "Analog Input (NI 9205) task out"() -> (w1976:refnum<k21>)
        n1451 = local read "Vent Valve Position - Vent"() -> (w1951:string)
        n1452 = local read "Vent Valve COM"() -> (w1949:refnum<visa-resource-name>)
        n1453 = local read "Vent Valve ID"() -> (w1950:i32)
        n1454 = call "STOP_CDAQ_NIMAX_NSE_Parallel.vi"("Analog input DAQmx Task"=w1976, "Error In"=w1975) -> ("error out"=w1944:errorcluster)  [unwired: 13 in]
        n1455 = local read "Watlow Zone - Reactor 2"() -> (w1955:dbl)
        n1456 = local read "Watlow Instance - Reactor 2"() -> (w1956:dbl)
        n1457 = local read "Watlow Zone - Reactor 3"() -> (w1957:dbl)
        n1458 = local read "Watlow Instance - Reactor 3"() -> (w1958:dbl)
        n1459 = local read "Watlow Zone - Reactor 4"() -> (w1959:dbl)
        n1460 = local read "Watlow Instance - Reactor 4"() -> (w1960:dbl)
        n1461 = local read "Watlow Zone - Reactor 5"() -> (w1961:dbl)
        n1462 = local read "Watlow Instance - Reactor 5"() -> (w1962:dbl)
        n1463 = local read "Watlow Zone - Reactor 6"() -> (w1963:dbl)
        n1464 = local read "Watlow Instance - Reactor 6"() -> (w1964:dbl)
        n1465 = local read "Watlow Zone - Reactor 7"() -> (w1965:dbl)
        n1466 = local read "Watlow Instance - Reactor 7"() -> (w1966:dbl)
        n1467 = local read "Watlow Zone - Reactor 8"() -> (w1967:dbl)
        n1468 = local read "Watlow Instance - Reactor 8"() -> (w1968:dbl)
        n1469 = local read "Watlow Zone - Reactor 9"() -> (w1970:dbl)
        n1470 = local read "Watlow Instance - Reactor 9"() -> (w1969:dbl)
        n1471 = local read "Watlow Zone - Reactor 10"() -> (w1971:dbl)
        n1472 = local read "Watlow Instance - Reactor 10"() -> (w1972:dbl)
        n1473 = local read "Watlow Instance - Reactor 1"() -> (w1954:dbl)
        n1474 = local read "Watlow Zone - Reactor 1"() -> (w1953:dbl)
        n1475 = local read "Watlow COM"() -> (w1952:refnum<visa-resource-name>)
        n1476 = call "Write.vi"("PC Comms Port"=w1952, "Zone"=w1953, "Parameter"=w1974, "Instance"=w1954, "Write Value"=w1973, "Error In"=w1944) -> ()  [unwired: 13 in, 1 out]
        n1477 = call "Write.vi"("PC Comms Port"=w1952, "Zone"=w1955, "Parameter"=w1974, "Instance"=w1956, "Write Value"=w1973, "Error In"=w1944) -> ()  [unwired: 13 in, 1 out]
        n1478 = call "Write.vi"("PC Comms Port"=w1952, "Zone"=w1957, "Parameter"=w1974, "Instance"=w1958, "Write Value"=w1973, "Error In"=w1944) -> ()  [unwired: 13 in, 1 out]
        n1479 = call "Write.vi"("PC Comms Port"=w1952, "Zone"=w1959, "Parameter"=w1974, "Instance"=w1960, "Write Value"=w1973, "Error In"=w1944) -> ()  [unwired: 13 in, 1 out]
        n1480 = call "Write.vi"("PC Comms Port"=w1952, "Zone"=w1961, "Parameter"=w1974, "Instance"=w1962, "Write Value"=w1973, "Error In"=w1944) -> ()  [unwired: 13 in, 1 out]
        n1481 = call "Write.vi"("PC Comms Port"=w1952, "Zone"=w1963, "Parameter"=w1974, "Instance"=w1964, "Write Value"=w1973, "Error In"=w1944) -> ()  [unwired: 13 in, 1 out]
        n1482 = call "Write.vi"("PC Comms Port"=w1952, "Zone"=w1965, "Parameter"=w1974, "Instance"=w1966, "Write Value"=w1973, "Error In"=w1944) -> ()  [unwired: 13 in, 1 out]
        n1483 = call "Write.vi"("PC Comms Port"=w1952, "Zone"=w1967, "Parameter"=w1974, "Instance"=w1968, "Write Value"=w1973, "Error In"=w1944) -> ()  [unwired: 13 in, 1 out]
        n1484 = call "Write.vi"("PC Comms Port"=w1952, "Zone"=w1970, "Parameter"=w1974, "Instance"=w1969, "Write Value"=w1973, "Error In"=w1944) -> ()  [unwired: 13 in, 1 out]
        n1485 = call "Write.vi"("PC Comms Port"=w1952, "Zone"=w1971, "Parameter"=w1974, "Instance"=w1972, "Write Value"=w1973, "Error In"=w1944) -> ("Error Out"=w1941:errorcluster)  [unwired: 13 in]
        n1486 = call "VALCO_SET_POS_232.vi"("Error In"=w1941, "New Position (as string)"=w1951, "Valve ID"=w1950, "COM Port In"=w1949) -> ("Error Out"=w1947:errorcluster)  [unwired: 5 in, 2 out]
        n1487 = call "Display Message to User3"("error in (no error)"=w1947, "Message"="The vent valve is open, but only the selector valves' current reactor channel is depressurized. The other channel lines remain pressurized. Proceed with caution.") -> ("error out"=w1945:errorcluster)  [unwired: 8 in, 1 out]
        n1488 = case shown="True" TRUE {
          selector: TRUE -> [_ w1982]
          tunnel: w1945 -> [_ w1980]
          frame False {
          }
          frame True {
            n1489 = local write "Shutdown complete"(w1982) -> ()
            n1490 = call "Time Delay7"("error in (no error)"=w1980, "Delay Time (s)"=1.0) -> ()  [unwired: 9 in, 1 out]
            n1491 = Stop(stop? (T)=w1982) -> ()
          }
        }
        n1492 = Close Python Session(session in=w1940, error in=w1941) -> (11:→"error out":errorcluster)
      }
    }
    n1493 = local read "Shutdown complete"() -> (w1938:bool)
  }
  n1494 = call "Time Delay45"("error in (no error)"=errorcluster {"status"=FALSE, "code"=0, "source"=""} ("error constant"), "Delay Time (s)"=600.0) -> ("error out"=w2:errorcluster)  [unwired: 9 in]
  n1495 = while {
    shift-right: [w1983] -> _
    shift-left: Liquid_Handler_Enum_NSE."Waiting for hardware initialization" ("Enum") -> [w1984]
    stop <- w1985 stop-if-true
    n1496 = case shown="\"Liquid handler is preparing a droplet\"" w1984 {
      tunnel: [w1986 w2000 Liquid_Handler_Enum_NSE."Liquid handler is idle" ("Enum")] -> w1983
      frame "Waiting for hardware initialization" {
        n1497 = while {
          tunnel: [w1987] -> w1986
          stop <- w1988 stop-if-true
          n1498 = local read "Ready to start schedule timer"() -> (w1990:bool)
          n1499 = call "Elapsed Time2"("Time Target (s)"=1.0) -> ("Time has Elapsed"=w1988:bool)  [unwired: 11 in, 7 out]
          n1500 = case shown="False" w1990 {
            tunnel: [Liquid_Handler_Enum_NSE."Waiting for hardware initialization" ("Enum") Liquid_Handler_Enum_NSE."Liquid handler is preparing a droplet" ("Enum")] -> w1987
            frame False {
            }
            frame True {
              # "Once the hardware initialization is complete, the main timer will start,\nand the liquid handler can begin preparing its first droplet"
            }
          }
        }
      }
      frame "Liquid handler is idle" {
        # "Start preparing the next droplet in the list\nif the next start time specified in the schedule\nis less than the master time AND we know that\nthe liquid handler's schedule is not finished."
        n1501 = local read "liquid_handler_finished"() -> (w1995:bool)
        n1502 = local read "Next start time - liquid handler"() -> (w1998:dbl)
        n1503 = local read "Master time [s]"() -> (w1997:dbl)
        n1504 = Less Or Equal?(x=w1998, y=w1997) -> (x <= y?=w1996:bool)
        n1505 = Not(x=w1995) -> (.not. x?=w1994:bool)
        n1506 = And(x=w1996, y=w1994) -> (x .and. y?=w1993:bool)
        n1507 = case shown="True" w1993 {
          tunnel: [Liquid_Handler_Enum_NSE."Liquid handler is idle" ("Enum") Liquid_Handler_Enum_NSE."Liquid handler is preparing a droplet" ("Enum")] -> w2000
          frame False {
            n1508 = Wait (ms)(milliseconds to wait=1000) -> ()  [unwired: 1 out]
          }
          frame True {
          }
        }
        n1509 = local write "Phase Sensor Reading Start - Injection Valve [s]"(1000000000000000.0) -> ()
      }
      frame "Liquid handler is preparing a droplet" {
        w2016 = 280.0
        # "Get rid of air bubbles that might appear while stirring"
        # "Small delay to make sure\ncarrier has time to get the\nprevious droplet out of the\nsample loop"
        # "Check for droplet at injection valve sample loop using phase sensor"
        # "Get the droplet most of the way there,\nthen keep withdrawing until the phase\nsensor confirms that the droplet is in\nthe injection sample loop"
        # "The injection valve phase sensor should be detecting liquid most of the time.\nWhen the reading is below the liquid threshold, we know there's gas at the\nsensor, which means the droplet is in the sample loop (until it gets injected)"
        # "Update slug tracker to identify injected slug\nGet next start time for the liquid handler"
        # "Withdraw droplet into injection valve's sample loop"
        # "Infuse at least ~300uL\nto get the transfer fluid\nback past the sample loop"
        n1510 = local read "Injection Valve Position - LH Needle"() -> (w2044:string)
        n1511 = local read "Gilson COM"() -> (w2042:refnum<visa-resource-name>)
        n1512 = local read "Gilson LH ID"() -> (w2043:i32)
        n1513 = local read "Injection Valve ID"() -> (w2045:i32)
        n1514 = local read "LH Pump COM"() -> (w2115:refnum<visa-resource-name>)
        n1515 = local read "Gilson COM"() -> (w2111:refnum<visa-resource-name>)
        n1516 = local read "Injection Valve COM"() -> (w2046:refnum<visa-resource-name>)
        n1517 = call "Time Delay2"("error in (no error)"=errorcluster {"status"=FALSE, "code"=0, "source"=""} ("error constant"), "Delay Time (s)"=25) -> ("error out"=w2040:errorcluster)  [unwired: 9 in]
        n1518 = local read "Gilson Valve ID"() -> (w2112:i32)
        n1519 = call "Gilson Home Device.vi"("error in"=w2040, "ID (30 for GX-241)"=w2043, "VISA resource name"=w2042) -> ("error out"=w2041:errorcluster)  [unwired: 6 in, 2 out]
        n1520 = call "VALCO_SET_POS_232.vi"("Error In"=w2041, "New Position (as string)"=w2044, "Valve ID"=w2045, "COM Port In"=w2046) -> ("Error Out"=w2047:errorcluster)  [unwired: 5 in, 2 out]
        n1521 = local read "LH Pump ID"() -> (w2116:i32)
        n1522 = call "Gilson DI Switch to Inject.vi"("error in"=w2047, "ID"=w2112, "VISA resource name"=w2111) -> ("error out"=w2113:errorcluster)  [unwired: 6 in, 2 out]
        n1523 = local read "LH Transfer Fluid Density (g/L)"() -> (w2089:dbl)
        n1524 = local read "LH Sample Loop Volume (uL)"() -> (w2088:dbl)
        n1525 = call "Gilson Dispense Sample - Harvard.vi"("Outlet and LH Pump ID"=w2116, "Volume to Dispense (uL)"=430.0, "Outlet and LH Pump COM"=w2115, "error in"=w2113, "Dispense Speed (uL/min)"=3000.0) -> ("Pump ID Out"=w2117:u8, "error out"=w2114:errorcluster)  [unwired: 11 in, 2 out]
        n1526 = local read "LH Valve Position - Needle"() -> (w2101:string)
        n1527 = local read "LH Valve Position - Reservoir"() -> (w2100:string)
        n1528 = local read "LH Valve COM"() -> (w2110:refnum<visa-resource-name>)
        n1529 = local read "Number of LH Needle Purges Prior to Droplet Prep"() -> (w2098:dbl)
        n1530 = script code="invalid_concs = 0;\n\n[prep_slug,comp,all_slugs] = nse_get_next_slug_to_prep_v5(all_slugs,reagent_table,inj_vol,rho_tf);\n\nif ~isempty(comp)\n    invalid_concs = double(any(comp(1,:) < 0))\n    if invalid_concs\n        all_slugs(prep_slug).complete = -1;\n        temp_num = all_slugs(prep_slug).number;\n        all_slugs(prep_slug).in_prep = 0;\n        prep_slug = 0;\n        prep_flag = ['Slug ' num2str(temp_num) ' has an invalid composition!'];\n    else\n        prep_flag = ['Preparing slug ' num2str(all_slugs(prep_slug).number)];\n    end\nend\nabort_prep = 0;"("??"=w2040, "inj_vol"=w2088, "rho_tf"=w2089) -> ("??"=w2039:errorcluster, "prep_flag"=w2085:string)
        "Slug Composition Error" <- w2039
        n1531 = call "Gilson Home Pump and Flush - Harvard.vi"("Outlet and LH Pump COM"=w2115, "Pump ID"=w2117, "Numer of primes"=w2098, "Volume (uL)"=600.0, "Flow rate (uL/min)"=1000.0, "error in"=w2114, "LH Valve COM"=w2110, "LH Valve Position - Reservoir"=w2100, "LH Valve Position - Needle"=w2101) -> ("error out"=w2099:errorcluster)  [unwired: 8 in, 2 out]
        n1532 = call "Time Delay3"("error in (no error)"=w2099, "Delay Time (s)"=2.5) -> ("error out"=w2097:errorcluster)  [unwired: 9 in]
        n1533 = local read "Gilson COM"() -> (w2102:refnum<visa-resource-name>)
        n1534 = local read "Gilson LH ID"() -> (w2096:i32)
        n1535 = call "Gilson Lift Probe.vi"("error in"=w2097, "Handler ID"=w2096, "VISA resource name"=w2102) -> ("error out"=w2108:errorcluster)  [unwired: 6 in, 2 out]
        n1536 = local read "Dip Time of LH Needle in Rinse Vial [s]"() -> (w2103:dbl)
        n1537 = local read "Rinse Well Number"() -> (w2109:i16)
        n1538 = local read "Rinse Rack Placement"() -> (w2104:i16)
        n1539 = local read "Rinse Rack Number"() -> (w2105:i16)
        n1540 = local read "Gilson LH ID"() -> (w2106:i32)
        n1541 = local read "Gilson COM"() -> (w2107:refnum<visa-resource-name>)
        n1542 = call "Gilson Dip Needle.vi"("VISA resource name"=w2107, "Handler ID"=w2106, "Number of Dips"=2, "error in"=w2108, "(Rinse) Rack Number"=w2105, "(Rinse) Rack Placement"=w2104, "(Rinse) Well Number"=w2109, "Dip Time (s)"=w2103) -> ("error out"=w2057:errorcluster)  [unwired: 17 in, 2 out]
        n1543 = Unbundle By Name(w2039) -> ("status"=w2087:bool, "source"=w2086:string)  [unwired: 1 out]
        n1544 = local write "Slug Composition Error"(w2039) -> ()
        n1545 = Select(t=w2086, s=w2087, f=w2085) -> (s? t:f=w2084:string)
        n1546 = local write "Slug preparation status"(w2084) -> ()
        n1547 = script code="MATLAB script"("??"=w2039) -> ("comp"=w2073:dbl[][])  [unwired: 1 out]
        n1548 = local read "Gas Buffer Well Number"() -> (w2083:i16)
        n1549 = local read "Gas Buffer Rack Placement"() -> (w2082:i16)
        n1550 = local read "Gas Buffer Rack Number"() -> (w2081:i16)
        n1551 = local read "Rinse Well Number"() -> (w2080:i16)
        n1552 = local read "Rinse Rack Placement"() -> (w2079:i16)
        n1553 = local read "Rinse Rack Number"() -> (w2078:i16)
        n1554 = local read "Gilson COM"() -> (w2077:refnum<visa-resource-name>)
        n1555 = local read "Gilson LH ID"() -> (w2076:i32)
        n1556 = local read "LH Pump ID"() -> (w2075:i32)
        n1557 = local read "Perfluorinated Oil Well Number"() -> (w2053:dbl)
        n1558 = local read "LH Withdraw\nFlow Rate (uL/min)"() -> (w2074:dbl)
        n1559 = local read "LH Injection Flow Rate (uL/min)"() -> (w2071:dbl)
        n1560 = local read "LH Buffer (upstream) [uL]"() -> (w2072:dbl)
        n1561 = local read "Number of Rinse Vial Dips of the LH Needle, Between Stock Solutions"() -> (w2070:i32)
        n1562 = local read "Dip Time of LH Needle in Rinse Vial [s]"() -> (w2069:dbl)
        n1563 = local read "Number of Droplet Stirs"() -> (w2068:i32)
        n1564 = local read "LH Gas Buffer (downstream) [uL]"() -> (w2063:dbl)
        n1565 = local read "LH Valve COM"() -> (w2064:refnum<visa-resource-name>)
        n1566 = local read "LH Valve Position - Needle"() -> (w2065:string)
        n1567 = local read "LH Pump COM"() -> (w2067:refnum<visa-resource-name>)
        n1568 = local read "LH Valve ID"() -> (w2066:i32)
        n1569 = call "Gilson Load into Needle Full - Harvard.vi"("Gilson COM"=w2077, "Handler ID"=w2076, "Pump ID"=w2075, "Slug Composition"=w2073, "Withdraw Flow Rate (uL/min)"=w2074, "Injection Flow Rate (uL/min)"=w2071, "Oil Well Number"=w2053, "Error In"=w2057, "(Rinse) Rack Number"=w2078, "Buffer (uL)"=w2072, "(Rinse) Rack Placement"=w2079, "Number of Dips"=w2070, "(Rinse) Well Number"=w2080, "Dip Time (s)"=w2069, "Gas Rack Number"=w2081, "Number of Stirs"=w2068, "Gas Rack Placement"=w2082, "Gas Well Number"=w2083, "LH Valve COM"=w2064, "LH Pump COM"=w2067, "LH Valve ID"=w2066, "LH Valve Position - Needle"=w2065, "Post-droplet gas buffer [uL]"=w2063) -> ("Prep Error Out"=w2025:errorcluster)  [unwired: 3 in, 1 out]
        n1570 = local read "LH Valve Position - Reservoir"() -> (w2028:string)
        n1571 = local read "LH Valve ID"() -> (w2027:i32)
        n1572 = local read "LH Valve COM"() -> (w2026:refnum<visa-resource-name>)
        n1573 = local read "LH Pump COM"() -> (w2019:refnum<visa-resource-name>)
        n1574 = local read "LH Pump ID"() -> (w2018:i32)
        n1575 = call "HARVARD_WITHDRAW_VOLUME.vi"("error in (no error)"=w2025, "Volume (uL)"=100.0, "Pump ID"=w2018, "Pump COM"=w2019) -> ("error out"=w2022:errorcluster)  [unwired: 5 in, 2 out]
        n1576 = call "Time Delay43"("error in (no error)"=w2022, "Delay Time (s)"=2.0) -> ("error out"=w2021:errorcluster)  [unwired: 9 in]
        n1577 = call "VALCO_SET_POS_232.vi"("Error In"=w2021, "New Position (as string)"=w2028, "Valve ID"=w2027, "COM Port In"=w2026) -> ("Error Out"=w2020:errorcluster)  [unwired: 5 in, 2 out]
        n1578 = call "HARVARD_INFUSE_VOLUME.vi"("error in (no error)"=w2020, "Volume (uL)"=w2016, "Pump ID"=w2018, "Pump COM"=w2019) -> ("error out"=w2017:errorcluster, "Pump ID  out"=w2015:u16, "Pump COM out"=w2014:refnum<visa-resource-name>)  [unwired: 5 in]
        n1579 = call "HARVARD_WITHDRAW_VOLUME.vi"("error in (no error)"=w2017, "Volume (uL)"=w2016, "Pump ID"=w2015, "Pump COM"=w2014) -> ("error out"=w2012:errorcluster)  [unwired: 5 in, 2 out]
        n1580 = call "Time Delay80"("error in (no error)"=w2012, "Delay Time (s)"=2.0) -> ("error out"=w2008:errorcluster)  [unwired: 9 in]
        n1581 = local read "LH Valve Position - Needle"() -> (w2009:string)
        n1582 = local read "Transfer Volume from Needle to Sample Loop [uL]"() -> (w2006:dbl)
        n1583 = local read "LH Valve ID"() -> (w2010:i32)
        n1584 = local read "LH Valve COM"() -> (w2011:refnum<visa-resource-name>)
        n1585 = call "VALCO_SET_POS_232.vi"("Error In"=w2008, "New Position (as string)"=w2009, "Valve ID"=w2010, "COM Port In"=w2011) -> ("Error Out"=w2007:errorcluster)  [unwired: 5 in, 2 out]
        n1586 = call "HARVARD_SETFLOWRATE_WITHDRAW.vi"("VISA resource name"=w2019, "Pump address (0)"=w2018, "Withdraw Flow Rate (80)"=500.0, "error in (no error)"=w2007) -> ("VISA resource name out"=w2061:refnum<visa-resource-name>, "Pump address  out"=w2062:u16, "error out"=w2034:errorcluster)  [unwired: 9 in]
        n1587 = call "Time Delay18"("error in (no error)"=w2034, "Delay Time (s)"=1.0) -> ("error out"=w2033:errorcluster)  [unwired: 9 in]
        n1588 = Subtract(x=w2006, y=100.0) -> (x-y=w2005:dbl)
        n1589 = call "HARVARD_WITHDRAW_VOLUME.vi"("error in (no error)"=w2033, "Volume (uL)"=w2005, "Pump ID"=w2062, "Pump COM"=w2061) -> ("error out"=w2050:errorcluster, "Pump ID  out"=w2051:u16, "Pump COM out"=w2052:refnum<visa-resource-name>)  [unwired: 5 in]
        n1590 = while {
          tunnel: w2050 -> [w2119]
          tunnel: [w2118] -> w2030
          stop <- w2121 stop-if-true
          n1591 = local read "Phase Sensor Reading - Injection Valve [V]"() -> (w2124:dbl)
          n1592 = local read "Phase Sensor Liquid Threshold - Injection Valve"() -> (w2123:dbl)
          n1593 = call "Time Delay30"("error in (no error)"=w2119, "Delay Time (s)"=0.5) -> ("error out"=w2118:errorcluster)  [unwired: 9 in]
          n1594 = Less?(x=w2124, y=w2123) -> (x < y?=w2122:bool)
          n1595 = case shown="True" w2122 {
            tunnel: w2118 -> [w2128 w2133]
            frame False {
              n1596 = local read "LH Pump COM"() -> (w2126:refnum<visa-resource-name>)
              n1597 = local read "LH Pump ID"() -> (w2127:i32)
              n1598 = call "HARVARD_WITHDRAW_VOLUME.vi"("error in (no error)"=w2128, "Volume (uL)"=5.0, "Pump ID"=w2127, "Pump COM"=w2126) -> ()  [unwired: 5 in, 3 out]
              n1599 = local read "Master time [s]"() -> (w2129:dbl)
              n1600 = local write "Phase Sensor Reading Start - Injection Valve [s]"(w2129) -> ()
            }
            frame True {
              n1601 = local read "LH Pump COM"() -> (w2135:refnum<visa-resource-name>)
              n1602 = local read "LH Pump ID"() -> (w2136:i32)
              n1603 = local read "Phase Sensor Reading Start - Injection Valve [s]"() -> (w2131:dbl)
              n1604 = local read "Master time [s]"() -> (w2130:dbl)
              n1605 = call "HARVARD_WITHDRAW_VOLUME.vi"("error in (no error)"=w2133, "Volume (uL)"=2.0, "Pump ID"=w2136, "Pump COM"=w2135) -> ()  [unwired: 5 in, 3 out]
              n1606 = local read "Phase Sensor - Injection Valve - Minimum Gas Length [s]"() -> (w2139:dbl)
              n1607 = local read "Phase Sensor Reading Start - Injection Valve [s]"() -> (w2140:dbl)
              n1608 = local read "Master time [s]"() -> (w2141:dbl)
              n1609 = Less?(x=w2130, y=w2131) -> (x < y?=w2132:bool)
              n1610 = case shown="True" w2132 {
                frame False {
                }
                frame True {
                  n1611 = local read "Master time [s]"() -> (w2142:dbl)
                  n1612 = local write "Phase Sensor Reading Start - Injection Valve [s]"(w2142) -> ()
                }
              }
              n1613 = Subtract(x=w2141, y=w2140) -> (x-y=w2138:dbl)
              n1614 = Greater Or Equal?(x=w2138, y=w2139) -> (x >= y?=w2137:bool)
              n1615 = case shown="False" w2137 {
                frame False {
                  n1616 = Wait (ms)(milliseconds to wait=200) -> ()  [unwired: 1 out]
                }
                frame True {
                  n1617 = local write "Phase Sensor Detection - Injection Valve"(TRUE) -> ()
                }
              }
            }
          }
          n1618 = local read "Phase Sensor Detection - Injection Valve"() -> (w2121:bool)
        }
        n1619 = call "Time Delay22"("error in (no error)"=w2030, "Delay Time (s)"=0.5) -> ("error out"=w2029:errorcluster)  [unwired: 9 in]
        n1620 = call "HARVARD_STOP.vi"("error in (no error)"=w2029, "Pump address (0)"=w2051, "VISA resource name"=w2052) -> ("error out"=w2054:errorcluster)  [unwired: 5 in, 2 out]
        n1621 = local read "Schedule - Liquid Handler"() -> (w2056:dbl[])
        n1622 = local read "LH Sample Loop Volume (uL)"() -> (w2058:dbl)
        n1623 = script code="% Update status of slug to injected into system\n[all_slugs] = cwc_mark_slug_injected_v2(all_slugs,prep_slug,load_vol);\n\n% Prepare quench injection\nquench_inj_vol = cwc_get_quench_inj_vol(all_slugs, prep_slug);\n% Base is prepared inside reactor control loop\ninjected = 1;\n\nliquid_handler_finished = 0;\nnext_slug = prep_slug + 1; % slug ID of next reaction\nif next_slug <= numel(liquid_handler_start_times)\n    liquid_handler_next_start_time = liquid_handler_start_times(next_slug);\nelse\n    liquid_handler_finished = 1;\nend"("??"=w2054, "load_vol"=w2058, "liquid_handler_start_times"=w2056) -> ("??"=w2038:errorcluster, "liquid_handler_next_start_time"=w2055:dbl, "liquid_handler_finished"=w2036:dbl)
        "Slug Preparation Error" <- w2038
        n1624 = Not Equal To 0?(x=w2036) -> (x != 0?=w2035:bool)
        n1625 = local write "liquid_handler_finished"(w2035) -> ()
        n1626 = local write "Next start time - liquid handler"(w2055) -> ()
        n1627 = Unbundle By Name(w2038) -> ("status"=w2037:bool)
        n1628 = local write "Slug preparation error"(w2037) -> ()
      }
    }
    n1629 = local read "Stop everything"() -> (w1985:bool)
  }
  n1630 = in-place {
    in-place-border: [w2147] -> w1
    in-place-border: w2 -> [w2147]
    n1631 = local read "Index_Ana_Rxn"() -> (w2145:dbl)
    n1632 = local read "Next analysis time"() -> (w2146:dbl)
    n1633 = local write "NextAnaTimeTrigger"(w2146) -> ()
    n1634 = local write "IndexAct"(w2145) -> ()
  }
  n1635 = while {
    shift-right: [w2148] -> _
    shift-left: w1 -> [w2165]
    shift-right: [w2159] -> _
    shift-left: w3 -> [w2160]
    stop <- w2171 stop-if-true
    n1636 = local read "Analytical method length [s]"() -> (w2156:dbl)
    n1637 = local read "Analysis Error"() -> (w2166:errorcluster)
    n1638 = local read "Transport time - reactor to analysis [s]"() -> (w2151:dbl)
    n1639 = local read "Master time [s]"() -> (w2158:dbl)
    n1640 = local read "NextAnaTimeTrigger"() -> (w2154:dbl)
    n1641 = local read "analysis_finished"() -> (w2164:bool)
    n1642 = local read "Converged?"() -> (w2162:bool)
    n1643 = local read "analysis_finished"() -> (w2170:bool)
    n1644 = local read "Path for HPLC Chromatograms"() -> (w2172:string)
    n1645 = Merge Errors(w2166, w2165) -> (w2150:errorcluster)
    n1646 = Add(x=30.0, y=w2156) -> (x+y=w2155:dbl)
    n1647 = Not(x=w2162) -> (.not. x?=w2161:bool)
    n1648 = Add(x=w2155, y=w2158) -> (x+y=w2153:dbl)
    n1649 = Not(x=w2170) -> (.not. x?=w2168:bool)
    n1650 = And(x=w2161, y=w2164) -> (x .and. y?=w2163:bool)
    n1651 = Subtract(x=w2153, y=w2151) -> (x-y=w2152:dbl)
    n1652 = Greater?(x=w2152, y=w2154) -> (0:w2169:bool)
    n1653 = And(x=w2169, y=w2168) -> (x .and. y?=w2167:bool)
    n1654 = case shown="True" w2167 {
      tunnel: w2172 -> [_ w2251]
      tunnel: w2150 -> [w2223 w2228]
      tunnel: [w2222 w2225] -> w2149
      frame False {
        n1655 = call "Time Delay42"("error in (no error)"=w2223, "Delay Time (s)"=5.0) -> ("error out"=w2222:errorcluster)  [unwired: 9 in]
      }
      frame True {
        # "Find File Alphabetically"
        # "Find Folders in Directoy"
        n1656 = String To Path(string=w2251) -> (path=w2250:path)
        n1657 = List Folder(path=w2250, pattern="Data pattern", error in=w2228) -> (folder names=w2249:string[], error out=w2229:errorcluster)  [unwired: 1 in, 2 out]
        n1658 = in-place {
          in-place-border: w2229 -> [w2263]
          in-place-border: [w2263] -> w2230
          n1659 = local read "reactor_to_analysis_finished"() -> (w2260:bool)
          n1660 = case shown="False" w2260 {
            frame False {
              n1661 = local write "analysis_finished"(FALSE) -> ()
            }
            frame True {
              n1662 = local write "analysis_finished"(TRUE) -> ()
            }
          }
          n1663 = local read "Next analysis time"() -> (w2262:dbl)
          n1664 = local read "Index_Ana_Rxn"() -> (w2261:dbl)
          n1665 = local write "NextAnaTimeTrigger"(w2262) -> ()
          n1666 = local write "IndexTemp"(w2261) -> ()
        }
        n1667 = local read "Analytical method length [s]"() -> (w2227:dbl)
        n1668 = Array Size(array=w2249) -> (size(s)=w2253:i32)
        n1669 = call "Time Delay81"("error in (no error)"=w2230, "Delay Time (s)"=w2227) -> ("error out"=w2232:errorcluster)  [unwired: 9 in]
        n1670 = Subtract(x=w2253, y=1.0) -> (x-y=w2257:dbl)
        n1671 = Split 1D Array(array=w2249, index=w2257) -> (second subarray=w2256:string[])  [unwired: 1 out]
        n1672 = local read "Number of initial experiments"() -> (w2233:i32)
        n1673 = Array of Strings to Path(0:w2256, 1:TRUE ("relative")) -> (2:w2254:path)
        n1674 = local read "IndexAct"() -> (w2231:dbl)
        n1675 = local read "Batch size"() -> (w2234:i32)
        n1676 = local read "Data Analysis File (root)"() -> (w2246:string)
        n1677 = Build Path(base path=w2250, name or relative path=w2254) -> (appended path=w2243:path)
        n1678 = Path To String(path=w2243) -> (string=w2247:string)
        n1679 = local read "Name of HPLC processing function"() -> (w2244:string)
        n1680 = local read "Full Results"() -> (w2238:dbl[])
        n1681 = local read "Batch Results"() -> (w2237:dbl[])
        n1682 = script code="reprocessing = 0;\noptimization_on = 0;\nconverged = 0;\n\n[all_slugs,product_area,data_processing_exit_flag] = feval(process_fun,data_path,ana_path,all_slugs,analyte_table,1,optimization_on,reprocessing);\n\nif ~isempty(full_results)\n  current_opt = max(full_results);\nend\n\nif  isempty(full_results)\n  current_opt = 0;\nend\n\nif iteration == 0\n   IndexAdd = 0;\nelse\n   IndexAdd = N_InExp+(iteration-1)*Batch_size;\nend\n\nbatch_results(Index_Ana_Rxn) = product_area;\nIndex_fullRes = IndexAdd + Index_Ana_Rxn;\nfull_results(Index_fullRes) = product_area;\n\n%full_results = [full_results,product_area];\n%batch_results = [batch_results,product_area];\n\n\nif analysis_finished % check for convergence\nif max(batch_results) < (current_opt + convergence_criterion)\n        converged = 1;\nend\nend"("??"=w2232, "data_path"=w2247, "ana_path"=w2246, "process_fun"=w2244, "convergence_criterion"="Convergence criterion (area counts)", "full_results"=w2238, "batch_results"=w2237, "Index_Ana_Rxn"=w2231, "Batch_size"=w2234, "N_InExp"=w2233) -> ("??"=w2226:errorcluster, "data_processing_exit_flag"=→"Data processing output":string, "converged"=w2240:dbl, "product_area"=→"Product area":dbl, "full_results"=w2236:dbl[], "batch_results"=w2235:dbl[])
        n1683 = Not Equal To 0?(x=w2240) -> (x != 0?=→"Converged?":bool)
        n1684 = local write "Full Results"(w2236) -> ()
        n1685 = local write "Batch Results"(w2235) -> ()
        n1686 = in-place {
          in-place-border: w2226 -> [w2258]
          in-place-border: [w2258] -> w2225
          n1687 = local read "IndexTemp"() -> (w2259:dbl)
          n1688 = local write "IndexAct"(w2259) -> ()
        }
      }
    }
    n1689 = case shown="True" w2163 {
      tunnel: w2160 -> [w2174 w2177]
      tunnel: [w2174 w2177] -> w2159
      frame False {
        n1690 = Wait (ms)(milliseconds to wait=10000) -> ()  [unwired: 1 out]
      }
      frame True {
        w2200 = 0.0
        n1691 = local read "Batch size"() -> (w2186:i32)
        n1692 = local read "Batch Results"() -> (w2189:dbl[])
        n1693 = local read "Array"() -> (w2191:dbl[][])
        n1694 = local read "InitializationExp"() -> (w2185:bool)
        n1695 = local read "Next batch"() -> (w2193:dbl[][])
        n1696 = call "Time Delay82"("error in (no error)"=errorcluster {"status"=FALSE, "code"=0, "source"=""} ("error constant"), "Delay Time (s)"=120.0) -> ("error out"=w2183:errorcluster)  [unwired: 9 in]
        n1697 = local read "Refinement function"() -> (w2192:string)
        n1698 = case shown="True" w2185 {
          tunnel: w2186 -> [w2213 _]
          tunnel: [w2213 w2214] -> w2187
          frame False {
          }
          frame True {
            n1699 = local read "Number of initial experiments"() -> (w2214:i32)
          }
        }
        n1700 = Reshape Array(w2189, 1, w2187) -> (w2188:dbl[][])
        n1701 = local read "Dragonfly python path"() -> (w2194:path)
        n1702 = node(w2177, w2194, w2192, w2183, w2191, w2193, w2188, w2187, w2186) -> (w2176:errorcluster, w2181:dbl[][])  [unwired: 4 in, 3 out]
        n1703 = local write "Next batch"(w2181) -> ()
        n1704 = local read "Master time [s]"() -> (w2212:dbl)
        n1705 = script code="iteration = iteration + 1;\nreagent_table_path = nse_dragonfly_to_reagent_table(template_file_path, iteration, next_batch);\n\nreagent_table = ReagentTable();\nreagent_table.load_from_file(reagent_table_path);\nmaster_time_buffer = master_time + 200;\n\n[all_slugs] = nse_parse_initial_slugs_parallel_v7(reagent_table_path, N_reactors, enabled_reactors_list);\n[liquid_handler_start_times, loop_to_reactor_start_times, rinse_transfer_lines_start_times, reactor_to_analysis_start_times, rinse_reactor_start_times, analysis_start_times, reactors_start_times] = nse_scheduler_v4(all_slugs, 10, tau_prep, tau_loop_to_reactor, tau_rinse_vent_transfer_lines, tau_rinse_vent_reactor, tau_reactor_to_analysis, tau_analysis, master_time_buffer)\nloop_to_reactor_last_rxn = 0;\nrinse_transfer_lines_last_rxn = 0;\nrinse_reactor_last_rxn = 0;\nreactor_to_analysis_last_rxn = 0;\n\n% Define initial start times\nliquid_handler_next_start_time = liquid_handler_start_times(1);\nloop_to_reactor_next_start_time = loop_to_reactor_start_times(1);\nrinse_transfer_lines_next_start_time = rinse_transfer_lines_start_times(1);\nrinse_reactor_next_start_time = rinse_reactor_start_times(1);\nreactor_to_analysis_next_start_time = reactor_to_analysis_start_times(1);"("??"=w2176, "master_time"=w2212, "next_batch"=w2181) -> ("??"=w2179:errorcluster, "liquid_handler_start_times"=w2211:dbl[], "loop_to_reactor_start_times"=w2205:dbl[], "rinse_transfer_lines_start_times"=w2206:dbl[], "reactor_to_analysis_start_times"=w2207:dbl[], "rinse_reactor_start_times"=w2208:dbl[], "analysis_start_times"=w2209:dbl[], "reactors_start_times"=w2210:dbl[][], "liquid_handler_next_start_time"=w2204:dbl, "loop_to_reactor_next_start_time"=w2198:dbl, "rinse_transfer_lines_next_start_time"=w2197:dbl, "rinse_reactor_next_start_time"=w2196:dbl, "reactor_to_analysis_next_start_time"=w2195:dbl)
        n1706 = local write "Schedule - Liquid Handler"(w2211) -> ()
        n1707 = local write "Schedule - Liquid Handler to Reactor"(w2205) -> ()
        n1708 = local write "Schedule - Rinse Transfer Lines"(w2206) -> ()
        n1709 = local write "Schedule - Reactor to Analysis"(w2207) -> ()
        n1710 = local write "Schedule - Rinse Reactor"(w2208) -> ()
        n1711 = local write "Schedule - Analysis"(w2209) -> ()
        n1712 = local write "Schedule - Reactors"(w2210) -> ()
        n1713 = local write "Next start time - liquid handler"(w2204) -> ()
        n1714 = local write "Next start time - transport from loop to reactor"(w2198) -> ()
        n1715 = local write "Next start time - rinse transfer lines"(w2197) -> ()
        n1716 = local write "Next start time - rinse reactor"(w2196) -> ()
        n1717 = local write "Next start time - transport from reactor to analysis"(w2195) -> ()
        n1718 = call "Time Delay83"("error in (no error)"=w2179, "Delay Time (s)"=3.0) -> ("error out"=w2178:errorcluster)  [unwired: 9 in]
        n1719 = in-place {
          in-place-border: [w2221] -> w2203
          in-place-border: w2178 -> [w2221]
          w2219 = FALSE
          w2218 = FALSE
          n1720 = local read "Array 3"() -> (w2217:dbl[])
          n1721 = local write "liquid_handler_finished"(w2218) -> ()
          n1722 = local write "loop_to_reactor_finished"(w2218) -> ()
          n1723 = local write "rinse_transfer_lines_finished"(w2218) -> ()
          n1724 = local write "reactor_to_analysis_finished"(w2218) -> ()
          n1725 = local write "rinse_reactor_finished"(w2218) -> ()
          n1726 = local write "analysis_finished"(w2218) -> ()
          n1727 = local write "InitializationExp"(FALSE) -> ()
          n1728 = local write "Batch Results"(w2217) -> ()
          n1729 = local write "schedule_reset"(TRUE) -> ()
          n1730 = local write "r1_done"(w2219) -> ()
          n1731 = local write "r2_done"(w2219) -> ()
          n1732 = local write "r3_done"(w2219) -> ()
          n1733 = local write "r4_done"(w2219) -> ()
          n1734 = local write "r5_done"(w2219) -> ()
          n1735 = local write "r6_done"(w2219) -> ()
          n1736 = local write "r7_done"(w2219) -> ()
          n1737 = local write "r8_done"(w2219) -> ()
          n1738 = local write "r9_done"(w2219) -> ()
          n1739 = local write "r10_done"(w2219) -> ()
        }
        n1740 = local write "Reaction number - rinse reactor"(w2200) -> ()
        n1741 = local write "Reaction number - rinse transfer lines"(w2200) -> ()
        n1742 = local write "Reaction number - transport from reactor to analysis"(w2200) -> ()
        n1743 = local write "Reaction number - transport to reactor"(w2200) -> ()
        n1744 = call "Time Delay8"("error in (no error)"=w2203, "Delay Time (s)"=10.0) -> ("error out"=w2202:errorcluster)  [unwired: 9 in]
        n1745 = local write "Next analysis time"(1000000000000000.0) -> ()
        n1746 = in-place {
          in-place-border: w2202 -> [_]
          n1747 = local write "schedule_reset"(FALSE) -> ()
        }
      }
    }
    n1748 = call "Time Delay44"("error in (no error)"=w2149, "Delay Time (s)"=1.0) -> ("error out"=w2148:errorcluster)  [unwired: 9 in]
    n1749 = local read "Stop everything"() -> (w2171:bool)
  }
